vi "GUI2.vi"() -> ()   [LabVIEW 2023]
uses:
  <vilib>/userDefined/High Color/IMAQdx.ctl
  <vilib>/vision/Image Controls.llb/IMAQ Image.ctl
  <vilib>/vision/Avi.llb/IMAQ AVI2 Refnum.ctl
  Control2.ctl
  <vilib>/vision/driver/IMAQdx.llb/IMAQdx Acquisition Mode.ctl
  <vilib>/vision/driver/IMAQdx.llb/IMAQdx Buffer Number Mode.ctl
  <vilib>/Utility/error.llb/DialogType.ctl
  <vilib>/DAQmx/read.llb/DAQmx Read (Analog 1D Wfm NChan NSamp).vi
  <vilib>/DAQmx/write.llb/DAQmx Write (Analog 1D Wfm NChan NSamp).vi
  <extravilib>/ChannelInstances/Tag-bool/Read With Abort.vi
  <extravilib>/ChannelInstances/Stream-t'IMAQ Image.ctl'/Read With Abort.vi
  <extravilib>/ChannelInstances/Messenger-a[.](wfm(dbl))/Read With Abort.vi
  <extravilib>/ChannelInstances/Tag-str/Write With Abort.vi
  <extravilib>/ChannelInstances/Tag-c(bool,i32,str)/Read With Abort.vi
  <extravilib>/ChannelInstances/Messenger-c(bool,i32,str)/Write With Abort.vi
  <extravilib>/ChannelInstances/Messenger-a[.](wfm(dbl))/Write With Abort.vi
  <extravilib>/ChannelInstances/Messenger-c(bool,bool,bool,str,t'Rendezvous RefNum',bool)/Read With Abort.vi
  <extravilib>/ChannelInstances/Messenger-c(c(,,,bool),c(u16[NoSync,Sync],dbl,dbl,i32),str,ref(UserDefinedRefnumTag),c(path,str,u16[TDMS,CSV],str,bool))/Read With Abort.vi
  <extravilib>/ChannelInstances/Tag-bool/Write With Abort.vi
  <extravilib>/ChannelInstances/Messenger-c(bool,bool,bool,bool,t'Rendezvous RefNum',bool)/Write With Abort.vi
  <extravilib>/ChannelInstances/Messenger-c(c(str,i64,i64,str,str,t'IMAQdx.ctl'),c(i32,dbl,,,,str),c(dbl,str,str),c(i32,i32),i32,c(path,str,str,str,i32,str,i32,str))/Write With Abort.vi
  <extravilib>/ChannelInstances/Messenger-c(c(,,,bool),c(i32,i32,i32),str,c(path,str,u16[TDMS,CSV],str,bool))/Write With Abort.vi
  <extravilib>/ChannelInstances/Messenger-c(a[.](c(dbl,stamp,dbl)),bool,bool,bool,str,t'Rendezvous RefNum',bool)/Write With Abort.vi
  <extravilib>/ChannelInstances/Messenger-c(c(,,,bool),c(u16[NoSync,Sync],dbl,dbl,i32),str,ref(UserDefinedRefnumTag),c(path,str,u16[TDMS,CSV],str,bool))/Write With Abort.vi
  <extravilib>/ChannelInstances/Messenger-c(bool,bool,bool,str,t'Rendezvous RefNum',bool)/Write With Abort.vi
  <extravilib>/ChannelInstances/Tag-str/Read With Abort.vi
  <vilib>/Utility/High Resolution Relative Seconds.vi
  <extravilib>/ChannelInstances/Messenger-c(a[.](c(dbl,stamp,dbl)),bool,bool,bool,str,t'Rendezvous RefNum',bool)/Read With Abort.vi
  <extravilib>/ChannelInstances/Messenger-c(c(,,,bool),c(i32,i32,i32),str,c(path,str,u16[TDMS,CSV],str,bool))/Read With Abort.vi
  <extravilib>/ChannelInstances/Messenger-c(bool,i32,str)/Read With Abort.vi
  <extravilib>/ChannelInstances/Tag-c(bool,i32,str)/Write With Abort.vi
  <extravilib>/ChannelInstances/Messenger-c(bool,bool,bool,bool,t'Rendezvous RefNum',bool)/Read With Abort.vi
  <extravilib>/ChannelInstances/Messenger-c(c(str,i64,i64,str,str,t'IMAQdx.ctl'),c(i32,dbl,,,,str),c(dbl,str,str),c(i32,i32),i32,c(path,str,str,str,i32,str,i32,str))/Read With Abort.vi
  <extravilib>/ChannelInstances/Stream-t'IMAQ Image.ctl'/Write With Abort.vi
  <extravilib>/ChannelInstances/Stream-t'IMAQ Image.ctl'/EndpointRead.vi
  <extravilib>/ChannelInstances/Stream-t'IMAQ Image.ctl'/Endpoint.vi
  <extravilib>/ChannelInstances/Tag-bool/Instantiate.vi
  <extravilib>/ChannelInstances/Messenger-a[.](wfm(dbl))/Instantiate.vi
  <extravilib>/ChannelInstances/Messenger-c(bool,i32,str)/Instantiate.vi
  <vilib>/Utility/file.llb/Read Delimited Spreadsheet (DBL).vi
  TDMS File Initialization (Read).vi
  <vilib>/Utility/error.llb/Error Cluster From Error Code.vi
  <extravilib>/ChannelInstances/Tag-bool/EndpointRead.vi
  <extravilib>/ChannelInstances/Messenger-a[.](wfm(dbl))/Endpoint.vi
  <extravilib>/ChannelInstances/Tag-str/Instantiate.vi
  <extravilib>/ChannelInstances/Messenger-c(bool,bool,bool,str,t'Rendezvous RefNum',bool)/Instantiate.vi
  <extravilib>/ChannelInstances/Messenger-c(c(,,,bool),c(u16[NoSync,Sync],dbl,dbl,i32),str,ref(UserDefinedRefnumTag),c(path,str,u16[TDMS,CSV],str,bool))/Instantiate.vi
  <extravilib>/ChannelInstances/Messenger-c(a[.](c(dbl,stamp,dbl)),bool,bool,bool,str,t'Rendezvous RefNum',bool)/Instantiate.vi
  <extravilib>/ChannelInstances/Messenger-c(c(,,,bool),c(i32,i32,i32),str,c(path,str,u16[TDMS,CSV],str,bool))/Instantiate.vi
  <extravilib>/ChannelInstances/Messenger-c(bool,bool,bool,bool,t'Rendezvous RefNum',bool)/Instantiate.vi
  <extravilib>/ChannelInstances/Messenger-c(c(str,i64,i64,str,str,t'IMAQdx.ctl'),c(i32,dbl,,,,str),c(dbl,str,str),c(i32,i32),i32,c(path,str,str,str,i32,str,i32,str))/Instantiate.vi
  <extravilib>/ChannelInstances/Tag-bool/Endpoint.vi
  <extravilib>/ChannelInstances/Messenger-c(bool,bool,bool,bool,t'Rendezvous RefNum',bool)/Endpoint.vi
  <extravilib>/ChannelInstances/Messenger-c(c(str,i64,i64,str,str,t'IMAQdx.ctl'),c(i32,dbl,,,,str),c(dbl,str,str),c(i32,i32),i32,c(path,str,str,str,i32,str,i32,str))/Endpoint.vi
  <extravilib>/ChannelInstances/Messenger-c(c(,,,bool),c(i32,i32,i32),str,c(path,str,u16[TDMS,CSV],str,bool))/Endpoint.vi
  <extravilib>/ChannelInstances/Messenger-c(a[.](c(dbl,stamp,dbl)),bool,bool,bool,str,t'Rendezvous RefNum',bool)/Endpoint.vi
  <extravilib>/ChannelInstances/Messenger-c(c(,,,bool),c(u16[NoSync,Sync],dbl,dbl,i32),str,ref(UserDefinedRefnumTag),c(path,str,u16[TDMS,CSV],str,bool))/Endpoint.vi
  <extravilib>/ChannelInstances/Messenger-c(bool,bool,bool,str,t'Rendezvous RefNum',bool)/Endpoint.vi
  <extravilib>/ChannelInstances/Tag-str/EndpointRead.vi
  <extravilib>/ChannelInstances/Messenger-c(bool,i32,str)/Endpoint.vi
  <extravilib>/ChannelInstances/Tag-c(bool,i32,str)/Instantiate.vi
  <extravilib>/ChannelInstances/Tag-str/Endpoint.vi
  <vilib>/DAQmx/create/channels.llb/DAQmx Create Channel (AO-Voltage-Basic).vi
  <vilib>/DAQmx/configure/timing.llb/DAQmx Timing (Sample Clock).vi
  <vilib>/DAQmx/configure/trigger.llb/DAQmx Start Trigger (Digital Edge).vi
  <vilib>/Waveform/WDTFileIO.llb/Export Waveforms To Spreadsheet File (1D).vi
  <vilib>/DAQmx/miscellaneous.llb/DAQmx Fill In Error Info.vi
  <extravilib>/ChannelInstances/Tag-c(bool,i32,str)/EndpointRead.vi
  <vilib>/DAQmx/create/channels.llb/DAQmx Create Channel (AI-Voltage-Basic).vi
  <extravilib>/ChannelInstances/Tag-c(bool,i32,str)/Endpoint.vi
  <extravilib>/ChannelInstances/Stream-t'IMAQ Image.ctl'/Instantiate.vi
  <extravilib>/ChannelInstances/Stream-t'IMAQ Image.ctl'/)Channel.vi
  <resource>/ChannelSupport/_ChannelSupport/WaitIfNeeded.vi
  <vilib>/vision/EDVR.llb/IMAQ ImageToEDVR.vi
  <vilib>/vision/EDVR.llb/IMAQ ImageToEDVR 1D U8.vi
  <vilib>/vision/EDVR.llb/IMAQ ImageToEDVR 1D I16.vi
  <vilib>/vision/EDVR.llb/IMAQ ImageToEDVR 1D U32.vi
  <vilib>/vision/EDVR.llb/IMAQ ImageToEDVR 1D U16.vi
  <vilib>/Waveform/WDTOps.llb/WDT Append Waveforms DBL.vi
  <vilib>/Utility/file.llb/Write Delimited Spreadsheet (string).vi
  <vilib>/ErrorRing/Error Ring.xnode
  <vilib>/vision/driver/NI_Vision_Acquisition_Software.lvlib
  <resource>/objmgr/imaqdx.rc
  <extravilib>/ChannelInstances/Messenger-c(bool,i32,str).lvlib
  <extravilib>/ChannelInstances/Tag-c(bool,i32,str).lvlib
  <extravilib>/ChannelInstances/Tag-bool.lvlib
  <resource>/objmgr/daqmx.rc
  <extravilib>/ChannelInstances/Stream-t'IMAQ Image.ctl'.lvlib
  <extravilib>/ChannelInstances/Tag-str.lvlib
  <extravilib>/ChannelInstances/Messenger-c(bool,bool,bool,bool,t'Rendezvous RefNum',bool).lvlib
  <extravilib>/ChannelInstances/Messenger-c(a[.](c(dbl,stamp,dbl)),bool,bool,bool,str,t'Rendezvous RefNum',bool).lvlib
  <extravilib>/ChannelInstances/Messenger-c(bool,bool,bool,str,t'Rendezvous RefNum',bool).lvlib
  <extravilib>/ChannelInstances/Messenger-a[.](wfm(dbl)).lvlib
  <extravilib>/ChannelInstances/Messenger-c(c(,,,bool),c(i32,i32,i32),str,c(path,str,u16[TDMS,CSV],str,bool)).lvlib
  <extravilib>/ChannelInstances/Messenger-c(c(,,,bool),c(u16[NoSync,Sync],dbl,dbl,i32),str,ref(UserDefinedRefnumTag),c(path,str,u16[TDMS,CSV],str,bool)).lvlib
  <extravilib>/ChannelInstances/Messenger-c(c(str,i64,i64,str,str,t'IMAQdx.ctl'),c(i32,dbl,,,,str),c(dbl,str,str),c(i32,i32),i32,c(path,str,str,str,i32,str,i32,str)).lvlib
  <vilib>/measure/NI_MABase.lvlib
panel:
  out "Sensor Readout Time":dbl
  out "Max FPS":dbl
  out "FPS":dbl
  out "Images Behind":dbl
  out "Missed Images":dbl
  out "Video Bytes/s":dbl
  out "Estimated Time":dbl
  out "FPS 2":dbl
  out "Images Behind 2":dbl
  out "Missed Images 2":dbl
  out "Estimated Time 2":dbl
  out "Array 2":string[](array[string])
  out "Array":string[](array[string])
  in  "CameraPane Selector":u16(ring) items=["None", "CameraDisplay", "Plot1", "Plot2", "Plot3", "Plot4", "XY1", "XY2"]
  in  "Experiment Name":string="VoltageTest"
  in  "Save Path":path
  in  "Save Config":bool
  in  "Apply Configuration":bool
  in  "Config Path":path
  in  "Initialize from config file?":bool caption="Checkbox"
  in  "Quit":bool
  in  "Controls":bool
  in  "File Manager":bool
  in  "Settings":bool
  in  "Camera Setup":bool
  in  "MainTabControl":T1(tab)
  in  "Stop Square":bool
  in  "Initialize Camera":bool
  in  "Cluster - Borderless":T3={"Cluster - Borderless"={"Time Stamp\n Position"=enum."Exposure Center", "Synchronize Camera and Data"=TRUE}, "Sensor readout mode\n(Fast Decreases Quality)"=0, "Pixel Format\n(p not supported)"=0, "Gain"=0.0, "Gamma"=1.0, "Temporary Format\n(can be converted)"=enum."AVI", "Cluster - Borderless 2"={"Frame Limit"=0.0}, "Cluster - Borderless 3"={"Frame Limit"=0.0}, "Camera Ref"="", "Tempory Storage Location\n(File can be moved after acquisition)\nSSD recomended for high frame rate"=path "E:/Jacob", "Images Per File"=1000000.0, "Buffer Images"=1000.0, "Exposure (us)"=100.0, "FPS"=30.0, "Encoding Quality"=-1.0, "Image Width"=0.0, "Image Height"=0.0, "Signal Line"=2, "Codec"=2, "Confirm File Write Optimizations (TDMS)"=TRUE, "Confirm Disable Buffering (advanced TDMS)"=FALSE, "Camera Signal Output Port"="/Dev1/PFI2", "Exposure Mode"=0, "Video File Suffix"="Video", "Timing File Suffix"="VideoTime", "Include Camera Signal Output File"=FALSE, "File Time Resolution (s)"=0.0, "Stop Acquisition on Full Buffer"=TRUE} {"Exposure Mode" items=["Standard", "Ultra Short"]; "Codec" items=["(Select at runtime)", "YUV 4:2:0 Planar (NI Vision)", "Y800 Uncompressed Grey Scale (NI Vision)", "VP9 (NI Vision)", "Motion JPEG (NI Vision)", "FF Video Codec 1 (FFV1) (NI Vision)", "VP8 (NI Vision)"]; "Signal Line" items=["Software", "Line 1", "Line 3", "Line 4", "Software Signal 1", "Software Signal 2", "Software Signal 3"]; "Gamma" min=0.0 max=4.0 step=1.0 scale=0.0..3.0; "Gain" min=0.0 max=12.0092 step=1.0 scale=0.0..12.0; "Pixel Format\n(p not supported)" items=["Mono 8", "Mono 10"]; "Sensor readout mode\n(Fast Decreases Quality)" items=["Normal", "Fast"]}
  in  "Stop Acquisition On Full Hard Drive":bool=TRUE caption="Checkbox"
  in  "XY2 Y":u16(ring) items=["None", "Current (mA)", "Voltage (V)"]
  in  "XY2 X":u16(ring) items=["None", "Current (mA)", "Voltage (V)"]
  in  "XY1 Y":u16(ring) items=["None", "Current (mA)", "Voltage (V)"]
  in  "XY1 X":u16(ring) items=["None", "Current (mA)", "Voltage (V)"]
  in  "Data File Settings":T4={"Data File Format"=FALSE, "Data Temporary Storage Location"=path "E:/Jacob", "Temporary Location"=TRUE, "Input Data File Suffix"="Data", "Output Data File Suffix"="DataOutput", "              CSV\nMultiple Time Columns"=FALSE}
  in  "Plot 4 Channels":i32[](listbox)
  in  "Plot 3 Channels":i32[](listbox)
  in  "Plot 2 Channels":i32[](listbox)
  in  "Plot 1 Channels":i32[](listbox)
  in  "Samples to Generate":dbl=1000.0
  out "1D Array":string[](array[string])
  in  "Channel Names":string[](array[string])
  in  "Sample Buffer":dbl=1000.0
  in  "Sample Rate":dbl=10000.0
  in  "Input Channels":tag
  in  "Voltage Input Channel":tag
  in  "Current Input Channel":tag
  in  "Using Gamry Potentiostat":bool caption="Checkbox"
  in  "Recipients":string
  in  "Send email on non-user-initiated stop":bool
  out "Shutting\nDown":bool
  out "Video Space Remaining (min)":dbl
  out "Data Space Remaining (min)":dbl
  out "Video Buffer Fill Percent":dbl(slide) scale=0.0..100.0
  in  "Stop Button":bool
  in  "Use Camera":bool
  in  "FPS":dbl=150.0
  in  "Save Video":bool
  in  "Initialize Camera":bool
  in  "Outputs":T5={"AO0"={"signal type"=enum."Sine Wave", "Frequency"=0.0, "Amplitude"=0.0, "Offset"=0.0, "Phase"=0.0, "Duty Cycle"=0.0}, "AO0Enable"=FALSE, "AO1"={"signal type"=enum."Sine Wave", "Frequency"=0.0, "Amplitude"=0.0, "Offset"=0.0, "Phase"=0.0, "Duty Cycle"=0.0}, "AO1Enable"=FALSE, "AO2"={"signal type"=enum."Sine Wave", "Frequency"=0.0, "Amplitude"=0.0, "Offset"=0.0, "Phase"=0.0, "Duty Cycle"=0.0}, "AO3Enable"=FALSE, "AO0Name"="Ao0", "AO1Name"="Ao1", "AO2Name"="Ao2"}
  in  "Re/Start Acquisition":bool
  in  "Exposure (us)":dbl
  in  "Update Viewport Every N Frames":dbl=1.0
  in  "PlotSelector":T6(tab)
  in  "OneSelection":u16(ring) items=["None", "CameraDisplay", "Plot1", "Plot2", "Plot3", "Plot4", "XY1", "XY2"]
  in  "TwoVertSelL":u16(ring) items=["None", "CameraDisplay", "Plot1", "Plot2", "Plot3", "Plot4", "XY1", "XY2"]
  in  "TwoVertSelR":u16(ring) items=["None", "CameraDisplay", "Plot1", "Plot2", "Plot3", "Plot4", "XY1", "XY2"]
  in  "2HorizSelB":u16(ring) items=["None", "CameraDisplay", "Plot1", "Plot2", "Plot3", "Plot4", "XY1", "XY2"]
  in  "2HorizSelT":u16(ring) items=["None", "CameraDisplay", "Plot1", "Plot2", "Plot3", "Plot4", "XY1", "XY2"]
  in  "3PaneVertSelBR":u16(ring) items=["None", "CameraDisplay", "Plot1", "Plot2", "Plot3", "Plot4", "XY1", "XY2"]
  in  "3PaneVertSelTR":u16(ring) items=["None", "CameraDisplay", "Plot1", "Plot2", "Plot3", "Plot4", "XY1", "XY2"]
  in  "3PaneVertSelL":u16(ring) items=["None", "CameraDisplay", "Plot1", "Plot2", "Plot3", "Plot4", "XY1", "XY2"]
  in  "3PaneHorizBL":u16(ring) items=["None", "CameraDisplay", "Plot1", "Plot2", "Plot3", "Plot4", "XY1", "XY2"]
  in  "3PaneHorizBR":u16(ring) items=["None", "CameraDisplay", "Plot1", "Plot2", "Plot3", "Plot4", "XY1", "XY2"]
  in  "3PaneHorizT":u16(ring) items=["None", "CameraDisplay", "Plot1", "Plot2", "Plot3", "Plot4", "XY1", "XY2"]
  in  "4PaneSelBR":u16(ring) items=["None", "CameraDisplay", "Plot1", "Plot2", "Plot3", "Plot4", "XY1", "XY2"]
  in  "4PaneSelBL":u16(ring) items=["None", "CameraDisplay", "Plot1", "Plot2", "Plot3", "Plot4", "XY1", "XY2"]
  in  "4PaneSelTR":u16(ring) items=["None", "CameraDisplay", "Plot1", "Plot2", "Plot3", "Plot4", "XY1", "XY2"]
  in  "4PaneSelTL":u16(ring) items=["None", "CameraDisplay", "Plot1", "Plot2", "Plot3", "Plot4", "XY1", "XY2"]
  out "Plot Overflow":i32
  out "Actual Sample Rate":dbl
  out "Images Missed":u32
  out "Processing Speed (ms)":dbl format="%_19f"
  out "Write Speed (ms)":dbl format="%_19f"
  out "BufferWasFull":bool
  out "Files Complete":i32(slide)=1 max=4 scale=0.0..4.0
  in  "Start Button":bool
  in  "Codec":u16(ring)=2 items=["(Select at runtime)", "YUV 4:2:0 Planar (NI Vision)", "Y800 Uncompressed Grey Scale (NI Vision)", "VP9 (NI Vision)", "Motion JPEG (NI Vision)", "FF Video Codec 1 (FFV1) (NI Vision)", "VP8 (NI Vision)"]
  in  "Quality":dbl=-1.0
  in  "Same as previous":bool=TRUE caption="Checkbox"
  in  "Timing File":path=path "E:/Jacob"
  in  "AVI FPS":dbl=30.0
  in  "Same as acquisition":bool caption="Checkbox"
  in  "Save Name":string
  in  "Save Path":path=path "E:/Jacob"
  in  "Combine Split Videos":bool caption="Checkbox"
  in  "First Video File":path=path "E:/Jacob"
  in  "Current Image Type":u16(ring) items=["Grayscale (U8)"=0, "Grayscale (I16)"=1, "Grayscale (U16)"=7, "RGB Color (U32)"=4]
  in  "Stop Conversion":bool
  out "File Percent Done":dbl(slide) scale=0.0..1.0
  # "Basic Camera Controls"
  # "Camera"
  # "Image Aquisition Settings"
  # "Video File Settings"
  # "Do not use \"_\""
  # "This may cause memory issues"
  # "Advanced Settings"
  # "Advanced File Settings"
  # "(Must be multiple of 64)"
  # "AVI Settings"
  # "If very high framerates are required, save to TDMS not AVI\nFor high framerates Y800 is recomended, but requires\ncompression later to save space\nFor lower framerates, Motion JPEG saves \nspace and conversion time"
  # "For further advanced setting changes (binning,\netc.) open NI Max, select the camera, and change\nthe desired properties, pressing save at the end.\n\n(Note: This program may overwrite settings\ntemporarily while running in order to function)"
  # "(1-1000) or -1 for highest"
  # "Hardware Triggered\nAcquisition Settings"
  # "Use shift or ctrl to select multiple channels for each plot"
  # "XY Plots not yet implemented"
  # "If the data generation estimate does not line up with the measured value, consider increasing the buffer,\nthis allows software processing without interupting sample generation/aquisition.\nIt is highly recomended to measure the generated output instead of relying on just the estimate, since there might be\nartifacts generated by processing, especially near the beginning.\nHaving too small a buffer compared to samples to generate \ncan cause blips in the signal generation when interacting with the software. Leaving a sufficient number of ms\nfor software to work is recomended.\nIf working with an important experiment, it is recomended to minimize interaction to ensure sample generation\nis what is desired.\n\nIf the plot update is too slugish, consider decreasing the buffer.\nHowever, decreasing the buffer decreases ability of plot to keep up with supplied data."
  # "This should be lower than the sample rate"
  # "(Output Only)"
  # "This should be at least 2x higher than the sample buffer"
  # "TDMS may be faster (Can be converted later)"
  # "Writing to CSV can be very slow \nuse only for small data rates with minimal channels\n\nIf time accuracy is required within 10 us, \nuse multiple time columns"
  # "(Needs Reset)"
  # "Does not save video"
  # "TDMS Video Conversion"
  # "Requires timing file"
  # "(1-1000) or -1 for highest"
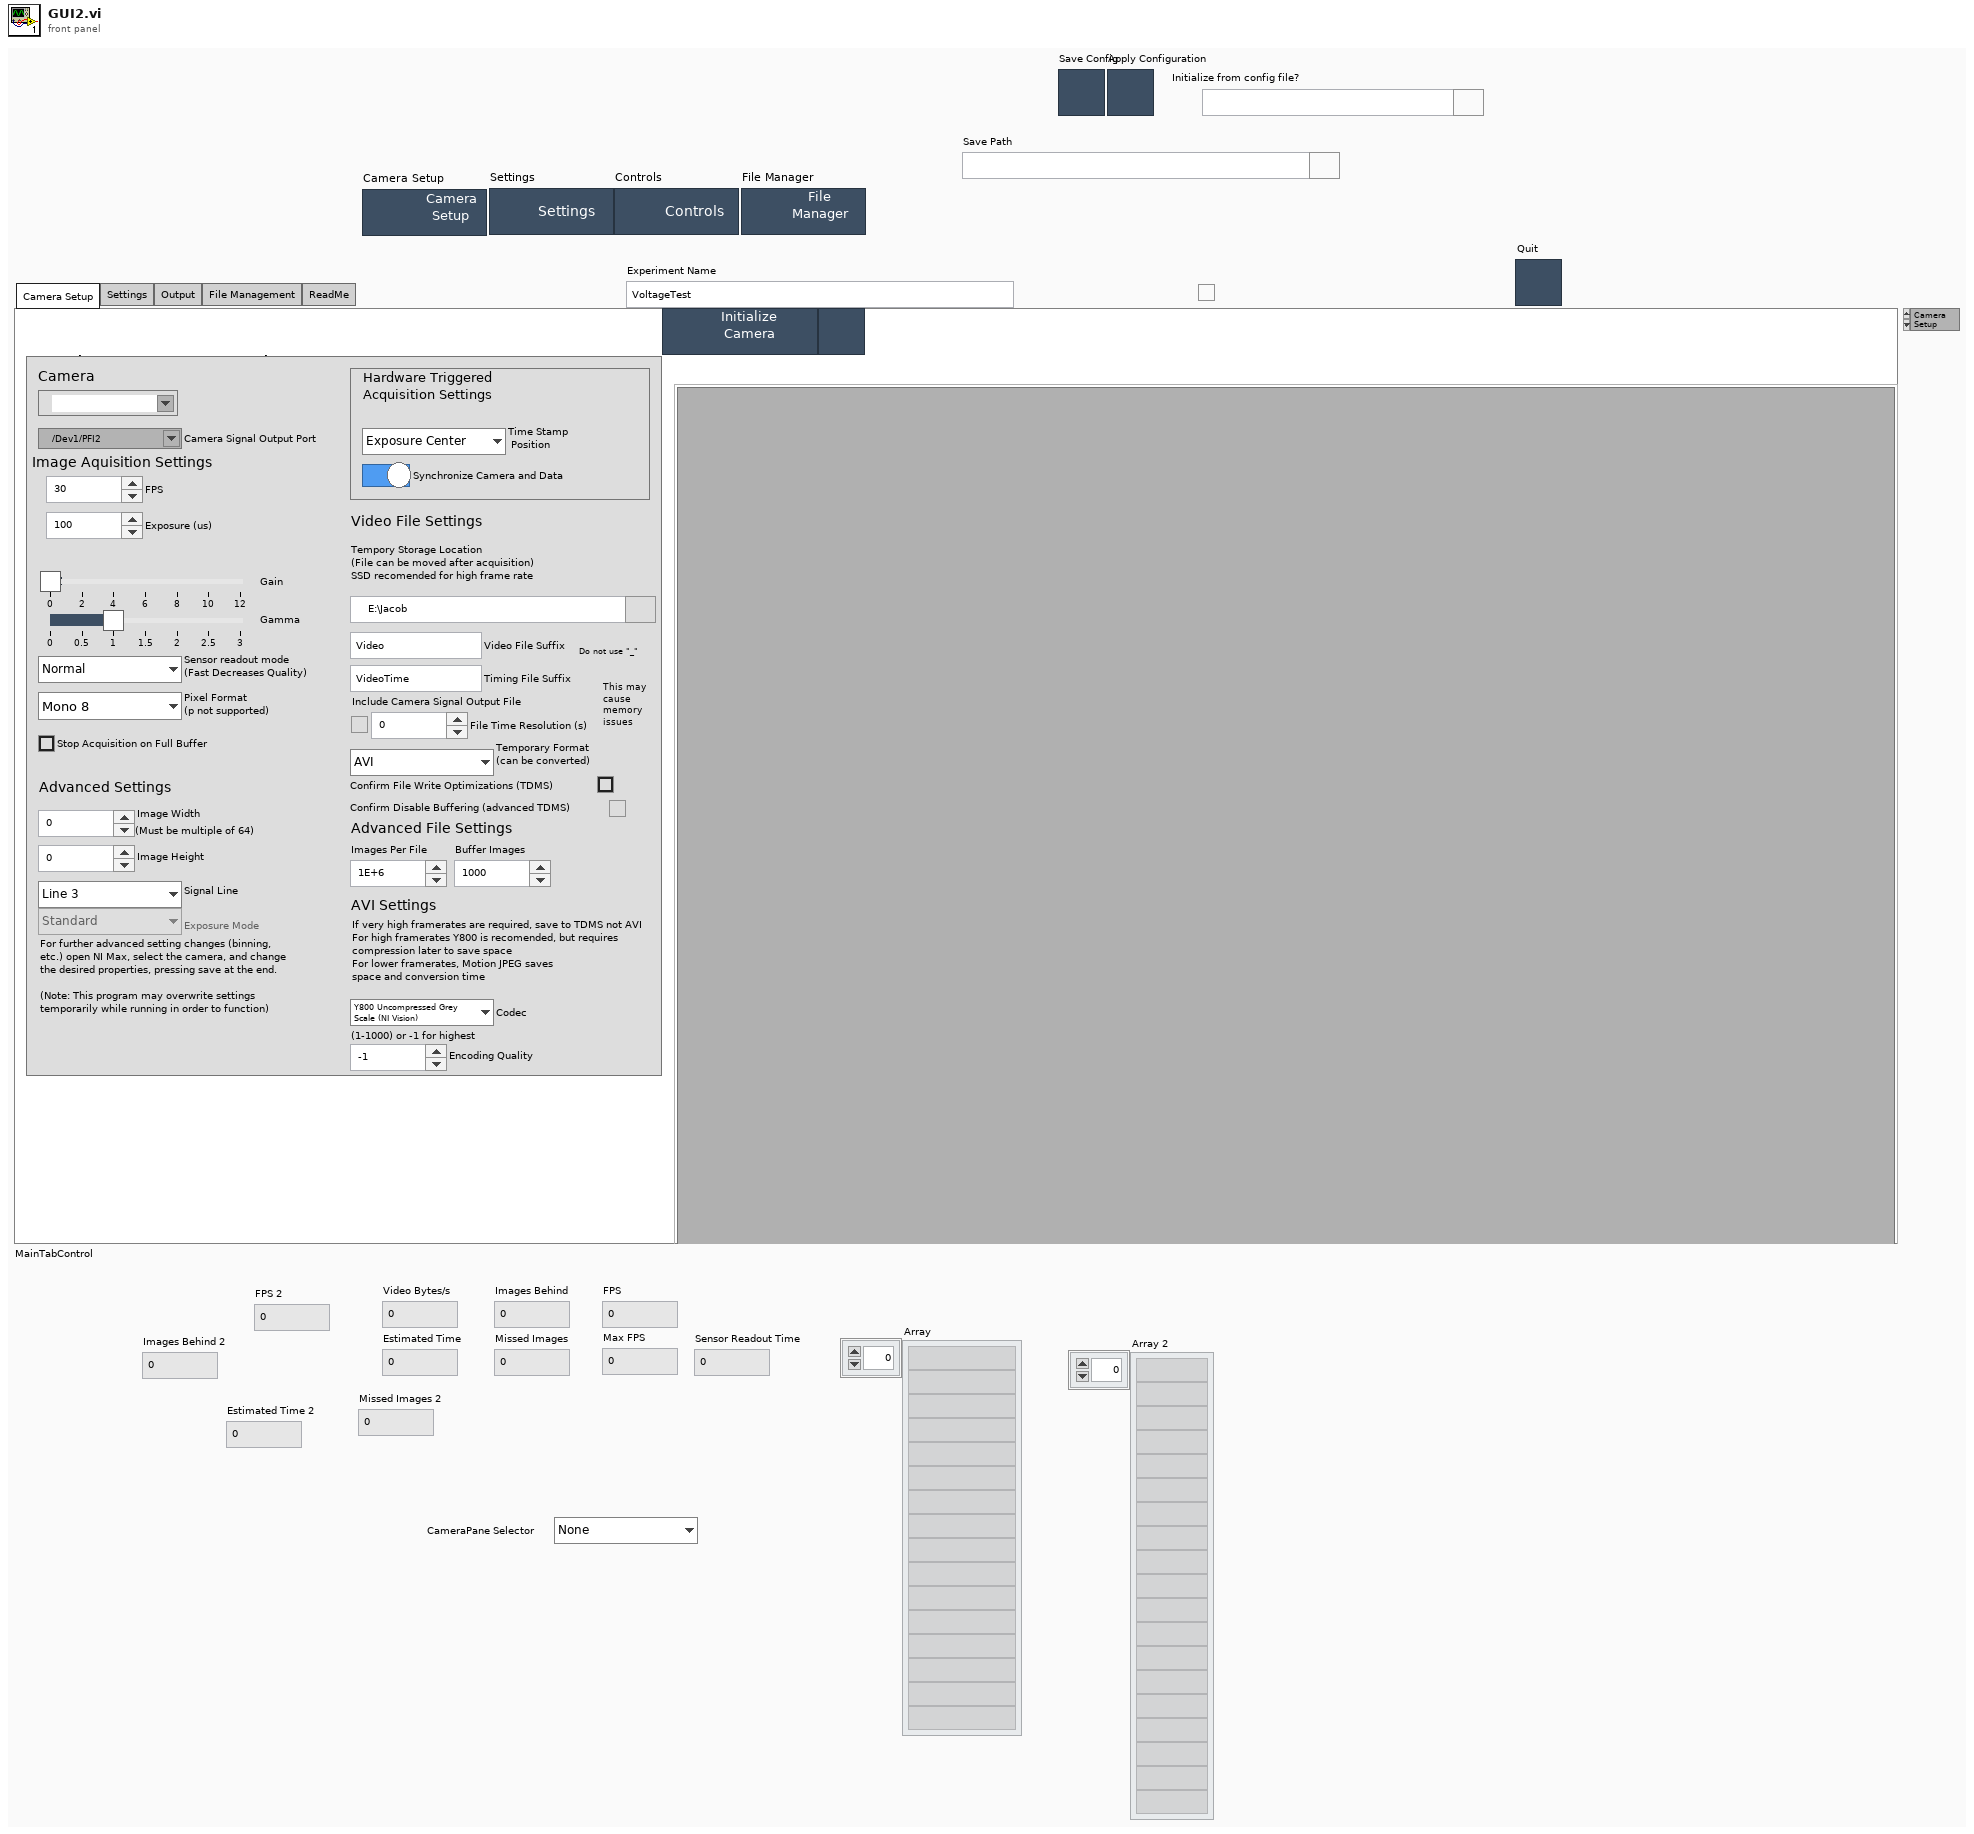
[diagram p1: front panel]
types:
  T1 = enum32{"Camera Setup", "Settings", "Output", "File Management", "ReadMe"}
  T2 = typedef "IMAQdx.ctl" = refnum<k21>
  T3 = cluster{"Cluster - Borderless":cluster{"Time Stamp\n Position":enum16{"Exposure Center", "Exposure Beginning", "Exposure End"}, "Synchronize Camera and Data":bool}, "Sensor readout mode\n(Fast Decreases Quality)":u16, "Pixel Format\n(p not supported)":u16, "Gain":dbl, "Gamma":dbl, "Temporary Format\n(can be converted)":enum16{"AVI", "TDMS", "None"}, "Cluster - Borderless 2":cluster{"Frame Limit":dbl}, "Cluster - Borderless 3":cluster{"Frame Limit":dbl}, "Camera Ref":T2, "Tempory Storage Location\n(File can be moved after acquisition)\nSSD recomended for high frame rate":path, "Images Per File":dbl, "Buffer Images":dbl, "Exposure (us)":dbl, "FPS":dbl, "Encoding Quality":dbl, "Image Width":dbl, "Image Height":dbl, "Signal Line":u16, "Codec":u16, "Confirm File Write Optimizations (TDMS)":bool, "Confirm Disable Buffering (advanced TDMS)":bool, "Camera Signal Output Port":tag, "Exposure Mode":u16, "Video File Suffix":string, "Timing File Suffix":string, "Include Camera Signal Output File":bool, "File Time Resolution (s)":dbl, "Stop Acquisition on Full Buffer":bool}
  T4 = cluster{"Data File Format":bool, "Data Temporary Storage Location":path, "Temporary Location":bool, "Input Data File Suffix":string, "Output Data File Suffix":string, "              CSV\nMultiple Time Columns":bool}
  T5 = cluster{"AO0":cluster{"signal type":enum16{"Sine Wave", "Triangle Wave", "Square Wave", "Sawtooth Wave"}, "Frequency":dbl, "Amplitude":dbl, "Offset":dbl, "Phase":dbl, "Duty Cycle":dbl}, "AO0Enable":bool, "AO1":cluster{"signal type":enum16{"Sine Wave", "Triangle Wave", "Square Wave", "Sawtooth Wave"}, "Frequency":dbl, "Amplitude":dbl, "Offset":dbl, "Phase":dbl, "Duty Cycle":dbl}, "AO1Enable":bool, "AO2":cluster{"signal type":enum16{"Sine Wave", "Triangle Wave", "Square Wave", "Sawtooth Wave"}, "Frequency":dbl, "Amplitude":dbl, "Offset":dbl, "Phase":dbl, "Duty Cycle":dbl}, "AO3Enable":bool, "AO0Name":string, "AO1Name":string, "AO2Name":string}
  T6 = enum32{"One Pane", "2 Vertical Panes", "2 Horizontal Panes", "3 Panes Vert", "3 Panes Horiz", "Four Panes"}
  T7 = typedef "Rendezvous RefNum" = refnum<k1>
  T8 = cluster{"Use Camera":bool, "Use Inputs":bool, "Use Outputs":bool, "rendezvous":T7, "Save Video":bool, "VideoPath":path, "DataPath":path, "Acquiring":bool, "LastSizeVid":dbl, "Last Time":dbl, "LastSizeData":dbl, "StopMessage":string, "Description":string, "Post Notes":string, "StopDueToError":bool}
  T9 = cluster{"SyncStart":bool, "Leader":bool, "Started?":bool, "AfterErrorCheck":string, "rendezvous ref":T7, "AcStarted":bool, "FirstAq":bool, "t0":timestamp, "TDMSRef":refnum<k34>, "CSV path":path}
  T10 = cluster{"Physical Settings":cluster{"physical channels":tag, "source":tag, "Start Trigger":tag, "StartTriggered":bool}, "Acquisition Settings":cluster{"SyncType":enum16{"NoSync", "Sync"}, "Frame Rate":dbl, "Sample Rate":dbl, "Sample BufferSize":i32}, "Channel Names":string, "task in":refnum<k21>, "FileSettings":cluster{"Path":path, "File":string, "FileFormat":enum16{"TDMS", "CSV"}, "FileSuffix":string, "Multiple Time Columns":bool}}
  T11 = cluster{"DefaultAction":string, "NextAction":string, "ActionString":string}
  T12 = typedef "Control2.ctl" = cluster{"SubPanel":refnum<vi>, "Selector":refnum<vi>}
  T13 = cluster{"One Pane":cluster{"Panel2":cluster{"SubPanel":refnum<vi>, "Selector":refnum<vi>}, "Panel3":cluster{"SubPanel":refnum<vi>, "Selector":refnum<vi>}, "Panel4":cluster{"SubPanel":refnum<vi>, "Selector":refnum<vi>}, "Panel1":T12}, "2 Vertical Panes":cluster{"Panel2":cluster{"SubPanel":refnum<vi>, "Selector":refnum<vi>}, "Panel3":cluster{"SubPanel":refnum<vi>, "Selector":refnum<vi>}, "Panel4":cluster{"SubPanel":refnum<vi>, "Selector":refnum<vi>}, "Panel1":T12}, "2 Horizontal Panes":cluster{"Panel2":cluster{"SubPanel":refnum<vi>, "Selector":refnum<vi>}, "Panel3":cluster{"SubPanel":refnum<vi>, "Selector":refnum<vi>}, "Panel4":cluster{"SubPanel":refnum<vi>, "Selector":refnum<vi>}, "Panel1":T12}, "3 Panes Vert":cluster{"Panel2":cluster{"SubPanel":refnum<vi>, "Selector":refnum<vi>}, "Panel3":cluster{"SubPanel":refnum<vi>, "Selector":refnum<vi>}, "Panel4":cluster{"SubPanel":refnum<vi>, "Selector":refnum<vi>}, "Panel1":T12}, "3 Panes Horiz":cluster{"Panel2":cluster{"SubPanel":refnum<vi>, "Selector":refnum<vi>}, "Panel3":cluster{"SubPanel":refnum<vi>, "Selector":refnum<vi>}, "Panel4":cluster{"SubPanel":refnum<vi>, "Selector":refnum<vi>}, "Panel1":T12}, "Four Panes":cluster{"Panel2":cluster{"SubPanel":refnum<vi>, "Selector":refnum<vi>}, "Panel3":cluster{"SubPanel":refnum<vi>, "Selector":refnum<vi>}, "Panel4":cluster{"SubPanel":refnum<vi>, "Selector":refnum<vi>}, "Panel1":T12}, "Camera Pane":cluster{"Panel2":cluster{"SubPanel":refnum<vi>, "Selector":refnum<vi>}, "Panel3":cluster{"SubPanel":refnum<vi>, "Selector":refnum<vi>}, "Panel4":cluster{"SubPanel":refnum<vi>, "Selector":refnum<vi>}, "Panel1":T12}}
  T14 = cluster{"Panel2":cluster{"SubPanel":refnum<vi>, "Selector":refnum<vi>}, "Panel3":cluster{"SubPanel":refnum<vi>, "Selector":refnum<vi>}, "Panel4":cluster{"SubPanel":refnum<vi>, "Selector":refnum<vi>}, "Panel1":T12}
  T15 = cluster{"PreviousInfo":cluster{"FinalSamplePhase":dbl, "LastTf":timestamp, "LastSelectedPhase":dbl}[], "SyncStart":bool, "Leader":bool, "Started?":bool, "AfterErrorCheck":string, "rendezvous ref ":T7, "AcStarted":bool, "PrevousWave":waveform(dbl)[], "TDMSRef":refnum<k34>, "CSV path":path}
  T16 = cluster{"Physical Settings":cluster{"physical channels":tag, "source":tag, "Start Trigger":tag, "StartTriggered":bool}, "OutputTask":refnum<k21>, "GenerationSettings":cluster{"NumberOfSamples":i32, "Sample Rate":i32, "SampleBuffer":i32}, "Channel Names":string, "FileSettings":cluster{"Path":path, "File":string, "FileFormat":enum16{"TDMS", "CSV"}, "FileSuffix":string, "Multiple Time Columns":bool}}
  T17 = cluster{"SyncStart":bool, "AfterErrorCheck":string, "VideoPath":path, "ConfirmTDMSOptimizations":bool, "ConfirmTDMSDisableBuffer":bool, "CameraOpen":bool, "TriggerStarted":bool, "AcquisitionStarted":bool, "FileOpen":bool, "VideoSave":bool, "BufferOpen":bool, "ShutdownActions":string[], "Acquisition Configured":bool, "rendezvous ref ":T7, "ResetAq?":bool, "AcStarted":bool, "Frames":i32}
  T18 = typedef "IMAQ Image.ctl" = refnum<image>
  T19 = typedef "IMAQ AVI2 Refnum.ctl" = refnum<k20>
  T20 = typedef "Image Type" = u32
  T21 = cluster{"User Camera Settings":cluster{"Pixel Format":string, "Width":i64, "Height":i64, "Trigger Source":string, "Readout Mode":string, "Session In":T2}, "IMAQdx Session":T2, "Camera Aq Attributes":cluster{"Readout Time":dbl, "Resulting FPS":dbl, "Width":u32, "Height":u32, "Format":u32, "Bit Depth":u32}, "Camera Attributes":cluster{"Exposure Start Delay":dbl, "Model":string, "Make":string}, "AcquisitionSettings":cluster{"Buffer":i32, "FramesPerFile":i32}, "Image Buffer":T18[], "Example Image":T18, "AVIRef":T19, "TDMSRef":refnum<k34>, "TDMSWSet":cluster{"Image Type":T20, "Async File Format":bool}, "CameraSignalRefnum":refnum<k21>, "CameraSignalDefinition":cluster{"High Time":dbl, "Low Time":dbl, "Delay":dbl}, "DisplayEveryNFrames":i32, "Trigger Settings":cluster{"FPS":i32, "Exposure Time":dbl, "Start Trigger Source":tag, "Camera\nClock\nCounter":tag, "PhysicalCameraSignalLine":tag, "Sync Type":string}, "FileSettings":cluster{"FileSaveLocation":path, "FileName":string, "VideoSuffix":string, "Codec":string, "Quality":i32, "Format":string, "AVI FPS":i32, "TimingSuffix":string}}
  T22 = enum8{"Enabled", "Disabled", "Disabled and Grayed Out"}
  T23 = enum16{"open", "replace", "create", "open or create", "replace or create", "replace or create with confirmation"}
  T24 = cluster{"User Camera Settings":cluster{"Pixel Format":string, "Width":i64, "Height":i64, "Trigger Source":string, "Readout Mode":string, "Session In":T2}, "Trigger Settings":cluster{"FPS":i32, "Exposure Time":dbl, "Start Trigger Source":tag, "Camera\nClock\nCounter":tag, "PhysicalCameraSignalLine":tag, "Sync Type":string}, "Camera Attributes":cluster{"Exposure Start Delay":dbl, "Model":string, "Make":string}, "AcquisitionSettings":cluster{"Buffer":i32, "FramesPerFile":i32}, "DisplayEveryNFrames":i32, "FileSettings":cluster{"FileSaveLocation":path, "FileName":string, "VideoSuffix":string, "Codec":string, "Quality":i32, "Format":string, "AVI FPS":i32, "TimingSuffix":string}}
  T25 = enum16{"Exposure End", "Exposure Center", "Exposure Start", "Start", "NoSync"}
  T26 = cluster{"Physical Settings":cluster{"physical channels":tag, "source":tag, "Start Trigger":tag, "StartTriggered":bool}, "GenerationSettings":cluster{"NumberOfSamples":i32, "Sample Rate":i32, "SampleBuffer":i32}, "Channel Names":string, "FileSettings":cluster{"Path":path, "File":string, "FileFormat":enum16{"TDMS", "CSV"}, "FileSuffix":string, "Multiple Time Columns":bool}}
  T27 = typedef "Tag-bool.lvlib/))Channel.ctl" = refnum<queue>
  T28 = cluster{"Panel2":cluster{"SubPanel":refnum<vi>, "Selector":refnum<vi>}, "Panel3":cluster{"SubPanel":refnum<vi>, "Selector":refnum<vi>}, "Panel4":cluster{"SubPanel":refnum<vi>, "Selector":refnum<vi>}, "Panel1":T12}[]
  T29 = cluster{"SubPanel":refnum<vi>, "Selector":refnum<vi>}
  T30 = cluster{"FPS":i32, "Exposure Time":dbl, "Start Trigger Source":tag, "Camera\nClock\nCounter":tag, "PhysicalCameraSignalLine":tag, "Sync Type":string}
  T31 = cluster{"SyncStart":bool, "ConfirmTDMSOptimizations":bool, "ConfirmTDMSDisableBuffer":bool, "VideoSave":bool, "rendezvous ref ":T7, "AcStarted":bool}
  T32 = cluster{"FileSaveLocation":path, "FileName":string, "VideoSuffix":string, "Codec":string, "Quality":i32, "Format":string, "AVI FPS":i32, "TimingSuffix":string}
  T33 = cluster{"Pixel Format":string, "Width":i64, "Height":i64, "Trigger Source":string, "Readout Mode":string, "Session In":T2}
  T34 = typedef "Messenger-c(bool,bool,bool,bool,t'Rendezvous RefNum',bool).lvlib/))Channel.ctl" = refnum<queue>
  T35 = typedef "Messenger-c(c(str,i64,i64,str,str,t'IMAQdx.ctl'),c(i32,dbl,,,,str),c(dbl,str,str),c(i32,i32),i32,c(path,str,str,str,i32,str,i32,str)).lvlib/))Channel.ctl" = refnum<queue>
  T36 = cluster{"Path":path, "File":string, "FileFormat":enum16{"TDMS", "CSV"}, "FileSuffix":string, "Multiple Time Columns":bool}
  T37 = cluster{"PreviousInfo":cluster{"FinalSamplePhase":dbl, "LastTf":timestamp, "LastSelectedPhase":dbl}[], "SyncStart":bool, "Leader":bool, "Started?":bool, "AfterErrorCheck":string, "rendezvous ref ":T7, "AcStarted":bool}
  T38 = cluster{"physical channels":tag, "source":tag, "Start Trigger":tag, "StartTriggered":bool}
  T39 = cluster{"NumberOfSamples":i32, "Sample Rate":i32, "SampleBuffer":i32}
  T40 = typedef "Messenger-c(c(,,,bool),c(i32,i32,i32),str,c(path,str,u16[TDMS,CSV],str,bool)).lvlib/))Channel.ctl" = refnum<queue>
  T41 = typedef "Messenger-c(a[.](c(dbl,stamp,dbl)),bool,bool,bool,str,t'Rendezvous RefNum',bool).lvlib/))Channel.ctl" = refnum<queue>
  T42 = cluster{"SyncStart":bool, "Leader":bool, "Started?":bool, "AfterErrorCheck":string, "rendezvous ref":T7, "AcStarted":bool}
  T43 = cluster{"SyncType":enum16{"NoSync", "Sync"}, "Frame Rate":dbl, "Sample Rate":dbl, "Sample BufferSize":i32}
  T44 = typedef "Messenger-c(c(,,,bool),c(u16[NoSync,Sync],dbl,dbl,i32),str,ref(UserDefinedRefnumTag),c(path,str,u16[TDMS,CSV],str,bool)).lvlib/))Channel.ctl" = refnum<queue>
  T45 = typedef "Messenger-c(bool,bool,bool,str,t'Rendezvous RefNum',bool).lvlib/))Channel.ctl" = refnum<queue>
  T46 = typedef "Messenger-c(bool,i32,str).lvlib/))Channel.ctl" = refnum<queue>
  T47 = typedef "Tag-c(bool,i32,str).lvlib/))Channel.ctl" = refnum<queue>
  T48 = enum16{"open", "open or create", "create or replace", "create", "open (read-only)"}
  T49 = typedef "Tag-str.lvlib/))Channel.ctl" = refnum<queue>
  T50 = typedef "Messenger-a[.](wfm(dbl)).lvlib/))Channel.ctl" = refnum<queue>
  T51 = typedef "NI_Vision_Acquisition_Software.lvlib/IMAQdx Acquisition Mode.ctl" = enum32{"One Shot", "Continuous"}
  T52 = typedef "NI_Vision_Acquisition_Software.lvlib/IMAQdx Buffer Number Mode.ctl" = enum32{"Next", "Last", "Buffer Number", "Every", "Last New"}
  T53 = cluster{"Exposure Start Delay":dbl, "Model":string, "Make":string}
  T54 = cluster{"Readout Time":dbl, "Resulting FPS":dbl, "Width":u32, "Height":u32, "Format":u32, "Bit Depth":u32}
  T55 = cluster{"Image Type":T20, "Async File Format":bool}
  T56 = cluster{"Asynchronous Writes":bool, "Reserve Disk Space":bool, "Disable Buffering":bool}
  T57 = cluster{"High Time":dbl, "Low Time":dbl, "Delay":dbl}
  T58 = typedef "DialogType.ctl" = u16
  T59 = typedef "Stream-t'IMAQ Image.ctl'.lvlib/)Channel.ctl" = refnum<queue>
  T60 = cluster{"FinalSamplePhase":dbl, "LastTf":timestamp, "LastSelectedPhase":dbl}[]
  T61 = cluster{"AO0":cluster{"signal type":enum16{"Sine Wave", "Triangle Wave", "Square Wave", "Sawtooth Wave"}, "Frequency":dbl, "Amplitude":dbl, "Offset":dbl, "Phase":dbl, "Duty Cycle":dbl}, "AO0Enable":bool, "AO1":cluster{"signal type":enum16{"Sine Wave", "Triangle Wave", "Square Wave", "Sawtooth Wave"}, "Frequency":dbl, "Amplitude":dbl, "Offset":dbl, "Phase":dbl, "Duty Cycle":dbl}, "AO1Enable":bool, "AO2":cluster{"signal type":enum16{"Sine Wave", "Triangle Wave", "Square Wave", "Sawtooth Wave"}, "Frequency":dbl, "Amplitude":dbl, "Offset":dbl, "Phase":dbl, "Duty Cycle":dbl}, "AO3Enable":bool, "Nme":string, "Nme 2":string, "Nme 3":string}
  T62 = typedef "TDMS Read Data.ctl" = cluster{"Image Type":T20, "Width":u32, "Height":u32, "Pixels per Image":u32, "Total Width":u32, "Left Offset":u32, "Image":T18}
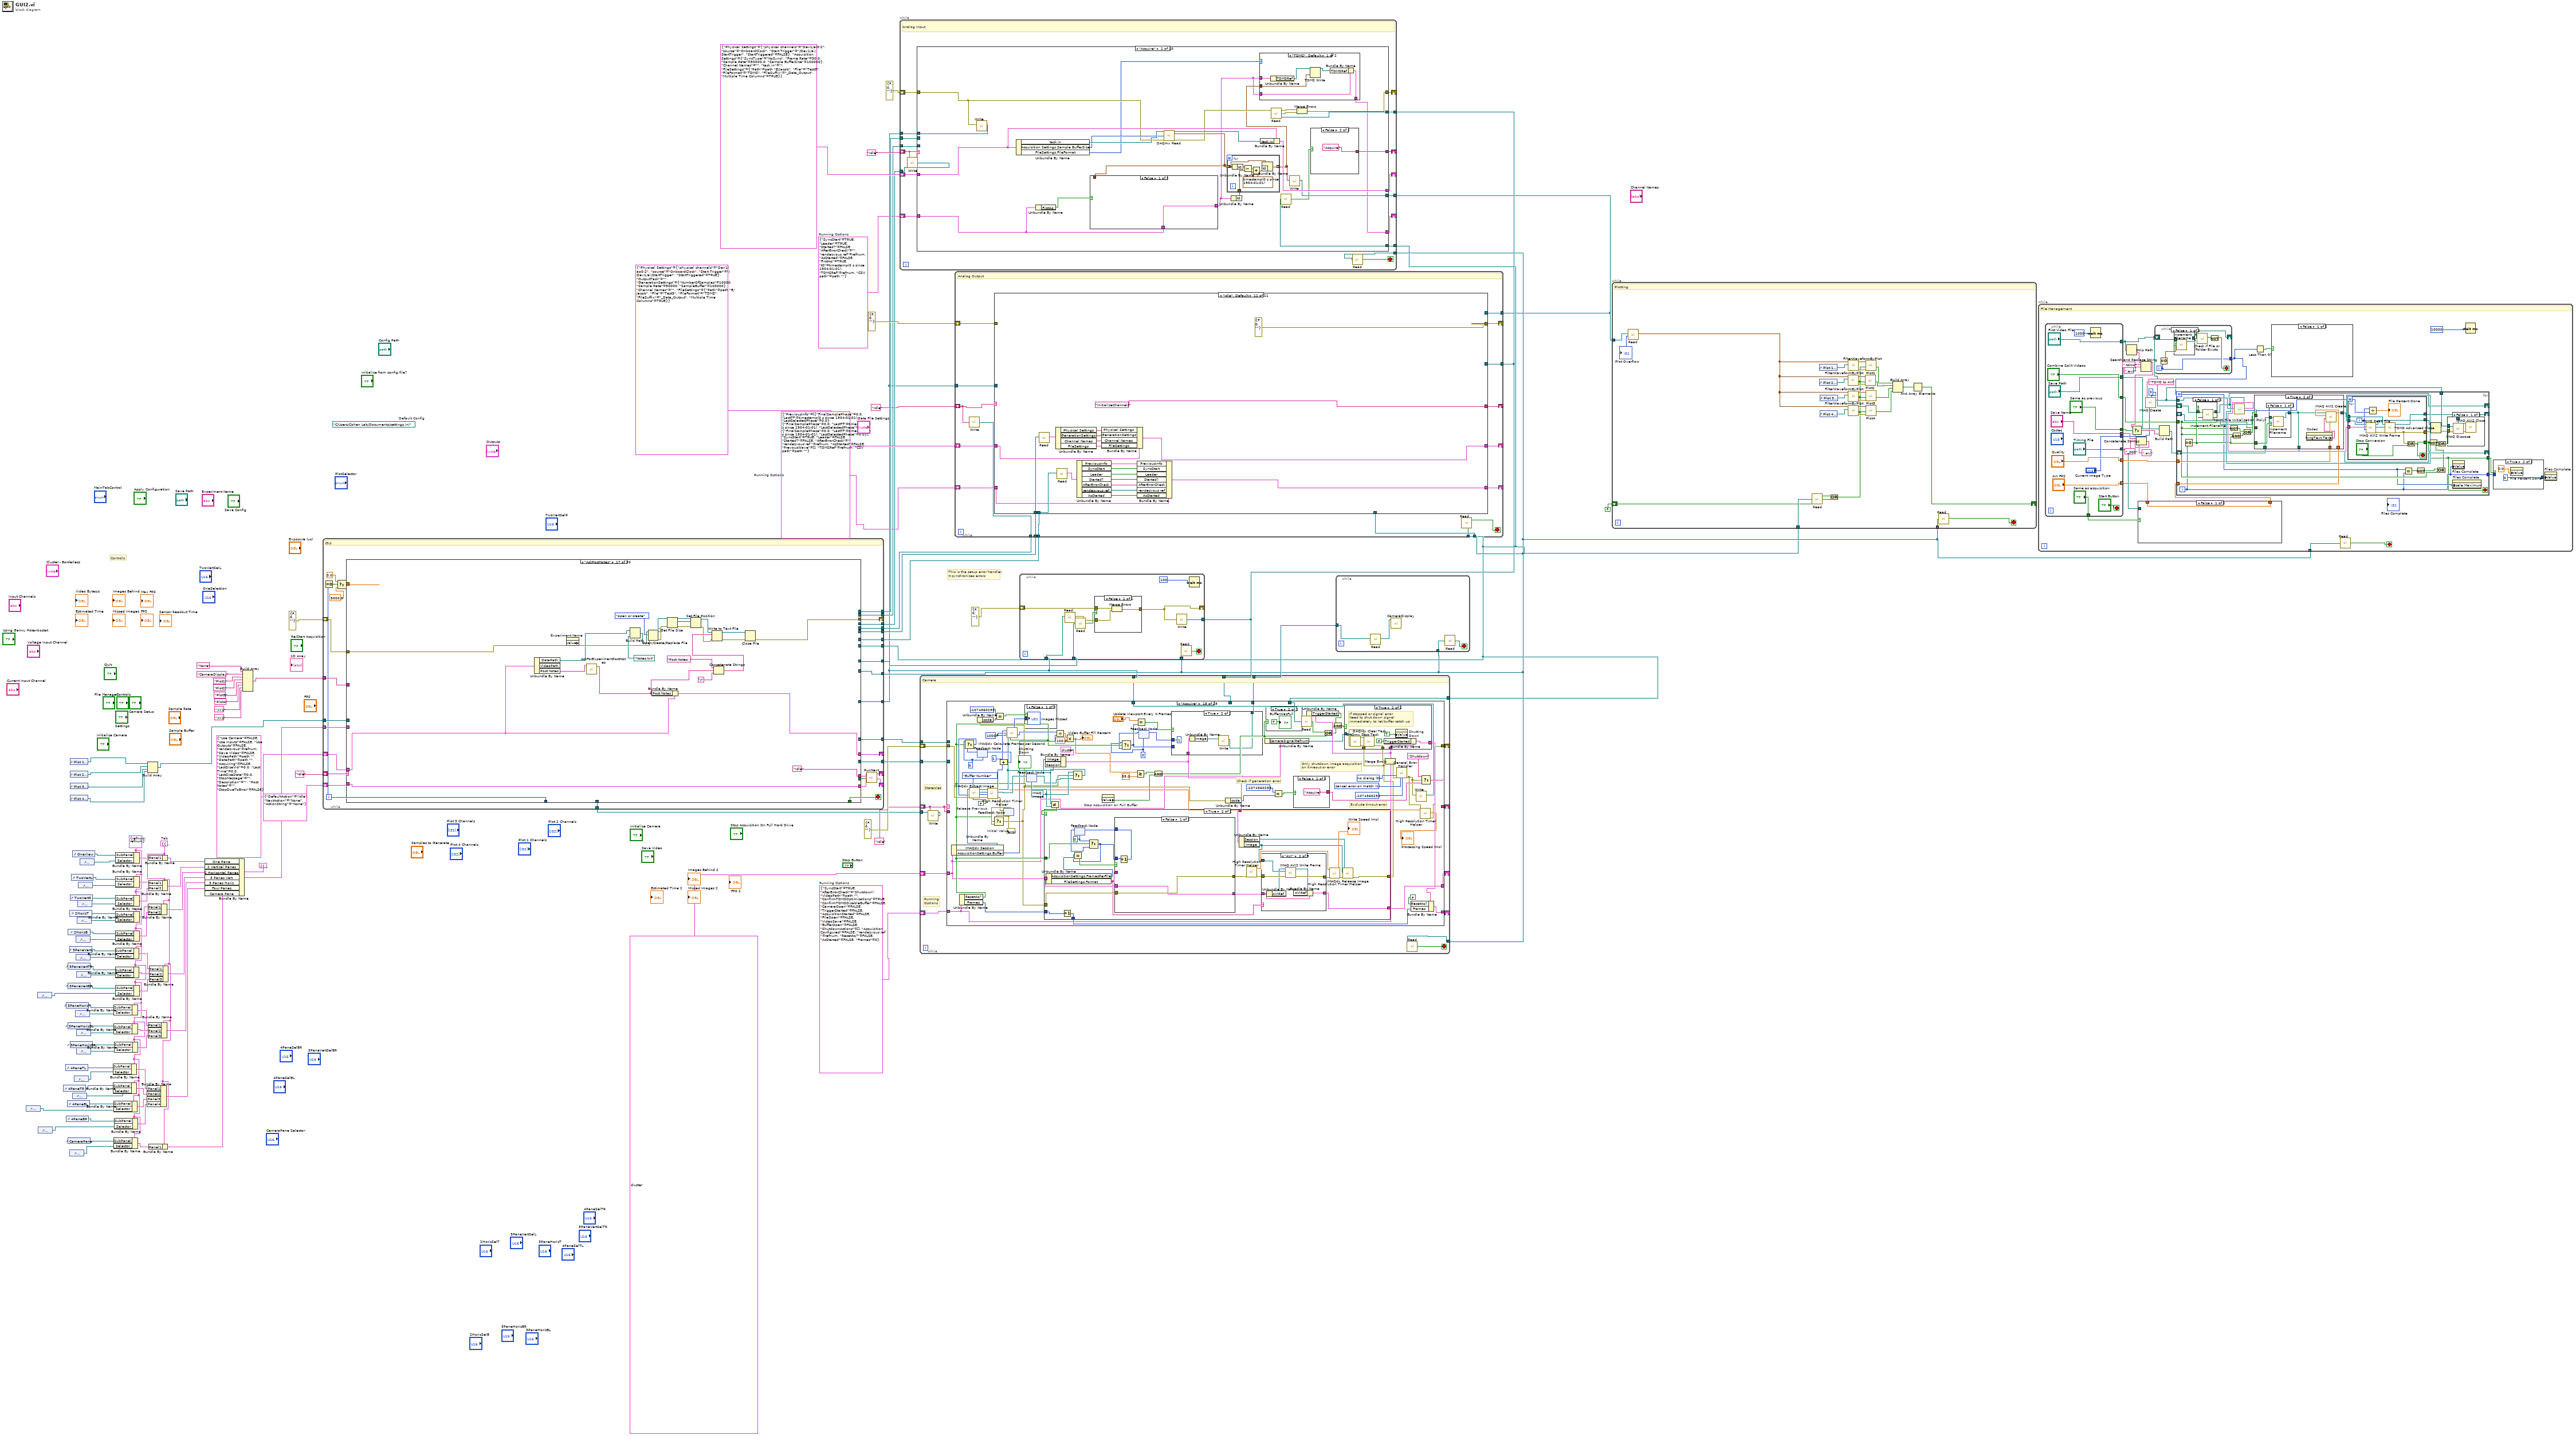
[diagram p0: block diagram]
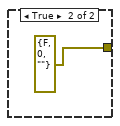
[diagram p2: hidden frame]
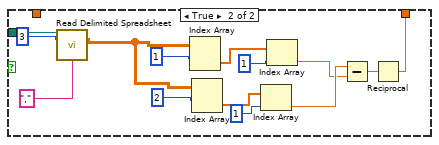
[diagram p3: hidden frame]
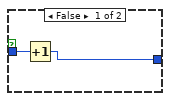
[diagram p4: hidden frame]
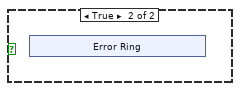
[diagram p9: hidden frame]
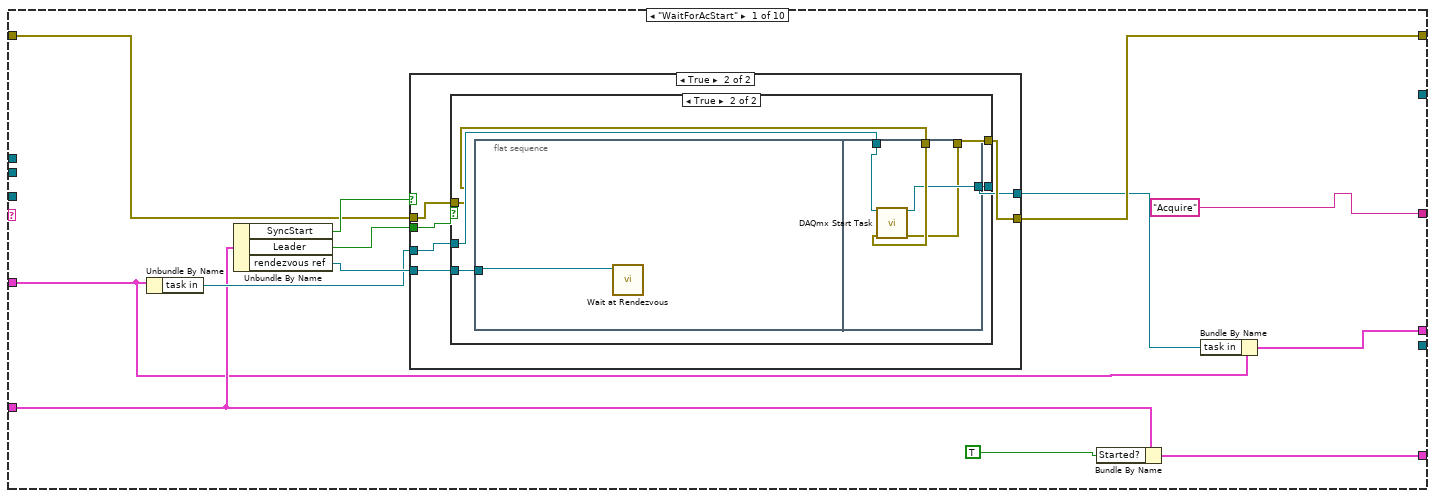
[diagram p11: hidden frame]
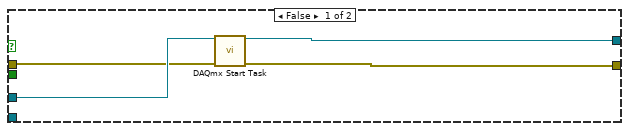
[diagram p12: hidden frame]
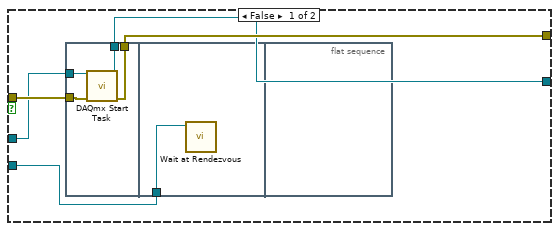
[diagram p13: hidden frame]
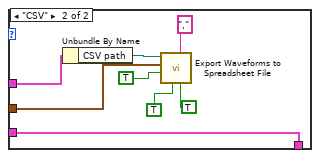
[diagram p14: hidden frame]
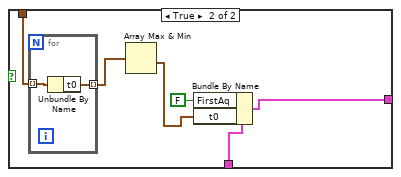
[diagram p15: hidden frame]
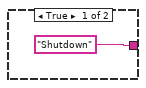
[diagram p16: hidden frame]
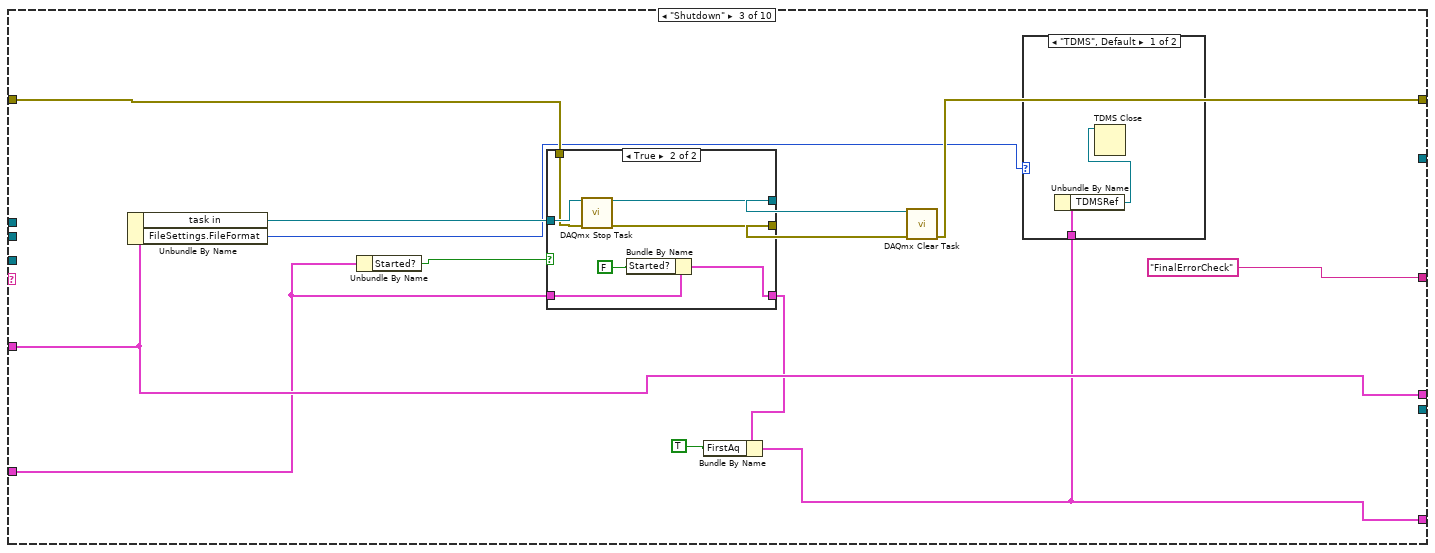
[diagram p17: hidden frame]
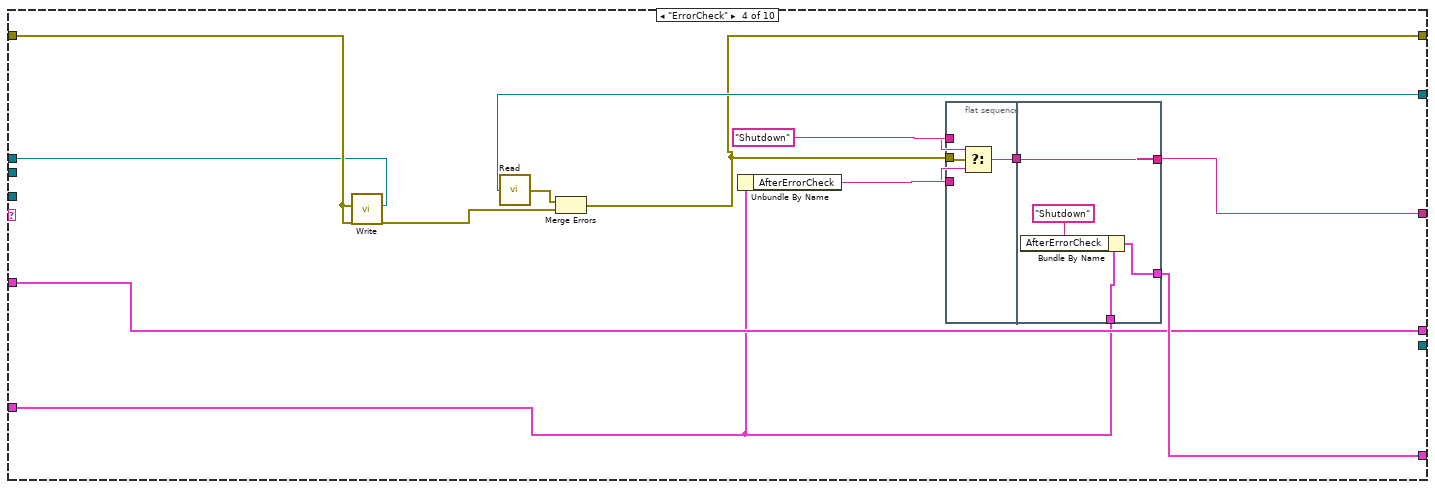
[diagram p20: hidden frame]
diagram:
  w11 = T9 {"SyncStart"=TRUE, "Leader"=TRUE, "Started?"=FALSE, "AfterErrorCheck"="", "rendezvous ref"=refnum, "AcStarted"=FALSE, "FirstAq"=TRUE, "t0"=timestamp(0 s since 1904-01-01), "TDMSRef"=refnum, "CSV path"=path ""}  # Running Options
  w41 = T12 {"SubPanel"=refnum, "Selector"=refnum} ("Panel1")
  w39 = T14 {"Panel2"={"SubPanel"=refnum, "Selector"=refnum}, "Panel3"={"SubPanel"=refnum, "Selector"=refnum}, "Panel4"={"SubPanel"=refnum, "Selector"=refnum}, "Panel1"={"SubPanel"=refnum, "Selector"=refnum}}  # Tab
  w12 = T15 {"PreviousInfo"=[{"FinalSamplePhase"=0.0, "LastTf"=timestamp(0 s since 1904-01-01), "LastSelectedPhase"=0.0}, {"FinalSamplePhase"=0.0, "LastTf"=timestamp(0 s since 1904-01-01), "LastSelectedPhase"=0.0}, {"FinalSamplePhase"=0.0, "LastTf"=timestamp(0 s since 1904-01-01), "LastSelectedPhase"=0.0}], "SyncStart"=TRUE, "Leader"=FALSE, "Started?"=FALSE, "AfterErrorCheck"="", "rendezvous ref "=refnum, "AcStarted"=FALSE, "PrevousWave"=[], "TDMSRef"=refnum, "CSV path"=path ""}  # Running Options
  w10 = T17 {"SyncStart"=TRUE, "AfterErrorCheck"="Shutdown", "VideoPath"=path "", "ConfirmTDMSOptimizations"=TRUE, "ConfirmTDMSDisableBuffer"=FALSE, "CameraOpen"=FALSE, "TriggerStarted"=FALSE, "AcquisitionStarted"=FALSE, "FileOpen"=FALSE, "VideoSave"=FALSE, "BufferOpen"=FALSE, "ShutdownActions"=[], "Acquisition Configured"=FALSE, "rendezvous ref "=refnum, "ResetAq?"=FALSE, "AcStarted"=FALSE, "Frames"=0}  # Running Options
  (unwired) path "C:/Users/Cohen Lab/Documents/settings.ini"  # Default Config
  # "This is the setup error handler\nIt synchronizes errors"
  # "Controls"
  n1 = control-ref of="4PaneSelBL"() -> (w30:refnum<vi>)
  n2 = control-ref of="3PaneVertSelBR"() -> (w28:refnum<vi>)
  n3 = control-ref of="4PaneSelBR"() -> (w29:refnum<vi>)
  n4 = control-ref of="4PaneTR"() -> (w49:refnum<vi>)
  n5 = control-ref of="4PaneTL"() -> (w50:refnum<vi>)
  n6 = control-ref of="3PaneHorizT"() -> (w53:refnum<vi>)
  n7 = control-ref of="4PaneBR"() -> (w47:refnum<vi>)
  n8 = control-ref of="4PaneBL"() -> (w48:refnum<vi>)
  n9 = control-ref of="3PaneVertBR"() -> (w67:refnum<vi>)
  n10 = control-ref of="CameraPane"() -> (w43:refnum<vi>)
  n11 = control-ref of="2HorizB"() -> (w76:refnum<vi>)
  n12 = control-ref of="3PaneVertTR"() -> (w69:refnum<vi>)
  n13 = control-ref of="3PaneHorizBL"() -> (w52:refnum<vi>)
  n14 = control-ref of="2HorizT"() -> (w44:refnum<vi>)
  n15 = control-ref of="3PaneVertL"() -> (w71:refnum<vi>)
  n16 = control-ref of="CameraPane Selector"() -> (w42:refnum<vi>)
  n17 = control-ref of="Plot 4 Channels"() -> (w5:refnum<vi>)
  n18 = control-ref of="TwoVertR"() -> (w85:refnum<vi>)
  n19 = control-ref of="3PaneHorizBR"() -> (w51:refnum<vi>)
  n20 = control-ref of="Plot 1 Channels"() -> (w8:refnum<vi>)
  n21 = control-ref of="Plot 2 Channels"() -> (w7:refnum<vi>)
  n22 = control-ref of="Plot 3 Channels"() -> (w6:refnum<vi>)
  n23 = control-ref of="TwoVertL"() -> (w88:refnum<vi>)
  n24 = control-ref of="OneView"() -> (w93:refnum<vi>)
  n25 = control-ref of="4PaneSelTR"() -> (w54:refnum<vi>)
  n26 = control-ref of="4PaneSelTL"() -> (w55:refnum<vi>)
  n27 = control-ref of="3PaneHorizT"() -> (w58:refnum<vi>)
  n28 = control-ref of="2HorizSelB"() -> (w78:refnum<vi>)
  n29 = control-ref of="3PaneVertSelL"() -> (w70:refnum<vi>)
  n30 = control-ref of="3PaneVertSelTR"() -> (w68:refnum<vi>)
  n31 = control-ref of="3PaneHorizBL"() -> (w57:refnum<vi>)
  n32 = control-ref of="3PaneHorizBR"() -> (w56:refnum<vi>)
  n33 = control-ref of="2HorizSelT"() -> (w77:refnum<vi>)
  n34 = control-ref of="TwoVertSelR"() -> (w84:refnum<vi>)
  n35 = control-ref of="TwoVertSelL"() -> (w87:refnum<vi>)
  n36 = control-ref of="OneSelection"() -> (w92:refnum<vi>)
  n37 = Bundle By Name(cluster=w41, "SubPanel"=w50, "Selector"=w55) -> (w62:T12)
  n38 = Bundle By Name(cluster=w41, "SubPanel"=w49, "Selector"=w54) -> (w61:T12)
  n39 = Bundle By Name(cluster=w41, "SubPanel"=w48, "Selector"=w30) -> (w60:T12)
  n40 = Bundle By Name(cluster=w41, "SubPanel"=w53, "Selector"=w58) -> (w65:T12)
  n41 = Bundle By Name(cluster=w41, "SubPanel"=w52, "Selector"=w57) -> (w64:T12)
  n42 = Bundle By Name(cluster=w41, "SubPanel"=w43, "Selector"=w42) -> (w38:T12)
  n43 = Bundle By Name(cluster=w41, "SubPanel"=w51, "Selector"=w56) -> (w63:T12)
  n44 = Bundle By Name(cluster=w41, "SubPanel"=w47, "Selector"=w29) -> (w59:T12)
  n45 = Bundle By Name(cluster=w41, "SubPanel"=w71, "Selector"=w70) -> (w75:T12)
  n46 = Bundle By Name(cluster=w41, "SubPanel"=w69, "Selector"=w68) -> (w74:T12)
  n47 = Bundle By Name(cluster=w41, "SubPanel"=w93, "Selector"=w92) -> (w91:T12)
  n48 = Bundle By Name(cluster=w41, "SubPanel"=w88, "Selector"=w87) -> (w86:T12)
  n49 = Bundle By Name(cluster=w41, "SubPanel"=w85, "Selector"=w84) -> (w83:T12)
  n50 = Bundle By Name(cluster=w41, "SubPanel"=w44, "Selector"=w77) -> (w81:T12)
  n51 = Bundle By Name(cluster=w41, "SubPanel"=w76, "Selector"=w78) -> (w80:T12)
  n52 = Bundle By Name(cluster=w41, "SubPanel"=w67, "Selector"=w28) -> (w73:T12)
  n53 = Bundle By Name(cluster=w39, "Panel1"=w62, "Panel2"=w61, "Panel3"=w60, "Panel4"=w59) -> (w45:T14)
  n54 = Build Array(w8, w7, w6, w5) -> (w9:refnum<vi>[])
  n55 = Bundle By Name(cluster=w39, "Panel1"=w81, "Panel2"=w80) -> (w79:T14)
  n56 = Bundle By Name(cluster=w39, "Panel1"=w65, "Panel2"=w64, "Panel3"=w63) -> (w66:T14)
  n57 = Bundle By Name(cluster=w39, "Panel1"=w86, "Panel2"=w83) -> (w82:T14)
  n58 = Bundle By Name(cluster=w39, "Panel1"=w38) -> (w40:T14)
  n59 = Bundle By Name(cluster=w39, "Panel1"=w91) -> (w89:T14)
  n60 = Bundle By Name(cluster=w39, "Panel1"=w75, "Panel2"=w74, "Panel3"=w73) -> (w72:T14)
  n61 = Bundle By Name(cluster=T13 {"One Pane"={"Panel2"={"SubPanel"=refnum, "Selector"=refnum}, "Panel3"={"SubPanel"=refnum, "Selector"=refnum}, "Panel4"={"SubPanel"=refnum, "Selector"=refnum}, "Panel1"={"SubPanel"=refnum, "Selector"=refnum}}, "2 Vertical Panes"={"Panel2"={"SubPanel"=refnum, "Selector"=refnum}, "Panel3"={"SubPanel"=refnum, "Selector"=refnum}, "Panel4"={"SubPanel"=refnum, "Selector"=refnum}, "Panel1"={"SubPanel"=refnum, "Selector"=refnum}}, "2 Horizontal Panes"={"Panel2"={"SubPanel"=refnum, "Selector"=refnum}, "Panel3"={"SubPanel"=refnum, "Selector"=refnum}, "Panel4"={"SubPanel"=refnum, "Selector"=refnum}, "Panel1"={"SubPanel"=refnum, "Selector"=refnum}}, "3 Panes Vert"={"Panel2"={"SubPanel"=refnum, "Selector"=refnum}, "Panel3"={"SubPanel"=refnum, "Selector"=refnum}, "Panel4"={"SubPanel"=refnum, "Selector"=refnum}, "Panel1"={"SubPanel"=refnum, "Selector"=refnum}}, "3 Panes Horiz"={"Panel2"={"SubPanel"=refnum, "Selector"=refnum}, "Panel3"={"SubPanel"=refnum, "Selector"=refnum}, "Panel4"={"SubPanel"=refnum, "Selector"=refnum}, "Panel1"={"SubPanel"=refnum, "Selector"=refnum}}, "Four Panes"={"Panel2"={"SubPanel"=refnum, "Selector"=refnum}, "Panel3"={"SubPanel"=refnum, "Selector"=refnum}, "Panel4"={"SubPanel"=refnum, "Selector"=refnum}, "Panel1"={"SubPanel"=refnum, "Selector"=refnum}}, "Camera Pane"={"Panel2"={"SubPanel"=refnum, "Selector"=refnum}, "Panel3"={"SubPanel"=refnum, "Selector"=refnum}, "Panel4"={"SubPanel"=refnum, "Selector"=refnum}, "Panel1"={"SubPanel"=refnum, "Selector"=refnum}}}, "One Pane"=w89, "2 Vertical Panes"=w82, "2 Horizontal Panes"=w79, "3 Panes Vert"=w72, "3 Panes Horiz"=w66, "Four Panes"=w45, "Camera Pane"=w40) -> (w46:T13)
  n62 = Build Array("None", "CameraDisplay", "Plot1", "Plot2", "Plot3", "Plot4", "XY1", "XY2") -> (w94:string[])
  n63 = while {
    shift-right: [w130] -> _
    shift-left: "Idle" ("NextAction") -> [w140]
    shift-right: [w135] -> _
    shift-left: errorcluster {"status"=FALSE, "code"=0, "source"=""} ("error constant") -> [w134]
    tunnel: w94 -> [w133]
    tunnel: w46 -> [w132]
    shift-right: [w129] -> _
    shift-left: T11 {"DefaultAction"="Idle", "NextAction"="None", "ActionString"="None"} -> [w131]
    shift-right: [w124] -> _
    shift-left: T8 {"Use Camera"=FALSE, "Use Inputs"=FALSE, "Use Outputs"=FALSE, "rendezvous"=refnum, "Save Video"=FALSE, "VideoPath"=path "", "DataPath"=path "", "Acquiring"=FALSE, "LastSizeVid"=0.0, "Last Time"=0.0, "LastSizeData"=0.0, "StopMessage"="", "Description"="", "Post Notes"="", "StopDueToError"=FALSE} -> [w125]
    tunnel: [w123] -> w26
    tunnel: [w122] -> w25
    tunnel: [w121] -> w24
    tunnel: [w120] -> w23
    tunnel: [w119] -> w22
    tunnel: [w118] -> w21
    tunnel: w20 -> [w117]
    tunnel: w19 -> [w116]
    tunnel: w18 -> [w115]
    tunnel: [w114] -> w3
    tunnel: [w113] -> w17
    tunnel: [w112] -> w16
    tunnel: [w110] -> w13
    tunnel: w9 -> [w109]
    i -> [w108]
    stop <- w111 stop-if-true
    # "GUI"
    n64 = Equal To 0?(x=w108) -> (x = 0?=w139:bool)
    n65 = Select(t=0.0, s=w139, f=5000.0) -> (s? t:f=w136:dbl)
    n66 = case shown="\"AskPostNotes\"" w140 {
      selector: w140 -> [w144 _ _ _ _ _ _ _ _ _ _ _ _ _ _ _ _ _ _ _ _ _ _ _ _ _ _ _ _ _]
      tunnel: w136 -> [_ w158 _ _ _ _ _ _ _ _ _ _ _ _ _ _ _ _ _ _ _ _ _ _ _ _ _ _ _ _]
      tunnel: w134 -> [w142 w157 w205 w232 w245 w273 w351 w428 w433 w445 w464 w499 w518 w545 w547 w623 w647 w664 w699 w711 w796 w880 w947 w989 w1050 w1089 w1094 w1106 w1129 w1189]
      tunnel: [w142 w157 w205 w232 w245 w273 w341 w428 w433 w448 w464 w499 w518 w545 w547 w622 w648 w663 w699 w711 w796 w880 w947 w989 w1050 w1089 w1096 w1104 w1129 w1189] -> w135
      tunnel: w133 -> [_ _ _ _ w244 _ _ _ _ _ _ _ _ _ _ _ _ _ _ _ _ _ _ _ _ _ _ _ _ _]
      tunnel: w132 -> [_ _ _ _ w242 w280 _ _ _ _ _ _ w520 _ _ _ _ _ _ _ _ _ _ _ _ _ _ _ _ _]
      tunnel: w131 -> [w145 w155 w199 w225 w237 w265 w348 w427 w431 w435 w467 w502 w515 w546 w552 w633 w654 w672 w697 w712 w798 w882 w944 w988 w1039 w1088 w1102 w1110 w1128 w1187]
      tunnel: ["Idle" ("DefaultAction") "Idle" w201 "Idle" "InitializeSubVIs" "Idle" "Idle" "Idle" "CloseOpenVIs" "Idle" "Idle" "Idle" "InitializeSubVIs" "Idle" "Idle" "Idle" ("DefaultAction") "Idle" ("DefaultAction") "Idle" "Idle" ("DefaultAction") "Idle" "Idle" "Idle" "Idle" w991 w1051 "Idle" "Idle" "Idle" w1127 "Break"] -> w128
      tunnel: [w145 w156 w197 w226 w237 w265 w348 w427 w431 w435 w467 w502 w515 w546 w552 w633 w654 w672 w697 w712 w798 w882 w944 w987 w1038 w1088 w1102 w1110 w1128 w1187] -> w127
      tunnel: [_ _ w200 _ TRUE _ _ _ _ _ _ _ _ _ _ _ _ _ _ _ _ _ _ w990 w1040 _ _ _ w1114 _] -> w126
      tunnel: w125 -> [w143 w152 w198 w222 w235 w264 w337 w425 w430 w434 w465 w500 w514 w543 w551 w629 w656 w671 w698 w706 w797 w881 w943 w986 w1037 w1084 w1100 w1108 w1116 w1188]
      tunnel: [w143 w151 w198 w222 w235 w264 w337 w425 w430 w434 w465 w500 w514 w542 w550 w631 w655 w670 w698 w706 w797 w881 w943 w985 w1049 w1084 w1100 w1108 w1125 w1188] -> w124
      tunnel: [_ _ _ _ _ _ _ _ _ _ _ _ _ _ _ _ _ _ _ w710 _ _ _ _ _ _ _ _ _ _] -> w123
      tunnel: [_ _ _ _ _ _ _ _ _ _ _ _ _ _ _ _ _ _ _ w709 _ _ _ _ _ _ _ _ _ _] -> w122
      tunnel: [_ _ _ _ _ _ _ _ _ _ _ _ _ _ _ _ _ _ _ _ w801 _ _ _ _ _ _ _ _ _] -> w121
      tunnel: [_ _ _ _ _ _ _ _ _ _ _ _ _ _ _ _ _ _ _ _ w800 _ _ _ _ _ _ _ _ _] -> w120
      tunnel: [_ _ _ _ _ _ _ _ _ _ _ _ _ _ _ _ _ _ _ _ _ w884 _ _ _ _ _ _ _ _] -> w119
      tunnel: [_ _ _ _ _ _ _ _ _ _ _ _ _ _ _ _ _ _ _ _ _ w883 _ _ _ _ _ _ _ _] -> w118
      tunnel: w117 -> [_ _ _ _ _ _ _ _ _ _ _ _ _ _ _ _ _ _ _ _ _ _ w950 w1000 _ _ _ _ w1132 _]
      tunnel: w116 -> [_ _ _ _ _ _ _ _ _ _ _ _ _ _ _ _ _ _ _ _ _ _ w948 w1002 _ _ _ _ w1133 _]
      tunnel: w115 -> [_ _ _ _ _ _ _ _ _ _ _ _ _ _ _ _ _ _ _ _ _ _ w949 w1001 _ _ _ _ w1134 _]
      tunnel: [_ _ _ _ _ _ _ _ _ _ _ _ _ _ _ _ _ _ _ _ _ _ _ _ _ _ _ _ w1130 _] -> w114
      tunnel: [_ w150 _ _ _ _ _ _ _ _ _ _ _ _ _ _ _ _ _ _ _ _ _ _ _ _ _ _ w1131 _] -> w113
      tunnel: [_ _ _ _ _ _ _ _ _ _ _ _ _ _ _ _ _ _ _ _ _ _ _ _ _ _ _ _ _ w1191] -> w112
      tunnel: [_ _ _ _ _ _ _ _ _ _ _ _ _ _ _ _ _ _ _ _ _ _ _ _ _ _ _ _ _ w1190] -> w111
      tunnel: [_ _ _ _ _ _ _ _ _ _ _ _ _ _ _ _ _ _ _ _ _ _ _ _ _ _ _ _ w1126 _] -> w110
      tunnel: w109 -> [_ _ _ _ _ _ _ _ _ _ w478 _ _ _ _ _ _ _ _ _ _ _ _ _ _ _ _ _ _ _]
      tunnel: w108 -> [_ w148 _ _ _ _ _ _ _ _ _ _ _ _ _ _ _ _ _ _ _ _ _ _ _ _ _ _ _ _]
      frame "NameError", Default {
        n67 = Concatenate Strings("The name does not exist" ("message"), w144) -> (w146:string)
        n68 = call "oneButtonTimeout.vi"("message"=w146) -> ()  [unwired: 1 in, 1 out]
      }
      frame "Idle" {
        n69 = event shown="[10] \"Re/Start Acquisition\": Value Change" {
          selector: _ -> [_ _ _ _ _ _ _ _ _ _ _ _ _]
          dyn-events: _ -> [_ _ _ _ _ _ _ _ _ _ _ _ _]
          timeout: w158 -> [_ _ _ _ _ _ _ _ _ _ _ _ _]
          tunnel: [w161 "CloseOpenVIs,InitializeSubVIs" "ChangeNameArray,UpdatePlotSelection" "UpdatePlotSelection" "UpdatePlotSelection,GreyOutputs" "StopAcquisition,ManageCameraButton,StartCamera" "StopAcquisition" _ "StopAcquisition,Abort" "InitializeCameraSelections" "StopAcquisition,SetAcquireState,ExperimentName,CheckDriveSpace,AskDescription,Rendezvous,StartCamera,StartOutput,StartInput,AcquisitionGUI" "UpdateVideoControlExFPS" ("f") "UpdateFPControlExFPS" ("f")] -> w154
          tunnel: w152 -> [w159 w168 w170 w172 w174 w179 w181 _ w187 w189 w193 _ _]
          tunnel: [w159 w168 w170 w172 w174 w180 w181 _ w187 w189 w191 _ _] -> w151
          tunnel: w148 -> [w160 _ _ _ _ _ _ _ _ _ _ _ _]
          event Timeout {
            n70 = event-data() -> ()  [unwired: 1 in, 3 out]
            n71 = case shown="Default" w160 {
              tunnel: [w162 "Initialize"] -> w161
              tunnel: w159 -> [w166 _]
              frame Default {
                n72 = Unbundle By Name(w166) -> ("Acquiring"=w163:bool)
                n73 = Select(t="CheckStatus,CheckHardDrive", s=w163, f="Idle") -> (s? t:f=w162:string)
              }
              frame 0 {
              }
            }
          }
          event "OneSelection", "TwoVertSelR", "TwoVertSelL", "2HorizSelT", "2HorizSelB", "3PaneVertSelL", "3PaneVertSelTR", "3PaneHorizT", "3PaneHorizBR", "3PaneHorizBL", "4PaneSelTL", "4PaneSelTR", "MainTabControl", "PlotSelector": Value Change {
            n74 = event-data() -> ()  [unwired: 1 in, 6 out]
          }
          event "Input Channels": Value Change {
            n75 = event-data() -> ()  [unwired: 1 in, 6 out]
          }
          event "Channel Names": Value Change {
            n76 = event-data() -> ()  [unwired: 1 in, 6 out]
          }
          event "Outputs.AO0Enable", "Outputs.AO1Enable", "Outputs.AO3Enable", "Outputs.AO0Name", "Outputs.AO1Name", "Outputs.AO2Name": Value Change {
            n77 = event-data() -> ()  [unwired: 1 in, 6 out]
          }
          event "Initialize Camera", "Initialize Camera": Value Change {
            w177 = FALSE ("Save Video")
            n78 = event-data() -> ()  [unwired: 1 in, 6 out]
            n79 = Bundle By Name(cluster=w179, "Save Video"=w177, "Use Inputs"=w177, "Use Outputs"=w177, "Use Camera"=TRUE) -> (w180:T8)
          }
          event "Stop Button", "Stop Square": Value Change {
            n80 = event-data() -> ()  [unwired: 1 in, 6 out]
          }
          event "Data File Settings.Temporary Location": Value Change {
            n81 = event-data() -> ("NewVal"=w184:bool)  [unwired: 1 in, 5 out]
            n82 = case shown="False" w184 {
              tunnel: [T22."Enabled" ("Disabled") T22."Disabled and Grayed Out" ("Disabled")] -> w183
              frame False {
              }
              frame True {
              }
            }
            n83 = property on="Data Temporary Storage Location" class="Path"("DisabledEnum"=w183) -> ()  [unwired: 2 in, 2 out]
          }
          event "Quit": Value Change {
            n84 = event-data() -> ()  [unwired: 1 in, 6 out]
          }
          event Value Change {
            n85 = event-data() -> ()  [unwired: 1 in, 6 out]
          }
          event "Re/Start Acquisition": Value Change {
            n86 = event-data() -> ()  [unwired: 1 in, 6 out]
            n87 = property on="Save Video" class="Bool (strict)"() -> ("Value"=w192:bool)  [unwired: 2 in, 2 out]
            n88 = Bundle By Name(cluster=w193, "Save Video"=w192) -> (w191:T8)
          }
          event "FPS", "Exposure (us)": Value Change {
            n89 = event-data() -> ()  [unwired: 1 in, 6 out]
          }
          event "Cluster - Borderless.FPS", "Cluster - Borderless.Exposure (us)": Value Change {
            n90 = event-data() -> ()  [unwired: 1 in, 6 out]
          }
        }
        n91 = call <extravilib>:"Write.vi"("element"=FALSE) -> ("channel"=w150:T27)  [unwired: 1 out]
        n92 = Bundle By Name(cluster=w155, "ActionString"=w154) -> (w156:T11)
      }
      frame "CheckDriveSpace" {
        n93 = Unbundle By Name(w198) -> ("VideoPath"=w209:path, "DataPath"=w208:path)
        n94 = Get Volume Info(11:w209) -> (1:w203:i64)  [unwired: 1 in, 5 out]
        n95 = Get Volume Info(11:w208) -> (1:w204:i64)  [unwired: 1 in, 5 out]
        n96 = Max & Min(x=w203, y=w204) -> (min(x,y)=w207:i64)  [unwired: 1 out]
        n97 = Greater?(x=w207, y=i64 10000000000) -> (0:w202:bool)
        n98 = case shown="False" w202 {
          tunnel: [w211 "Idle"] -> w201
          tunnel: [TRUE FALSE] -> w200
          tunnel: w199 -> [w213 w215]
          tunnel: [w212 w215] -> w197
          frame False {
            w211 = "StopAcquisition"
            n99 = Bundle By Name(cluster=w213, "DefaultAction"=w211, "NextAction"=w211, "ActionString"=w211) -> (w212:T11)
            n100 = call "oneButtonTimeout.vi"("message"="Drive must have more than 10 Gb to run.\nPlease make space before acquiring data.") -> ()  [unwired: 1 in, 1 out]
          }
          frame True {
          }
        }
      }
      frame "Initialize" {
        n101 = Build Array("InitializeSubViSelections", "InitializeCameraSelections", "GreyOutControls", "GreyOutputs" ("element"), "ChangeNameArray" ("element"), "UpdatePlotSelection" ("element"), "UpdateFPControlExFPS" ("element")) -> (w228:string[])
        n102 = call <vilib>:"1D String Array to Delimited String.vi"("delimiter"=",", "string array"=w228) -> ("delimited string"=w224:string)  [unwired: 9 in]
        n103 = Bundle By Name(cluster=w225, "ActionString"=w224) -> (w226:T11)
      }
      frame "InitializeSubViSelections" {
        (unwired) refnum<vi>[][] []
        n104 = Cluster To Array(cluster=w242) -> (array=w243:T28)
        n105 = for {
          tunnel: w243 -> [w249] mode=indexing
          shift-right: [w246] -> w234
          shift-left: refnum<vi>[] [] -> [w247]
          n106 = Cluster To Array(cluster=w249) -> (array=w248:T12[])
          n107 = for {
            tunnel: w248 -> [w255] mode=indexing
            shift-right: [w254] -> w246
            shift-left: w247 -> [w253]
            n108 = Unbundle By Name(w255) -> ("Selector"=w251:refnum<vi>)
            n109 = Equal?(x=refnum<vi> refnum ("Selector"), y=w251) -> (x = y?=w250:bool)
            n110 = case shown="False" w250 {
              tunnel: [w258 w259] -> w254
              tunnel: w253 -> [w257 w259]
              tunnel: w251 -> [w256 _]
              frame False {
                n111 = Insert Into Array(array=w257, new element=w256) -> (w258:refnum<vi>[])  [unwired: 1 in]
              }
              frame True {
              }
            }
          }
        }
        n112 = for {
          tunnel: w244 -> [w260]
          tunnel: w234 -> [w262] mode=indexing
          shift-right: [w263] -> w239
          shift-left: _ -> [w261]
          n113 = property class="Ring (strict)"(reference=w262, error in=w261, "Strings []"=w260) -> (error out=w263:errorcluster)  [unwired: 1 out]
        }
        n114 = Unbundle By Name(w242) -> ("Camera Pane.Panel1.Selector"=w241:refnum<vi>)
        n115 = property class="Ring (strict)"(reference=w241, error in=w239, "Value"=u16 1) -> ()  [unwired: 2 out]
      }
      frame "InitializeSubVIs" {
        n116 = property on="MainTabControl" class="TabCtl (strict)"() -> ("Value"=w281:T1)  [unwired: 2 in, 2 out]
        n117 = case shown="\"Output\"" w281 {
          tunnel: w280 -> [w319 _ w322 _]
          tunnel: [w318 w320 w321 w336] -> w274
          frame "Camera Setup", Default {
            n118 = Unbundle By Name(w319) -> ("Camera Pane"=w318:T14)
          }
          frame "Settings" {
            w320 = T14 {"Panel2"={"SubPanel"=refnum, "Selector"=refnum}, "Panel3"={"SubPanel"=refnum, "Selector"=refnum}, "Panel4"={"SubPanel"=refnum, "Selector"=refnum}, "Panel1"={"SubPanel"=refnum, "Selector"=refnum}}  # Tab
          }
          frame "Output" {
            n119 = property on="PlotSelector" class="TabCtl (strict)"() -> ("Value"=w323:T6)  [unwired: 2 in, 2 out]
            n120 = case shown="\"3 Panes Vert\"" w323 {
              tunnel: w322 -> [w325 w327 w329 w331 w333 w335]
              tunnel: [w324 w326 w328 w330 w332 w334] -> w321
              frame "One Pane", Default {
                n121 = Unbundle By Name(w325) -> ("One Pane"=w324:T14)
              }
              frame "2 Vertical Panes" {
                n122 = Unbundle By Name(w327) -> ("2 Vertical Panes"=w326:T14)
              }
              frame "2 Horizontal Panes" {
                n123 = Unbundle By Name(w329) -> ("2 Horizontal Panes"=w328:T14)
              }
              frame "3 Panes Vert" {
                n124 = Unbundle By Name(w331) -> ("3 Panes Vert"=w330:T14)
              }
              frame "3 Panes Horiz" {
                n125 = Unbundle By Name(w333) -> ("3 Panes Horiz"=w332:T14)
              }
              frame "Four Panes" {
                n126 = Unbundle By Name(w335) -> ("Four Panes"=w334:T14)
              }
            }
          }
          frame "File Management" {
            w336 = T14 {"Panel2"={"SubPanel"=refnum, "Selector"=refnum}, "Panel3"={"SubPanel"=refnum, "Selector"=refnum}, "Panel4"={"SubPanel"=refnum, "Selector"=refnum}, "Panel1"={"SubPanel"=refnum, "Selector"=refnum}}  # Tab
          }
        }
        n127 = Unbundle By Name(w274) -> ("Panel1"=w275:T12, "Panel2"=w276:T29, "Panel3"=w277:T29, "Panel4"=w278:T29)
        n128 = Build Array(w275, w276, w277, w278) -> (w279:T12[])
        n129 = for {
          tunnel: w279 -> [w290] mode=indexing
          shift-right: [w285] -> w272
          shift-left: refnum<vi>[] [] -> [w284]
          shift-right: [w283] -> w271
          shift-left: refnum<vi>[] [] -> [w282]
          n130 = Unbundle By Name(w290) -> ("SubPanel"=w286:refnum<vi>, "Selector"=w287:refnum<vi>)
          n131 = Equal?(x=refnum<vi> refnum ("OneView"), y=w286) -> (x = y?=w288:bool)
          n132 = case shown="True" w288 {
            tunnel: w287 -> [w296 _]
            tunnel: w286 -> [w295 _]
            tunnel: [w294 w298] -> w285
            tunnel: w284 -> [w293 w298]
            tunnel: [w292 w297] -> w283
            tunnel: w282 -> [w291 w297]
            frame False {
              n133 = Insert Into Array(array=w293, new element=w295) -> (w294:refnum<vi>[])  [unwired: 1 in]
              n134 = Insert Into Array(array=w291, new element=w296) -> (w292:refnum<vi>[])  [unwired: 1 in]
            }
            frame True {
            }
          }
        }
        n135 = for {
          tunnel: w272 -> [w305] mode=indexing
          tunnel: w271 -> [w304] mode=indexing
          shift-right: [w300] -> w270
          shift-left: string[] [] -> [w299]
          n136 = property class="Ring (strict)"(reference=w304) -> ("RingText.Text"=w301:string)  [unwired: 1 in, 2 out]
          n137 = Not Equal?(x="None", y=w301) -> (x != y?=w302:bool)
          n138 = case shown="True" w302 {
            tunnel: w305 -> [_ w310]
            tunnel: w301 -> [_ w311]
            tunnel: [w306 w309] -> w300
            tunnel: w299 -> [w306 w308]
            frame False {
            }
            frame True {
              n139 = Current VI's Path() -> (path=w313:path)
              n140 = property class="SubPnl"(reference=w310) -> ("Label.Text"=w307:string)  [unwired: 1 in, 2 out]
              n141 = Strip Path(path=w313) -> (stripped path=w312:path)  [unwired: 1 out]
              n142 = Concatenate Strings(w311, ".vi") -> (w315:string)
              n143 = Build Path(base path=w312, name or relative path=w315) -> (appended path=w314:path)
              n144 = Open VI Reference(vi path=w314) -> (vi reference=w316:refnum<vi>)  [unwired: 5 in, 1 out]
              n145 = invoke class="SubPnl" method="Insert VI"(reference=w310, "VI Ref"=w316) -> ()  [unwired: 2 in, 4 out]
              n146 = Insert Into Array(array=w308, new element=w307) -> (w309:string[])  [unwired: 1 in]
            }
          }
        }
        "Array 2" <- w270
      }
      frame "InitializeCameraSelections" {
        n147 = control-ref of="Camera Ref"() -> (w354:refnum<vi>)
        n148 = property class="IMAQdx (strict)"(reference=w354, error in=w351) -> (error out=w350:errorcluster, "Value"=w349:T2)  [unwired: 1 out]
        n149 = Not Equal?(x=T2 refnum ("Value"), y=w349) -> (x != y?=w352:bool)
        n150 = case shown="True" w352 {
          tunnel: w350 -> [w356 w367]
          tunnel: w349 -> [_ w366]
          tunnel: [w356 w359] -> w339
          tunnel: [w355 w363] -> w342
          tunnel: [w355 w358] -> w340
          tunnel: [w355 w357] -> w338
          frame False {
            w355 = T22."Disabled and Grayed Out" ("Disabled")
          }
          frame True {
            n151 = call <vilib>:"IMAQdx Open Camera.vi"("error in"=w367, "Session In"=w366) -> ("error out"=w365:errorcluster, "Session Out"=w371:T2)  [unwired: 8 in]
            n152 = property class="IMAQdx"(reference=w371, error in=w365) -> (reference out=w362:T2, error out=w364:errorcluster, "VendorName"=w370:string)
            n153 = Equal?(x=w370, y="Basler") -> (x = y?=w368:bool)
            n154 = case shown="True" w368 {
              tunnel: w364 -> [w374 w386]
              tunnel: [w376 w379] -> w360
              tunnel: [w372 T22."Enabled" ("Disabled")] -> w363
              tunnel: w362 -> [w373 w383]
              tunnel: [w373 w383] -> w361
              tunnel: [w372 w382] -> w358
              tunnel: [w372 w377] -> w357
              frame False {
                w372 = T22."Disabled and Grayed Out" ("Disabled")
                n155 = Merge Errors(w374, errorcluster {"status"=TRUE, "code"=258, "source"="Camera is Unsupported at this time"} ("error constant")) -> (w376:errorcluster)
              }
              frame True {
                w388 = u32 64 ("y")
                n156 = property class="IMAQdx"(reference=w383, "ActiveAttribute"="CameraAttributes::DeviceControl::DeviceModelName") -> ("ValueString"=w381:string)  [unwired: 1 in, 2 out]
                n157 = case shown="\"acA1300-200um\"" w381 {
                  tunnel: w383 -> [w400 w411 _]
                  tunnel: [T22."Disabled and Grayed Out" ("Disabled") T22."Enabled" ("Disabled") w412] -> w382
                  tunnel: [errorcluster {"status"=FALSE, "code"=0, "source"=""} ("error in") errorcluster {"status"=FALSE, "code"=0, "source"=""} ("error in") errorcluster {"status"=TRUE, "code"=599, "source"="Camera Not Yet Supported"} ("error in")] -> w378
                  tunnel: [T22."Enabled" ("Disabled") T22."Disabled and Grayed Out" ("Disabled") w412] -> w377
                  frame "acA720-520uc" {
                    n158 = property class="IMAQdx"(reference=w400, "ActiveAttribute"="CameraAttributes::AcquisitionControl::ExposureTimeMode") -> ("EnumStrings[]"=w402:string[])  [unwired: 1 in, 2 out]
                    n159 = property on="Exposure Mode" class="Ring (strict)"("Strings []"=w402) -> ()  [unwired: 2 in, 2 out]
                  }
                  frame "acA1300-200um" {
                    n160 = property class="IMAQdx"(reference=w411, "ActiveAttribute"="CameraAttributes::AcquisitionControl::SensorReadoutMode") -> ("EnumStrings[]"=w409:string[])  [unwired: 1 in, 2 out]
                    n161 = property on="Sensor readout mode\n(Fast Decreases Quality)" class="Ring (strict)"("Strings []"=w409) -> ()  [unwired: 2 in, 2 out]
                  }
                  frame "NotSupported", Default {
                    w412 = T22."Disabled and Grayed Out" ("Disabled")
                  }
                }
                n162 = property class="IMAQdx"(reference=w383, error in=w386, "ActiveAttribute"="CameraAttributes::ImageFormatControl::PixelFormat", "ActiveAttribute"="CameraAttributes::ImageFormatControl::Width", "ActiveAttribute"="CameraAttributes::ImageFormatControl::Height", "ActiveAttribute"="CameraAttributes::AcquisitionControl::TriggerSource") -> (error out=w380:errorcluster, "EnumStrings[]"=w395:string[], "ValueU32"=w390:u32, "ValueU32"=w392:u32, "EnumStrings[]"=w391:string[])  [unwired: 1 out]
                n163 = for {
                  tunnel: w395 -> [w416] mode=indexing
                  shift-right: [w415] -> w393
                  shift-left: string[] [] -> [w414]
                  n164 = Match Pattern(string=w416, regular expression="p") -> (offset past match=w419:i32)  [unwired: 1 in, 3 out]
                  n165 = Not Equal?(x=w419, y=-1) -> (x != y?=w417:bool)
                  n166 = case shown="False" w417 {
                    tunnel: w416 -> [w423 _]
                    tunnel: [w422 w424] -> w415
                    tunnel: w414 -> [w421 w424]
                    frame False {
                      n167 = Insert Into Array(array=w421, new element=w423) -> (w422:string[])  [unwired: 1 in]
                    }
                    frame True {
                    }
                  }
                }
                n168 = Quotient & Remainder(x=w390, y=w388) -> (floor(x/y)=w389:u32)  [unwired: 1 out]
                n169 = Multiply(x=w389, y=w388) -> (x*y=w387:u32)
                n170 = property on="Signal Line" class="Ring (strict)"("Strings []"=w391) -> ()  [unwired: 2 in, 2 out]
                n171 = property on="Image Width" class="DigNum (strict)"("Value"=w387) -> ()  [unwired: 2 in, 2 out]
                n172 = property on="Image Height" class="DigNum (strict)"("Value"=w392) -> ()  [unwired: 2 in, 2 out]
                n173 = property on="Pixel Format\n(p not supported)" class="Ring (strict)"("Strings []"=w393) -> ()  [unwired: 2 in, 2 out]
                n174 = Merge Errors(w380, w378) -> (w379:errorcluster)
              }
            }
            n175 = call <vilib>:"IMAQdx Close Camera.vi"("error in"=w360, "Session In"=w361) -> ("error out"=w359:errorcluster)  [unwired: 9 out]
          }
        }
        n176 = property on="Signal Line" class="Ring (strict)"("DisabledEnum"=w342) -> (error out=w345:errorcluster)  [unwired: 2 in, 1 out]
        n177 = property on="Image Height" class="DigNum (strict)"("DisabledEnum"=w342) -> (error out=w343:errorcluster)  [unwired: 2 in, 1 out]
        n178 = property on="Pixel Format\n(p not supported)" class="Ring (strict)"("DisabledEnum"=w342) -> (error out=w346:errorcluster)  [unwired: 2 in, 1 out]
        n179 = property on="Image Width" class="DigNum (strict)"("DisabledEnum"=w342) -> (error out=w344:errorcluster)  [unwired: 2 in, 1 out]
        n180 = property on="Exposure Mode" class="Ring (strict)"("DisabledEnum"=w338) -> ()  [unwired: 2 in, 2 out]
        n181 = property on="Sensor readout mode\n(Fast Decreases Quality)" class="Ring (strict)"("DisabledEnum"=w340) -> ()  [unwired: 2 in, 2 out]
        n182 = Merge Errors(w339, w346, w345, w344, w343) -> (w341:errorcluster)
      }
      frame "GreyOutControls" {
        w429 = T22."Enabled" ("Disabled")
        n183 = property on="Cluster - Borderless" class="Clust (strict)"("DisabledEnum"=w429) -> ()  [unwired: 2 in, 2 out]
        n184 = property on="Input Channels" class="DAQmxName"("DisabledEnum"=w429) -> ()  [unwired: 2 in, 2 out]
        n185 = property on="Channel Names" class="Arr (strict)"("DisabledEnum"=w429) -> ()  [unwired: 2 in, 2 out]
        n186 = property on="Sample Rate" class="DigNum (strict)"("DisabledEnum"=w429) -> ()  [unwired: 2 in, 2 out]
        n187 = property on="Save Video" class="Bool (strict)"("DisabledEnum"=w429) -> ()  [unwired: 2 in, 2 out]
        n188 = property on="Sample Buffer" class="DigNum (strict)"("DisabledEnum"=w429) -> ()  [unwired: 2 in, 2 out]
        n189 = property on="Initialize Camera" class="Bool (strict)"("DisabledEnum"=w429) -> ()  [unwired: 2 in, 2 out]
        n190 = property on="Samples to Generate" class="DigNum (strict)"("DisabledEnum"=w429) -> ()  [unwired: 2 in, 2 out]
        n191 = property on="Data File Settings" class="Clust (strict)"("DisabledEnum"=w429) -> ()  [unwired: 2 in, 2 out]
        n192 = property on="FPS" class="DigNum (strict)"("DisabledEnum"=w429) -> ()  [unwired: 2 in, 2 out]
        n193 = property on="Exposure (us)" class="DigNum (strict)"("DisabledEnum"=w429) -> ()  [unwired: 2 in, 2 out]
        n194 = property on="Use Camera" class="Bool (strict)"("DisabledEnum"=w429) -> ()  [unwired: 2 in, 2 out]
        n195 = property on="AO1Enable" class="Bool (strict)"("DisabledEnum"=w429) -> ()  [unwired: 2 in, 2 out]
        n196 = property on="AO3Enable" class="Bool (strict)"("DisabledEnum"=w429) -> ()  [unwired: 2 in, 2 out]
        n197 = property on="AO0Enable" class="Bool (strict)"("DisabledEnum"=w429) -> ()  [unwired: 2 in, 2 out]
      }
      frame "UpdatePlotTab" {
      }
      frame "ChangeNameArray" {
        n198 = control-ref of="Channel Names"() -> (w442:refnum<vi>)
        n199 = property on="Property Node" class="Arr (strict)"(reference=w442) -> ("Value"=w444:string[])  [unwired: 1 in, 2 out]
        n200 = property on="Input Channels" class="DAQmxName"(error in=w445) -> (error out=w447:errorcluster, "Value"=w449:string)  [unwired: 1 in, 1 out]
        n201 = control-ref of="1D Array"() -> (w441:refnum<vi>)
        n202 = call <vilib>:"DAQmx Unflatten Channel String.vi"("names in"=w449, "error in"=w447) -> ("names out"=w440:string[], "error out"=w446:errorcluster)  [unwired: 12 in]
        n203 = property on="Property Node" class="Arr (strict)"(reference=w441, "Value"=w440) -> (reference out=w439:refnum<vi>, error out=w438:errorcluster)  [unwired: 1 in]
        n204 = Array Size(array=w440) -> (size(s)=w437:i32)
        n205 = property on="Property Node" class="Arr (strict)"(reference=w439, error in=w438, "Number of Rows"=w437) -> ()  [unwired: 2 out]
        n206 = for {
          tunnel: w440 -> [w460] mode=indexing
          tunnel: w444 -> [w457]
          tunnel: [w459] -> w443 mode=indexing
          i -> [w458]
          n207 = Index Array(array=w457, index=w458) -> (element=w450:string)
          n208 = Equal?(x="", y=w450) -> (x = y?=w453:bool)
          n209 = Match Pattern(string=w450, regular expression="Dev") -> (offset past match=w455:i32)  [unwired: 1 in, 3 out]
          n210 = Not Equal?(x=w455, y=-1) -> (x != y?=w452:bool)
          n211 = Or(x=w452, y=w453) -> (x .or. y?=w451:bool)
          n212 = case shown="True" w451 {
            tunnel: w450 -> [w462 _]
            tunnel: w460 -> [_ w463]
            tunnel: [w462 w463] -> w459
            frame False {
            }
            frame True {
            }
          }
        }
        n213 = property on="Property Node" class="Arr (strict)"(reference=w442, error in=w446, "Number of Rows"=w437) -> (error out=w448:errorcluster)  [unwired: 1 out]
        n214 = property on="Property Node" class="Arr (strict)"(reference=w442, "Value"=w443) -> ()  [unwired: 1 in, 2 out]
      }
      frame "UpdatePlotSelection" {
        n215 = property on="Channel Names" class="Arr (strict)"() -> ("Value"=w477:string[])  [unwired: 2 in, 2 out]
        n216 = property on="Outputs" class="Clust (strict)"() -> ("Value"=w476:T5)  [unwired: 2 in, 2 out]
        n217 = Unbundle By Name(w476) -> ("AO0Enable"=w472:bool, "AO1Enable"=w471:bool, "AO3Enable"=w470:bool, "AO0Name"=w475:string, "AO1Name"=w474:string, "AO2Name"=w473:string)
        n218 = Build Array(w475, w474, w473) -> (w469:string[])
        n219 = Build Array(w472, w471, w470) -> (w468:bool[])
        n220 = for {
          tunnel: w478 -> [w485] mode=indexing
          tunnel: w477 -> [w484]
          tunnel: w469 -> [w488]
          tunnel: w468 -> [w487]
          n221 = for {
            tunnel: w488 -> [w492] mode=indexing
            tunnel: w487 -> [w491] mode=indexing
            shift-right: [w490] -> w483
            shift-left: string[] [] -> [w489]
            n222 = case shown="False" w491 {
              tunnel: w492 -> [_ w496]
              tunnel: [w493 w495] -> w490
              tunnel: w489 -> [w493 w494]
              frame False {
              }
              frame True {
                n223 = Build Array (concatenate)(w494, w496) -> (w495:string[])
              }
            }
          }
          n224 = Insert Into Array(array=w484, new element=w483) -> (w482:string[])  [unwired: 1 in]
          n225 = Insert Into Array(array=w482, index=0, new element="None" ("new element/subarray")) -> (w479:string[])
          n226 = property on="XY2 X" class="Ring (strict)"("Strings []"=w479) -> ()  [unwired: 2 in, 2 out]
          n227 = property on="XY2 Y" class="Ring (strict)"("Strings []"=w479) -> ()  [unwired: 2 in, 2 out]
          n228 = property class="LstBox (strict)"(reference=w485, "Item Names"=w482) -> ()  [unwired: 1 in, 2 out]
          n229 = property on="XY1 X" class="Ring (strict)"("Strings []"=w479) -> ()  [unwired: 2 in, 2 out]
          n230 = property on="XY1 Y" class="Ring (strict)"("Strings []"=w479) -> ()  [unwired: 2 in, 2 out]
        }
      }
      frame "GreyOutputs" {
        n231 = property on="Outputs" class="Clust (strict)"() -> ("Value"=w507:T5)  [unwired: 2 in, 2 out]
        n232 = Unbundle By Name(w507) -> ("AO0Enable"=w506:bool, "AO1Enable"=w498:bool, "AO3Enable"=w497:bool)
        n233 = case shown="False" w497 {
          tunnel: [T22."Disabled and Grayed Out" ("DisabledEnum") T22."Enabled" ("DisabledEnum")] -> w503
          frame False {
          }
          frame True {
          }
        }
        n234 = case shown="False" w506 {
          tunnel: [T22."Disabled and Grayed Out" ("DisabledEnum") T22."Enabled" ("DisabledEnum")] -> w505
          frame False {
          }
          frame True {
          }
        }
        n235 = case shown="False" w498 {
          tunnel: [T22."Disabled and Grayed Out" ("DisabledEnum") T22."Enabled" ("DisabledEnum")] -> w504
          frame False {
          }
          frame True {
          }
        }
        n236 = property on="AO0" class="Clust (strict)"("DisabledEnum"=w505) -> ()  [unwired: 2 in, 2 out]
        n237 = property on="AO2" class="Clust (strict)"("DisabledEnum"=w503) -> ()  [unwired: 2 in, 2 out]
        n238 = property on="AO1" class="Clust (strict)"("DisabledEnum"=w504) -> ()  [unwired: 2 in, 2 out]
      }
      frame "CloseOpenVIs" {
        n239 = Cluster To Array(cluster=w520) -> (array=w522:T28)
        n240 = for {
          tunnel: w522 -> [w526] mode=indexing
          shift-right: [w524] -> w519
          shift-left: refnum<vi>[] [] -> [w523]
          n241 = Cluster To Array(cluster=w526) -> (array=w525:T12[])
          n242 = for {
            tunnel: w525 -> [w530] mode=indexing
            shift-right: [w528] -> w524
            shift-left: w523 -> [w527]
            n243 = Unbundle By Name(w530) -> ("SubPanel"=w529:refnum<vi>)
            n244 = Insert Into Array(array=w527, new element=w529) -> (w528:refnum<vi>[])  [unwired: 1 in]
          }
        }
        n245 = for {
          tunnel: w519 -> [w534] mode=indexing
          shift-right: [w532] -> w517
          shift-left: _ -> [w531]
          n246 = Equal?(x=refnum<vi> refnum ("Selector"), y=w534) -> (x = y?=w533:bool)
          n247 = case shown="False" w533 {
            tunnel: w534 -> [w539 _]
            tunnel: [w537 w540] -> w532
            tunnel: w531 -> [w536 w540]
            frame False {
              n248 = property class="SubPnl"(reference=w539) -> ("Label.Text"=w538:string)  [unwired: 1 in, 2 out]
              n249 = invoke class="SubPnl" method="Remove VI"(reference=w539) -> ()  [unwired: 2 in, 3 out]
              n250 = Insert Into Array(array=w536, new element=w538) -> (w537:string[])  [unwired: 1 in]
            }
            frame True {
            }
          }
        }
        "Array" <- w517
      }
      frame "SetAcquireState" {
        n251 = Bundle By Name(cluster=w543, "Acquiring"=TRUE) -> (w542:T8)
      }
      frame "ExperimentName" {
        n252 = property on="Data Temporary Storage Location" class="Path"() -> ("Value"=w555:path)  [unwired: 2 in, 2 out]
        n253 = property on="Temporary Location" class="Bool (strict)"() -> ("Value"=w556:bool)  [unwired: 2 in, 2 out]
        n254 = property on="Experiment Name" class="Str"() -> ("Value"=w553:string)  [unwired: 2 in, 2 out]
        n255 = property on="Tempory Storage Location\n(File can be moved after acquisition)\nSSD recomended for high frame rate" class="Path"() -> ("Value"=w554:path)  [unwired: 2 in, 2 out]
        n256 = while {
          tunnel: w556 -> [w570]
          tunnel: w555 -> [w558]
          tunnel: w554 -> [w557]
          shift-right: [w566] -> w549
          shift-left: w553 -> [w565]
          tunnel: w551 -> [w563]
          tunnel: [w559] -> w550
          stop <- w564 stop-if-true
          n257 = Build Path(base path=w557, name or relative path=w565) -> (appended path=w562:path)
          n258 = case shown="False" w570 {
            tunnel: w558 -> [w607 _]
            tunnel: w565 -> [w606 _]
            tunnel: [w605 TRUE ("file or folder exists?")] -> w569
            tunnel: w562 -> [_ w608]
            tunnel: [w604 w608] -> w561
            frame False {
              n259 = Build Path(base path=w607, name or relative path=w606) -> (appended path=w604:path)
              n260 = call <vilib>:"Check if File or Folder Exists.vi"("path"=w604) -> ("file or folder exists?"=w605:bool)  [unwired: 8 in, 2 out]
            }
            frame True {
            }
          }
          n261 = call <vilib>:"Check if File or Folder Exists.vi"("path"=w562) -> ("file or folder exists?"=w568:bool, "dup path"=w560:path)  [unwired: 8 in, 1 out]
          n262 = And(x=w568, y=w569) -> (x .and. y?=w567:bool)
          n263 = case shown="True" w567 {
            tunnel: w565 -> [w579 w591]
            tunnel: [w579 w586] -> w566
            tunnel: [TRUE FALSE] -> w564
            tunnel: w563 -> [w573 w594]
            tunnel: w561 -> [w576 _]
            tunnel: w560 -> [w575 _]
            tunnel: [w574 w594] -> w559
            tunnel: w558 -> [_ w590]
            tunnel: w557 -> [_ w589]
            frame False {
              n264 = Equal?(x=w575, y=w576) -> (x = y?=w577:bool)
              n265 = case shown="True" w577 {
                tunnel: w576 -> [w583 w585]
                tunnel: w575 -> [w582 _]
                tunnel: [w581 w584] -> w572
                tunnel: [w580 w584] -> w571
                frame False {
                  n266 = Create Folder(path (use dialog)=w582) -> (created path=w581:path)  [unwired: 2 in, 2 out]
                  n267 = Create Folder(path (use dialog)=w583) -> (created path=w580:path)  [unwired: 2 in, 2 out]
                }
                frame True {
                  n268 = Create Folder(path (use dialog)=w585) -> (created path=w584:path)  [unwired: 2 in, 2 out]
                }
              }
              n269 = Bundle By Name(cluster=w573, "VideoPath"=w572, "DataPath"=w571) -> (w574:T8)
            }
            frame True {
              n270 = call "AskForExperimentName.vi"("String Control"=w591) -> ("Disable Button 2"=w593:bool, "Experiment Name 2"=w586:string)  [unwired: 5 in]
              n271 = Build Path(base path=w589, name or relative path=w586) -> (appended path=w587:path)
              n272 = Build Path(base path=w590, name or relative path=w586) -> (appended path=w588:path)
              n273 = case shown="True" w593 {
                tunnel: w588 -> [_ w597]
                tunnel: w587 -> [_ w595]
                frame False {
                }
                frame True {
                  n274 = Equal?(x=w595, y=w597) -> (x = y?=w598:bool)
                  n275 = case shown="True" w598 {
                    tunnel: w597 -> [w600 w603]
                    tunnel: w595 -> [w601 _]
                    tunnel: TRUE ("entire hierarchy (F)") -> [w599 w602]
                    frame False {
                      n276 = Delete(path (use dialog)=w600, entire hierarchy (F)=w599, confirm (F)=w599) -> ()  [unwired: 2 in, 3 out]
                      n277 = Delete(path (use dialog)=w601, entire hierarchy (F)=w599, confirm (F)=w599) -> ()  [unwired: 2 in, 3 out]
                    }
                    frame True {
                      n278 = Delete(path (use dialog)=w603, entire hierarchy (F)=w602, confirm (F)=w602) -> ()  [unwired: 2 in, 3 out]
                    }
                  }
                }
              }
            }
          }
        }
        n279 = property on="Experiment Name" class="Str"("Value"=w549) -> ()  [unwired: 2 in, 2 out]
      }
      frame "AskDescription" {
        n280 = Unbundle By Name(w629) -> ("DataPath"=w621:path, "Description"=w630:string)
        n281 = call "AskForExperimentDescription.vi"("String Control"=w630) -> ("Experiment Name 2"=w613:string)  [unwired: 5 in, 1 out]
        n282 = property on="Experiment Name" class="Str" props=["Value"]() -> ()  [unwired: 2 in, 3 out]
        n283 = Bundle By Name(cluster=w629, "Description"=w613) -> (w631:T8)
        n284 = Build Path(base path=w621, name or relative path=path "Notes.txt") -> (appended path=w626:path)
        n285 = Concatenate Strings("Description: " ("string"), w613, "\r") -> (w610:string)
        n286 = Open/Create/Replace File(file path (use dialog)=w626, error in=w623, operation (0:open)=T23."open or create") -> (refnum out=w615:refnum<file>, error out=w617:errorcluster)  [unwired: 3 in, 1 out]
        n287 = Get File Size(file=w615, error in=w617) -> (refnum out=w619:refnum<file>, size (in bytes)=w618:i64, 0:w620:errorcluster)
        n288 = Set File Position(offset (in bytes) (0)=w618, refnum=w619, error in=w620) -> (refnum out=w614:refnum<file>, error out=w616:errorcluster)  [unwired: 1 in]
        n289 = Write to Text File(file (use dialog)=w614, text=w610, error in=w616) -> (refnum out=w628:refnum<file>, error out=w625:errorcluster)  [unwired: 1 in, 1 out]
        n290 = Close File(refnum=w628, error in=w625) -> (error out=w622:errorcluster)  [unwired: 1 out]
      }
      frame "AskPostNotes" {
        n291 = Unbundle By Name(w656) -> ("DataPath"=w645:path, "Post Notes"=w657:string)  [unwired: 1 out]
        n292 = property on="Experiment Name" class="Str" props=["Value"]() -> ()  [unwired: 2 in, 3 out]
        n293 = call "AskForExperimentPostNotes.vi"("String Control"=w657) -> ("Experiment Name 2"=w635:string)  [unwired: 5 in, 1 out]
        n294 = Build Path(base path=w645, name or relative path=path "Notes.txt") -> (appended path=w650:path)
        n295 = Open/Create/Replace File(file path (use dialog)=w650, error in=w647, operation (0:open)=T23."open or create") -> (refnum out=w640:refnum<file>, error out=w642:errorcluster)  [unwired: 3 in, 1 out]
        n296 = Bundle By Name(cluster=w656, "Post Notes"=w635) -> (w655:T8)
        n297 = Get File Size(file=w640, error in=w642) -> (refnum out=w639:refnum<file>, size (in bytes)=w638:i64, 0:w641:errorcluster)
        n298 = Set File Position(offset (in bytes) (0)=w638, refnum=w639, error in=w641) -> (refnum out=w644:refnum<file>, error out=w643:errorcluster)  [unwired: 1 in]
        n299 = Concatenate Strings("Post Notes: " ("string"), w635, "\r") -> (w634:string)
        n300 = Write to Text File(file (use dialog)=w644, text=w634, error in=w643) -> (refnum out=w652:refnum<file>, error out=w649:errorcluster)  [unwired: 1 in, 1 out]
        n301 = Close File(refnum=w652, error in=w649) -> (error out=w648:errorcluster)  [unwired: 1 out]
      }
      frame "Rendezvous" {
        n302 = control-ref of="Outputs"() -> (w683:refnum<vi>)
        n303 = property on="Property Node" class="Clust (strict)"(reference=w683) -> ("Value"=w688:T5)  [unwired: 1 in, 2 out]
        n304 = control-ref of="Input Channels"() -> (w689:refnum<vi>)
        n305 = Unbundle By Name(w688) -> ("AO0Enable"=w687:bool, "AO1Enable"=w686:bool, "AO3Enable"=w685:bool)
        n306 = property on="Synchronize Camera and Data" class="Bool (strict)"() -> ("Value"=w659:bool)  [unwired: 2 in, 2 out]
        n307 = property on="Use Camera" class="Bool (strict)"() -> ("Value"=w661:bool)  [unwired: 2 in, 2 out]
        n308 = property on="Property Node" class="DAQmxName"(reference=w689) -> ("Value"=w691:string)  [unwired: 1 in, 2 out]
        n309 = Or(x=w687, y=w686) -> (x .or. y?=w684:bool)
        n310 = Not Equal?(x=w691, y=tag "" ("Input Channels")) -> (x != y?=w667:bool)
        n311 = Or(x=w684, y=w685) -> (x .or. y?=w666:bool)
        n312 = And(x=w661, y=w659) -> (x .and. y?=w660:bool)
        n313 = Select(t=1.0, s=w666, f=0.0) -> (s? t:f=w675:dbl)
        n314 = Select(t=1.0, s=w660, f=0.0) -> (s? t:f=w674:dbl)
        n315 = Select(t=1.0, s=w667, f=0.0) -> (s? t:f=w676:dbl)
        n316 = Compound Arithmetic op=ADD(w676, w675, w674) -> (w673:dbl)
        n317 = call <vilib>:"Create Rendezvous.vi"("return existing (F)"=FALSE, "size (2)"=w673) -> ("rendezvous"=w669:T7)  [unwired: 3 in, 2 out]
        n318 = Or(x=w667, y=w666) -> (x .or. y?=w668:bool)
        n319 = Or(x=w668, y=w660) -> (x .or. y?=w665:bool)
        n320 = Bundle By Name(cluster=w671, "Use Camera"=w661, "Use Inputs"=w667, "Use Outputs"=w666, "rendezvous"=w669) -> (w670:T8)
        n321 = case shown="True" w665 {
          tunnel: w664 -> [w694 w695]
          tunnel: [w692 w695] -> w663
          frame False {
            n322 = Merge Errors(w694, errorcluster {"status"=FALSE, "code"=2147, "source"="No Options are selected"} ("error constant")) -> (w692:errorcluster)
          }
          frame True {
          }
        }
      }
      frame "ManageCameraButton" {
        n323 = property on="Initialize Camera" class="Bool (strict)"("Value"=TRUE ("Initialize Camera")) -> ()  [unwired: 2 in, 2 out]
      }
      frame "StartCamera" {
        n324 = Unbundle By Name(w706) -> ("Use Camera"=w708:bool, "Save Video"=w703:bool, "Use Inputs"=w704:bool, "Use Outputs"=w705:bool, "rendezvous"=w702:T7, "VideoPath"=w701:path)
        n325 = case shown="True" w708 {
          tunnel: [_ w726] -> w710
          tunnel: [_ w723] -> w709
          tunnel: w703 -> [_ w724]
          tunnel: w705 -> [_ w721]
          tunnel: w704 -> [_ w722]
          tunnel: w703 -> [_ w717]
          tunnel: w702 -> [_ w716]
          tunnel: w701 -> [_ w715]
          frame False {
          }
          frame True {
            w730 = T30 {"FPS"=30, "Exposure Time"=0.0001, "Start Trigger Source"="/Dev1/ai/StartTrigger", "Camera\nClock\nCounter"="Dev1/ctr0", "PhysicalCameraSignalLine"="/Dev1/PFI2", "Sync Type"=""}  # Trigger Settings
            w740 = T31 {"SyncStart"=TRUE, "ConfirmTDMSOptimizations"=TRUE, "ConfirmTDMSDisableBuffer"=FALSE, "VideoSave"=FALSE, "rendezvous ref "=refnum, "AcStarted"=FALSE}  # Running Options
            w748 = T32 {"FileSaveLocation"=path "", "FileName"="", "VideoSuffix"="", "Codec"="", "Quality"=0, "Format"="", "AVI FPS"=0, "TimingSuffix"=""}  # FileSettings
            w751 = cluster{"Buffer":i32, "FramesPerFile":i32} {"Buffer"=10, "FramesPerFile"=100000}  # AcquisitionSettings
            w753 = tag "Dev1/ctr0"  # Camera Clock Counter
            w760 = T33 {"Pixel Format"="Mono 8", "Width"=704, "Height"=704, "Trigger Source"="Line 3", "Readout Mode"="Normal", "Session In"="cam0"}  # User Camera Settings
            n326 = property on="Synchronize Camera and Data" class="Bool (strict)"() -> ("Value"=w731:bool)  [unwired: 2 in, 2 out]
            n327 = property on="Pixel Format\n(p not supported)" class="Ring (strict)"() -> ("RingText.Text"=w754:string)  [unwired: 2 in, 2 out]
            n328 = property on="Signal Line" class="Ring (strict)"() -> ("RingText.Text"=w755:string)  [unwired: 2 in, 2 out]
            n329 = property on="Sensor readout mode\n(Fast Decreases Quality)" class="Ring (strict)"() -> ("RingText.Text"=w756:string)  [unwired: 2 in, 2 out]
            n330 = property on="Camera Ref" class="IMAQdx (strict)"() -> ("Value"=w757:T2)  [unwired: 2 in, 2 out]
            n331 = property on="Image Height" class="DigNum (strict)"() -> ("Value"=w758:dbl)  [unwired: 2 in, 2 out]
            n332 = property on="Image Width" class="DigNum (strict)"() -> ("Value"=w759:dbl)  [unwired: 2 in, 2 out]
            n333 = Bundle By Name(cluster=w760, "Pixel Format"=w754, "Width"=w759, "Height"=w758, "Trigger Source"=w755, "Readout Mode"=w756, "Session In"=w757) -> (w732:T33)
            n334 = case shown="False" w717 {
              tunnel: ["None" ("RingText.Text") w762] -> w746
              frame False {
              }
              frame True {
                n335 = property on="Temporary Format\n(can be converted)" class="Enum (strict)"() -> ("RingText.Text"=w762:string)  [unwired: 2 in, 2 out]
              }
            }
            n336 = property on="Images Per File" class="DigNum (strict)"() -> ("Value"=w749:dbl)  [unwired: 2 in, 2 out]
            n337 = property on="Buffer Images" class="DigNum (strict)"() -> ("Value"=w750:dbl)  [unwired: 2 in, 2 out]
            n338 = case shown="True" w731 {
              tunnel: w722 -> [_ w771]
              tunnel: w721 -> [_ w770]
              tunnel: [tag "" ("Start Trigger Source") w769] -> w741
              tunnel: w740 -> [w765 w768]
              tunnel: [w766 w767] -> w739
              frame False {
                n339 = Bundle By Name(cluster=w765, "SyncStart"=FALSE) -> (w766:T31)
              }
              frame True {
                n340 = case shown="True" w771 {
                  tunnel: w770 -> [w775 _]
                  tunnel: [w774 tag "/Dev1/ai/StartTrigger" ("Start Trigger Source")] -> w769
                  tunnel: w768 -> [w773 w784]
                  tunnel: [w772 w785] -> w767
                  frame False {
                    n341 = case shown="False" w775 {
                      tunnel: [tag "" ("Start Trigger Source") tag "/Dev1/ao/StartTrigger" ("Start Trigger Source")] -> w774
                      tunnel: w773 -> [w779 w780]
                      tunnel: [w777 w781] -> w772
                      frame False {
                        n342 = Bundle By Name(cluster=w779, "SyncStart"=FALSE) -> (w777:T31)
                      }
                      frame True {
                        n343 = Bundle By Name(cluster=w780, "SyncStart"=TRUE) -> (w781:T31)
                      }
                    }
                  }
                  frame True {
                    n344 = Bundle By Name(cluster=w784, "SyncStart"=TRUE) -> (w785:T31)
                  }
                }
              }
            }
            n345 = Bundle By Name(cluster=w751, "Buffer"=w750, "FramesPerFile"=w749) -> (w733:cluster{"Buffer":i32, "FramesPerFile":i32})
            n346 = property on="Codec" class="Ring (strict)"() -> ("RingText.Text"=w745:string)  [unwired: 2 in, 2 out]
            n347 = property on="Experiment Name" class="Str"() -> ("Value"=w742:string)  [unwired: 2 in, 2 out]
            n348 = property on="Video File Suffix" class="Str"() -> ("Value"=w743:string)  [unwired: 2 in, 2 out]
            n349 = property on="Timing File Suffix" class="Str"() -> ("Value"=w714:string)  [unwired: 2 in, 2 out]
            n350 = property on="Encoding Quality" class="DigNum (strict)"() -> ("Value"=w744:dbl)  [unwired: 2 in, 2 out]
            n351 = property on="Confirm File Write Optimizations (TDMS)" class="Bool (strict)"() -> ("Value"=w738:bool)  [unwired: 2 in, 2 out]
            n352 = property on="Confirm Disable Buffering (advanced TDMS)" class="Bool (strict)"() -> ("Value"=w737:bool)  [unwired: 2 in, 2 out]
            n353 = case shown="True" w731 {
              tunnel: [T25."NoSync" ("Sync Type") w789] -> w729
              frame False {
              }
              frame True {
                n354 = property on="Time Stamp\n Position" class="Enum (strict)"() -> ("RingText.Text"=w790:string)  [unwired: 2 in, 2 out]
                n355 = case shown="\"Exposure Center\", Default" w790 {
                  tunnel: [T25."Exposure Start" ("Sync Type") T25."Exposure End" ("Sync Type") T25."Exposure Center" ("Sync Type")] -> w789
                  frame "Exposure Beginning" {
                  }
                  frame "Exposure End" {
                  }
                  frame "Exposure Center", Default {
                  }
                }
              }
            }
            n356 = Bundle By Name(cluster=w739, "ConfirmTDMSOptimizations"=w738, "ConfirmTDMSDisableBuffer"=w737, "VideoSave"=w724, "rendezvous ref"=w716) -> (w725:T31)
            n357 = property on="Exposure (us)" class="DigNum (strict)"() -> ("Value"=w720:dbl)  [unwired: 2 in, 2 out]
            n358 = Divide(x=w720, y=1000000.0) -> (x/y=w718:dbl)
            n359 = property on="FPS" class="DigNum (strict)"() -> ("Value"=w747:dbl)  [unwired: 2 in, 2 out]
            n360 = Bundle By Name(cluster=w748, "FileSaveLocation"=w715, "FileName"=w742, "VideoSuffix"=w743, "Codec"=w745, "Quality"=w744, "Format"=w746, "AVI FPS"=w747, "TimingSuffix"=w714) -> (w734:T32)
            n361 = property on="Camera Signal Output Port" class="DAQmxName"() -> ("Value"=w752:string)  [unwired: 2 in, 2 out]
            n362 = property on="Update Viewport Every N Frames" class="DigNum (strict)"() -> ("Value"=w736:dbl)  [unwired: 2 in, 2 out]
            n363 = call <extravilib>:"Write.vi"("element"=w725) -> ("channel"=w723:T34)  [unwired: 8 in, 2 out]
            n364 = Format Into String(w729) -> (resulting string=w728:string)  [unwired: 3 in, 1 out]
            n365 = Bundle By Name(cluster=w730, "FPS"=w747, "Exposure Time"=w718, "Start Trigger Source"=w741, "Camera\nClock\nCounter"=w753, "PhysicalCameraSignalLine"=w752, "Sync Type"=w728) -> (w735:T30)
            n366 = Bundle By Name(cluster=T24 {"User Camera Settings"={"Pixel Format"="Mono 8", "Width"=1280, "Height"=1024, "Trigger Source"="Line 3", "Readout Mode"="Normal", "Session In"="cam0"}, "Trigger Settings"={"FPS"=30, "Exposure Time"=0.0001, "Start Trigger Source"="/Dev1/ai/StartTrigger", "Camera\nClock\nCounter"="Dev1/ctr0", "PhysicalCameraSignalLine"="/Dev1/PFI2", "Sync Type"=""}, "Camera Attributes"={"Exposure Start Delay"=0.0, "Model"="", "Make"=""}, "AcquisitionSettings"={"Buffer"=10, "FramesPerFile"=100000}, "DisplayEveryNFrames"=30, "FileSettings"={"FileSaveLocation"=path "", "FileName"="", "VideoSuffix"="", "Codec"="", "Quality"=0, "Format"="", "AVI FPS"=0, "TimingSuffix"=""}}, "User Camera Settings"=w732, "Trigger Settings"=w735, "AcquisitionSettings"=w733, "FileSettings"=w734, "DisplayEveryNFrames"=w736) -> (w727:T24)
            n367 = call <extravilib>:"Write.vi"("element"=w727) -> ("channel"=w726:T35)  [unwired: 8 in, 2 out]
          }
        }
      }
      frame "StartOutput" {
        n368 = Unbundle By Name(w797) -> ("Use Outputs"=w803:bool, "Use Inputs"=w802:bool, "rendezvous"=w795:T7, "DataPath"=w794:path)
        n369 = case shown="False" w803 {
          tunnel: w802 -> [_ w837]
          tunnel: [_ w819] -> w801
          tunnel: [_ w818] -> w800
          tunnel: w795 -> [_ w817]
          tunnel: w794 -> [_ w810]
          frame False {
          }
          frame True {
            w811 = T36 {"Path"=path "E:/Jacob", "File"="Test3", "FileFormat"=enum."TDMS", "FileSuffix"="_Data_Output", "Multiple Time Columns"=TRUE}  # FileSettings
            w836 = T37 {"PreviousInfo"=[{"FinalSamplePhase"=0.0, "LastTf"=timestamp(0 s since 1904-01-01), "LastSelectedPhase"=0.0}, {"FinalSamplePhase"=0.0, "LastTf"=timestamp(0 s since 1904-01-01), "LastSelectedPhase"=0.0}, {"FinalSamplePhase"=0.0, "LastTf"=timestamp(0 s since 1904-01-01), "LastSelectedPhase"=0.0}], "SyncStart"=FALSE, "Leader"=FALSE, "Started?"=FALSE, "AfterErrorCheck"="", "rendezvous ref "=refnum, "AcStarted"=FALSE}  # Running Options
            w833 = T38 {"physical channels"="Dev1/ao0:2", "source"="OnboardClock", "Start Trigger"="/Dev1/ai/StartTrigger", "StartTriggered"=TRUE}  # Physical Settings
            w847 = T39 {"NumberOfSamples"=10000, "Sample Rate"=50000, "SampleBuffer"=100000}  # GenerationSettings
            n370 = case shown="True" w837 {
              tunnel: [w853 w857] -> w835
              tunnel: [w852 w858] -> w834
              tunnel: [w851 w860] -> w831
              tunnel: [w850 w859] -> w830
              frame False {
                w852 = TRUE  # Leader
                w850 = FALSE  # StartTriggered
                w851 = tag ""  # Start Trigger
                n371 = property on="Synchronize Camera and Data" class="Bool (strict)"() -> ("Value"=w854:bool)  [unwired: 2 in, 2 out]
                n372 = case shown="True" w854 {
                  tunnel: [w855 w856] -> w853
                  frame False {
                    w855 = FALSE  # SyncStart
                  }
                  frame True {
                    w856 = TRUE  # SyncStart
                  }
                }
              }
              frame True {
                w857 = TRUE  # SyncStart
                w858 = FALSE  # Leader
                w859 = TRUE  # StartTriggered
                w860 = tag "/Dev1/ai/StartTrigger"  # Start Trigger
              }
            }
            n373 = property on="Outputs" class="Clust (strict)"() -> ("Value"=w843:T5)  [unwired: 2 in, 2 out]
            n374 = property on="Sample Rate" class="DigNum (strict)"() -> ("Value"=w846:dbl)  [unwired: 2 in, 2 out]
            n375 = property on="Sample Buffer" class="DigNum (strict)"() -> ("Value"=w845:dbl)  [unwired: 2 in, 2 out]
            n376 = property on="Samples to Generate" class="DigNum (strict)"() -> ("Value"=w844:dbl)  [unwired: 2 in, 2 out]
            n377 = Unbundle By Name(w843) -> ("AO0Enable"=w842:bool, "AO1Enable"=w841:bool, "AO3Enable"=w840:bool, "AO0Name"=w829:string, "AO1Name"=w828:string, "AO2Name"=w827:string)
            n378 = Bundle By Name(cluster=w847, "NumberOfSamples"=w844, "Sample Rate"=w846, "SampleBuffer"=w845) -> (w823:T39)
            n379 = Build Array(w829, w828, w827) -> (w826:string[])
            n380 = Build Array(w842, w841, w840) -> (w839:bool[])
            n381 = for {
              tunnel: w839 -> [w867] mode=indexing
              tunnel: w826 -> [w863] mode=indexing
              shift-right: [w865] -> w816
              shift-left: string[] [] -> [w864]
              shift-right: [w862] -> w815
              shift-left: string[] [] -> [w861]
              i -> [w868]
              n382 = Number To Decimal String(number=w868) -> (decimal integer string=w869:string)  [unwired: 1 in]
              n383 = Concatenate Strings("Dev1/ao", w869) -> (w866:string)
              n384 = case shown="False" w867 {
                tunnel: w866 -> [_ w878]
                tunnel: [w872 w877] -> w865
                tunnel: w864 -> [w872 w876]
                tunnel: w863 -> [_ w875]
                tunnel: [w871 w874] -> w862
                tunnel: w861 -> [w871 w873]
                frame False {
                }
                frame True {
                  n385 = Build Array (concatenate)(w873, w875) -> (w874:string[])
                  n386 = Build Array (concatenate)(w876, w878) -> (w877:string[])
                }
              }
            }
            n387 = call <vilib>:"1D String Array to Delimited String.vi"("delimiter"=",", "string array"=w816) -> ("delimited string"=w832:string)  [unwired: 9 in]
            n388 = call <vilib>:"1D String Array to Delimited String.vi"("delimiter"=",", "string array"=w815) -> ("delimited string"=w822:string)  [unwired: 9 in]
            n389 = property on="Data File Format" class="Bool (strict)"() -> ("Value"=w808:bool)  [unwired: 2 in, 2 out]
            n390 = case shown="False" w808 {
              tunnel: [enum16{"TDMS", "CSV"}."TDMS" ("FileFormat") enum16{"TDMS", "CSV"}."CSV" ("FileFormat")] -> w807
              frame False {
              }
              frame True {
              }
            }
            n391 = Bundle By Name(cluster=w833, "physical channels"=w832, "Start Trigger"=w831, "StartTriggered"=w830) -> (w824:T38)
            n392 = property on="Output Data File Suffix" class="Str"() -> ("Value"=w806:string)  [unwired: 2 in, 2 out]
            n393 = Bundle By Name(cluster=w836, "Leader"=w834, "SyncStart"=w835, "rendezvous ref"=w817) -> (w820:T37)
            n394 = property on="Experiment Name" class="Str"() -> ("Value"=w809:string)  [unwired: 2 in, 2 out]
            n395 = property on="CSV\nMultiple Time Columns" class="Bool (strict)"() -> ("Value"=w805:bool)  [unwired: 2 in, 2 out]
            n396 = Bundle By Name(cluster=w811, "Path"=w810, "File"=w809, "FileFormat"=w807, "FileSuffix"=w806, "Multiple Time Columns"=w805) -> (w804:T36)
            n397 = Bundle By Name(cluster=T26 {"Physical Settings"={"physical channels"="Dev1/ao0:2", "source"="OnboardClock", "Start Trigger"="/Dev1/ai/StartTrigger", "StartTriggered"=TRUE}, "GenerationSettings"={"NumberOfSamples"=10000, "Sample Rate"=50000, "SampleBuffer"=100000}, "Channel Names"="", "FileSettings"={"Path"=path "E:/Jacob", "File"="Test3", "FileFormat"=enum."TDMS", "FileSuffix"="_Data_Output", "Multiple Time Columns"=TRUE}}, "Physical Settings"=w824, "GenerationSettings"=w823, "Channel Names"=w822, "FileSettings"=w804) -> (w821:T26)
            n398 = call <extravilib>:"Write.vi"("element"=w821) -> ("channel"=w819:T40)  [unwired: 8 in, 2 out]
            n399 = call <extravilib>:"Write.vi"("element"=w820) -> ("channel"=w818:T41)  [unwired: 8 in, 2 out]
          }
        }
      }
      frame "StartInput" {
        n400 = Unbundle By Name(w881) -> ("Use Inputs"=w889:bool, "rendezvous"=w887:T7, "Use Camera"=w885:bool, "Use Outputs"=w886:bool, "DataPath"=w879:path)
        n401 = case shown="True" w889 {
          tunnel: w887 -> [_ w910]
          tunnel: w886 -> [_ w907]
          tunnel: w885 -> [_ w904]
          tunnel: [_ w901] -> w884
          tunnel: [_ w900] -> w883
          tunnel: w879 -> [_ w895]
          frame False {
          }
          frame True {
            w897 = T36 {"Path"=path "E:/Jacob", "File"="Test3", "FileFormat"=enum."TDMS", "FileSuffix"="_Data_Output", "Multiple Time Columns"=TRUE}  # FileSettings
            w911 = T42 {"SyncStart"=TRUE, "Leader"=TRUE, "Started?"=FALSE, "AfterErrorCheck"="", "rendezvous ref"=refnum, "AcStarted"=FALSE}  # Running Options
            w922 = T43 {"SyncType"=enum."NoSync", "Frame Rate"=30.0, "Sample Rate"=50000.0, "Sample BufferSize"=100000}  # Acquisition Settings
            w926 = T38 {"physical channels"="Dev1/ai0:2", "source"="OnboardClock", "Start Trigger"="", "StartTriggered"=FALSE}  # Physical Settings
            n402 = property on="Synchronize Camera and Data" class="Bool (strict)"() -> ("Value"=w921:bool)  [unwired: 2 in, 2 out]
            n403 = property on="Channel Names" class="Arr (strict)"() -> ("Value"=w899:string[])  [unwired: 2 in, 2 out]
            n404 = case shown="True" w921 {
              tunnel: [w938 w939] -> w920
              frame False {
                w938 = enum16{"NoSync", "Sync"}."NoSync"  # SyncType
              }
              frame True {
                w939 = enum16{"NoSync", "Sync"}."Sync"  # SyncType
              }
            }
            n405 = property on="Sample Buffer" class="DigNum (strict)"() -> ("Value"=w917:dbl)  [unwired: 2 in, 2 out]
            n406 = property on="Sample Rate" class="DigNum (strict)"() -> ("Value"=w918:dbl)  [unwired: 2 in, 2 out]
            n407 = property on="FPS" class="DigNum (strict)"() -> ("Value"=w919:dbl)  [unwired: 2 in, 2 out]
            n408 = property on="Input Channels" class="DAQmxName"() -> ("Value"=w925:string)  [unwired: 2 in, 2 out]
            n409 = for {
              tunnel: w899 -> [w932] mode=indexing
              tunnel: [w929] -> w898 mode=indexing
              n410 = Search and Replace String(input string=w932, search string="/", replace string="") -> (result string=w929:string)  [unwired: 5 in, 3 out]
            }
            n411 = Bundle By Name(cluster=w926, "physical channels"=w925, "Start Trigger"=tag "", "StartTriggered"=FALSE) -> (w914:T38)
            n412 = Bundle By Name(cluster=w922, "SyncType"=w920, "Frame Rate"=w919, "Sample Rate"=w918, "Sample BufferSize"=w917) -> (w913:T43)
            n413 = property on="Data File Format" class="Bool (strict)"() -> ("Value"=w891:bool)  [unwired: 2 in, 2 out]
            n414 = call <vilib>:"1D String Array to Delimited String.vi"("delimiter"=",", "string array"=w898) -> ("delimited string"=w912:string)  [unwired: 9 in]
            n415 = property on="Input Data File Suffix" class="Str"() -> ("Value"=w892:string)  [unwired: 2 in, 2 out]
            n416 = case shown="False" w891 {
              tunnel: [enum16{"TDMS", "CSV"}."TDMS" ("FileFormat") enum16{"TDMS", "CSV"}."CSV" ("FileFormat")] -> w893
              frame False {
              }
              frame True {
              }
            }
            n417 = property on="CSV\nMultiple Time Columns" class="Bool (strict)"() -> ("Value"=w890:bool)  [unwired: 2 in, 2 out]
            n418 = property on="Experiment Name" class="Str"() -> ("Value"=w894:string)  [unwired: 2 in, 2 out]
            n419 = Bundle By Name(cluster=w897, "Path"=w895, "File"=w894, "FileFormat"=w893, "FileSuffix"=w892, "Multiple Time Columns"=w890) -> (w896:T36)
            n420 = property on="Synchronize Camera and Data" class="Bool (strict)"() -> ("Value"=w906:bool)  [unwired: 2 in, 2 out]
            n421 = And(x=w906, y=w904) -> (x .and. y?=w905:bool)
            n422 = case shown="True" w905 {
              tunnel: [w933 TRUE ("SyncStart")] -> w908
              tunnel: w907 -> [w934 _]
              frame False {
                n423 = case shown="True" w934 {
                  tunnel: [FALSE ("SyncStart") TRUE ("SyncStart")] -> w933
                  frame False {
                  }
                  frame True {
                  }
                }
              }
              frame True {
              }
            }
            n424 = Bundle By Name(cluster=T10 {"Physical Settings"={"physical channels"="Dev1/ai0:2", "source"="OnboardClock", "Start Trigger"="/Dev1/ai/StartTrigger", "StartTriggered"=FALSE}, "Acquisition Settings"={"SyncType"=enum."NoSync", "Frame Rate"=30.0, "Sample Rate"=50000.0, "Sample BufferSize"=100000}, "Channel Names"="", "task in"="", "FileSettings"={"Path"=path "E:/Jacob", "File"="Test3", "FileFormat"=enum."TDMS", "FileSuffix"="_Data_Output", "Multiple Time Columns"=TRUE}}, "Physical Settings"=w914, "Acquisition Settings"=w913, "Channel Names"=w912, "FileSettings"=w896) -> (w903:T10)
            n425 = call <extravilib>:"Write.vi"("element"=w903) -> ("channel"=w901:T44)  [unwired: 8 in, 2 out]
            n426 = Bundle By Name(cluster=w911, "SyncStart"=w908, "Leader"=TRUE, "rendezvous ref"=w910) -> (w902:T42)
            n427 = call <extravilib>:"Write.vi"("element"=w902) -> ("channel"=w900:T45)  [unwired: 8 in, 2 out]
          }
        }
      }
      frame "AcquisitionGUI" {
        w945 = T22."Disabled and Grayed Out" ("Disabled")
        n428 = property on="Cluster - Borderless" class="Clust (strict)"("DisabledEnum"=w945) -> ()  [unwired: 2 in, 2 out]
        n429 = property on="Channel Names" class="Arr (strict)"("DisabledEnum"=w945) -> ()  [unwired: 2 in, 2 out]
        n430 = property on="Input Channels" class="DAQmxName"("DisabledEnum"=w945) -> ()  [unwired: 2 in, 2 out]
        n431 = property on="Sample Rate" class="DigNum (strict)"("DisabledEnum"=w945) -> ()  [unwired: 2 in, 2 out]
        n432 = property on="Samples to Generate" class="DigNum (strict)"("DisabledEnum"=w945) -> ()  [unwired: 2 in, 2 out]
        n433 = property on="Sample Buffer" class="DigNum (strict)"("DisabledEnum"=w945) -> ()  [unwired: 2 in, 2 out]
        n434 = property on="Initialize Camera" class="Bool (strict)"("DisabledEnum"=w945) -> ()  [unwired: 2 in, 2 out]
        n435 = property on="Exposure (us)" class="DigNum (strict)"("DisabledEnum"=w945) -> ()  [unwired: 2 in, 2 out]
        n436 = property on="AO1Enable" class="Bool (strict)"("DisabledEnum"=w945) -> ()  [unwired: 2 in, 2 out]
        n437 = property on="FPS" class="DigNum (strict)"("DisabledEnum"=w945) -> ()  [unwired: 2 in, 2 out]
        n438 = property on="AO3Enable" class="Bool (strict)"("DisabledEnum"=w945) -> ()  [unwired: 2 in, 2 out]
        n439 = property on="Use Camera" class="Bool (strict)"("DisabledEnum"=w945) -> ()  [unwired: 2 in, 2 out]
        n440 = property on="Save Video" class="Bool (strict)"("DisabledEnum"=w945) -> ()  [unwired: 2 in, 2 out]
        n441 = property on="AO0Enable" class="Bool (strict)"("DisabledEnum"=w945) -> ()  [unwired: 2 in, 2 out]
        n442 = Unbundle By Name(w943) -> ("Use Camera"=w942:bool, "Use Inputs"=w940:bool, "Use Outputs"=w941:bool)
        n443 = flat-sequence {
          tunnel: w950 -> [w956]
          tunnel: w949 -> [w955]
          tunnel: w948 -> [w954]
          tunnel: w942 -> [w953]
          tunnel: w941 -> [w952]
          tunnel: w940 -> [w951]
          frame #0 {
            n444 = while {
              tunnel: w955 -> [w968]
              tunnel: w954 -> [w967]
              tunnel: w956 -> [w966]
              tunnel: w953 -> [w959]
              tunnel: w952 -> [w958]
              tunnel: w951 -> [w957]
              stop <- w960 stop-if-true
              n445 = case shown="False" w957 {
                tunnel: w968 -> [_ w973]
                tunnel: [TRUE w972] -> w964
                frame False {
                }
                frame True {
                  n446 = call <extravilib>:"Read.vi"("channel"=w973) -> ("element"=w971:string)  [unwired: 1 in, 1 out]
                  n447 = Equal?(x=w971, y="Acquire") -> (x = y?=w972:bool)
                }
              }
              n448 = case shown="False" w958 {
                tunnel: w967 -> [_ w978]
                tunnel: [TRUE w977] -> w962
                frame False {
                }
                frame True {
                  n449 = call <extravilib>:"Read.vi"("channel"=w978) -> ("element"=w976:string)  [unwired: 1 in, 1 out]
                  n450 = Equal?(x=w976, y="Generate") -> (x = y?=w977:bool)
                }
              }
              n451 = case shown="True" w959 {
                tunnel: w966 -> [_ w983]
                tunnel: [TRUE w982] -> w963
                frame False {
                }
                frame True {
                  n452 = call <extravilib>:"Read.vi"("channel"=w983) -> ("element"=w981:string)  [unwired: 1 in, 1 out]
                  n453 = Equal?(x=w981, y="Acquire") -> (x = y?=w982:bool)
                }
              }
              n454 = And(x=w962, y=w963) -> (x .and. y?=w961:bool)
              n455 = And(x=w964, y=w961) -> (x .and. y?=w960:bool)
              n456 = Wait (ms)(milliseconds to wait=u32 10) -> ()  [unwired: 1 out]
            }
          }
          frame #1 {
            n457 = property on="Re/Start Acquisition" class="Bool (strict)"("Value"=FALSE) -> ()  [unwired: 2 in, 2 out]
          }
        }
      }
      frame "CheckStatus" {
        n458 = Unbundle By Name(w986) -> ("Use Camera"=w999:bool, "Use Inputs"=w998:bool, "Use Outputs"=w997:bool)
        n459 = case shown="True" w998 {
          tunnel: w1001 -> [_ w1025]
          tunnel: [FALSE w1024] -> w996
          frame False {
          }
          frame True {
            n460 = call <extravilib>:"Read.vi"("channel"=w1025) -> ("element"=w1023:string)  [unwired: 1 in, 1 out]
            n461 = Equal?(x=w1023, y="Idle") -> (x = y?=w1024:bool)
          }
        }
        n462 = case shown="False" w997 {
          tunnel: w1002 -> [_ w1030]
          tunnel: [FALSE w1029] -> w994
          frame False {
          }
          frame True {
            n463 = call <extravilib>:"Read.vi"("channel"=w1030) -> ("element"=w1028:string)  [unwired: 1 in, 1 out]
            n464 = Equal?(x=w1028, y="Idle") -> (x = y?=w1029:bool)
          }
        }
        n465 = case shown="True" w999 {
          tunnel: w1000 -> [_ w1035]
          tunnel: [FALSE w1034] -> w995
          frame False {
          }
          frame True {
            n466 = call <extravilib>:"Read.vi"("channel"=w1035) -> ("element"=w1033:string)  [unwired: 1 in, 1 out]
            n467 = Equal?(x=w1033, y="Idle") -> (x = y?=w1034:bool)
          }
        }
        n468 = Or(x=w994, y=w995) -> (x .or. y?=w993:bool)
        n469 = Or(x=w996, y=w993) -> (x .or. y?=w992:bool)
        n470 = case shown="False" w992 {
          tunnel: ["Idle" w1014] -> w991
          tunnel: [w1003 FALSE] -> w990
          tunnel: w988 -> [w1006 w1016]
          tunnel: [w1006 w1015] -> w987
          tunnel: w986 -> [w1005 w1012]
          tunnel: [w1004 w1010] -> w985
          frame False {
            w1003 = FALSE
            n471 = Bundle By Name(cluster=w1005, "StopDueToError"=w1003) -> (w1004:T8)
          }
          frame True {
            w1014 = "StopAcquisition"
            n472 = property on="BufferWasFull" class="Bool (strict)"() -> ("Value"=w1009:bool)  [unwired: 2 in, 2 out]
            n473 = case shown="True" w1009 {
              tunnel: ["Aquisition has stopped for unknown reason" ("StopMessage") "Aquisition has stopped due to full buffer" ("StopMessage")] -> w1011
              frame False {
              }
              frame True {
                n474 = property on="BufferWasFull" class="Bool (strict)"("Value"=FALSE ("BufferWasFull")) -> ()  [unwired: 2 in, 2 out]
              }
            }
            n475 = Bundle By Name(cluster=w1016, "DefaultAction"=w1014, "NextAction"=w1014, "ActionString"="StopAcquisition,StopWarning") -> (w1015:T11)
            n476 = Bundle By Name(cluster=w1012, "StopMessage"=w1011, "StopDueToError"=TRUE) -> (w1010:T8)
          }
        }
      }
      frame "CheckHardDrive" {
        # "If less than 10 Gb on disk, stop"
        n477 = Unbundle By Name(w1037) -> ("VideoPath"=w1060:path, "DataPath"=w1059:path, "LastSizeVid"=w1054:dbl, "Last Time"=w1055:dbl)  [unwired: 1 out]
        n478 = Greater Than 0?(x=w1055) -> ()  [unwired: 1 out]
        n479 = Get Volume Info(11:w1060) -> (1:w1045:i64, 5:w1058:path)  [unwired: 1 in, 4 out]
        n480 = Get Volume Info(11:w1059) -> (1:w1044:i64, 5:w1057:path)  [unwired: 1 in, 4 out]
        n481 = call "High Resolution Timer Helper.vi"("Previous Time"=w1055) -> ("Time Difference (ms)"=w1047:dbl, "Current Time"=w1046:dbl)  [unwired: 8 in, 1 out]
        n482 = Equal?(x=w1058, y=w1057) -> (x = y?=w1056:bool)
        n483 = Divide(x=w1047, y=1000.0) -> (x/y=w1053:dbl)
        n484 = case shown="True" w1056 {
          tunnel: w1053 -> [_ w1080]
          tunnel: w1054 -> [_ w1075]
          tunnel: w1045 -> [w1074 w1076]
          tunnel: [w1074 w1076] -> w1048
          frame False {
          }
          frame True {
            n485 = Subtract(x=w1075, y=w1076) -> (x-y=w1081:dbl)
            n486 = Divide(x=w1081, y=w1080) -> (x/y=w1082:dbl)
            n487 = Divide(x=w1076, y=w1082) -> (x/y=w1079:dbl)
            n488 = Divide(x=w1079, y=60.0) -> (x/y=w1078:dbl)
            n489 = property on="Video Space Remaining (min)" class="DigNum (strict)"("Value"=w1078) -> ()  [unwired: 2 in, 2 out]
            n490 = property on="Data Space Remaining (min)" class="DigNum (strict)"("Value"=w1078) -> ()  [unwired: 2 in, 2 out]
          }
        }
        n491 = Max & Min(x=w1045, y=w1044) -> (min(x,y)=w1042:i64)  [unwired: 1 out]
        n492 = Greater?(x=w1042, y=i64 10000000000) -> (0:w1043:bool)
        n493 = case shown="False" w1043 {
          tunnel: [w1064 "Idle"] -> w1051
          tunnel: [FALSE FALSE] -> w1040
          tunnel: w1039 -> [w1068 w1071]
          tunnel: [w1067 w1071] -> w1038
          tunnel: w1037 -> [w1063 w1070]
          tunnel: [w1061 w1070] -> w1036
          frame False {
            w1064 = "StopAcquisition" ("DefaultAction")
            n494 = Bundle By Name(cluster=w1068, "DefaultAction"=w1064, "NextAction"="StopAcquisition", "ActionString"="StopAcquisition,StopWarning") -> (w1067:T11)
            n495 = Bundle By Name(cluster=w1063, "StopMessage"="Acquisition Stopped because not enough space on drive.\n10 Gb required for acquisition.\nPlease back up and remove data." ("message")) -> (w1061:T8)
          }
          frame True {
          }
        }
        n496 = Bundle By Name(cluster=w1036, "LastSizeVid"=w1048, "Last Time"=w1046, "LastSizeData"=w1044) -> (w1049:T8)
      }
      frame "StopWarning" {
        (unwired) "Acquisition Stopped because not enough space on drive.\n10 Gb required for acquisition.\nPlease back up and remove data." ("message")
        n497 = Unbundle By Name(w1084) -> ("StopMessage"=w1083:string)
        n498 = call "oneButtonTimeout.vi"("message"=w1083) -> ()  [unwired: 1 in, 1 out]
        n499 = case shown="True" "Send email on non-user-initiated stop" {
          tunnel: "Recipients" -> [_ w1091]
          tunnel: w1083 -> [_ w1090]
          frame False {
          }
          frame True {
            n500 = call "Send Email"("Message"=w1090, "Subject"=w1090, "Recipients"=w1091) -> ()  [unwired: 8 in, 1 out]
          }
        }
      }
      frame "UpdateVideoControlExFPS" {
        n501 = property on="Exposure (us)" class="DigNum (strict)"(error in=w1094) -> (error out=w1093:errorcluster, "Value"=w1098:dbl)  [unwired: 1 in, 1 out]
        n502 = property on="FPS" class="DigNum (strict)"(error in=w1094) -> (error out=w1097:errorcluster, "Value"=w1099:dbl)  [unwired: 1 in, 1 out]
        n503 = property on="Exposure (us)" class="DigNum (strict)"(error in=w1093, "Value"=w1098) -> (error out=w1092:errorcluster)  [unwired: 1 in, 1 out]
        n504 = property on="FPS" class="DigNum (strict)"(error in=w1097, "Value"=w1099) -> (error out=w1095:errorcluster)  [unwired: 1 in, 1 out]
        n505 = Merge Errors(w1095, w1092) -> (w1096:errorcluster)
      }
      frame "UpdateFPControlExFPS" {
        n506 = property on="Exposure (us)" class="DigNum (strict)"(error in=w1106) -> (error out=w1107:errorcluster, "Value"=w1112:dbl)  [unwired: 1 in, 1 out]
        n507 = property on="FPS" class="DigNum (strict)"(error in=w1106) -> (error out=w1111:errorcluster, "Value"=w1113:dbl)  [unwired: 1 in, 1 out]
        n508 = property on="FPS" class="DigNum (strict)"(error in=w1111, "Value"=w1113) -> (error out=w1105:errorcluster)  [unwired: 1 in, 1 out]
        n509 = property on="Exposure (us)" class="DigNum (strict)"(error in=w1107, "Value"=w1112) -> (error out=w1103:errorcluster)  [unwired: 1 in, 1 out]
        n510 = Merge Errors(w1105, w1103) -> (w1104:errorcluster)
      }
      frame "StopAcquisition" {
        n511 = Get Date/Time In Seconds() -> (seconds since 1Jan1904=w1121:timestamp)
        n512 = property on="Recipients" class="Str"() -> ("Value"=w1124:string)  [unwired: 2 in, 2 out]
        n513 = while {
          tunnel: [w1140] -> w1123
          tunnel: w1122 -> [w1145]
          tunnel: w1121 -> [w1143]
          tunnel: 360.0 ("Time Target (s)") -> [w1141]
          stop <- w1145 stop-if-true
          n514 = Get Date/Time In Seconds() -> (seconds since 1Jan1904=w1142:timestamp)
          n515 = Subtract(x=w1142, y=w1143) -> (x-y=w1139:dbl)
          n516 = Wait (ms)(milliseconds to wait=u32 10) -> ()  [unwired: 1 out]
          n517 = Less?(x=w1141, y=w1139) -> (x < y?=w1140:bool)
        }
        n518 = Unbundle By Name(w1116) -> ("StopMessage"=w1117:string)
        n519 = flat-sequence {
          tunnel: [w1153] -> w1130
          tunnel: w1116 -> [w1152]
          tunnel: [w1150] -> w1115
          tunnel: w1134 -> [w1157]
          tunnel: w1133 -> [w1156]
          tunnel: w1132 -> [w1155]
          tunnel: [w1177] -> w1131
          tunnel: [w1175] -> w1126
          tunnel: w1116 -> [w1173]
          tunnel: [w1171] -> w1125
          tunnel: w1131 -> [w1181]
          tunnel: w1130 -> [w1179]
          tunnel: [TRUE] -> w1122
          frame #0 {
            n520 = Unbundle By Name(w1152) -> ("StopDueToError"=w1149:bool, "Acquiring"=w1151:bool)
            n521 = Not(x=w1149) -> (.not. x?=w1148:bool)
            n522 = call <extravilib>:"Write.vi"("element"=TRUE) -> ("channel"=w1153:T27)  [unwired: 1 out]
            n523 = And(x=w1148, y=w1151) -> (x .and. y?=w1150:bool)
          }
          frame #1 {
            n524 = while {
              tunnel: w1157 -> [w1170]
              tunnel: w1156 -> [w1169]
              tunnel: w1155 -> [w1168]
              stop <- w1158 stop-if-true
              w1159 = "Idle"
              n525 = call <extravilib>:"Read.vi"("channel"=w1168) -> ("element"=w1160:string)  [unwired: 1 in, 1 out]
              n526 = call <extravilib>:"Read.vi"("channel"=w1170) -> ("element"=w1162:string)  [unwired: 1 in, 1 out]
              n527 = call <extravilib>:"Read.vi"("channel"=w1169) -> ("element"=w1161:string)  [unwired: 1 in, 1 out]
              n528 = Equal?(x=w1160, y=w1159) -> (x = y?=w1165:bool)
              n529 = Equal?(x=w1161, y=w1159) -> (x = y?=w1164:bool)
              n530 = Equal?(x=w1162, y=w1159) -> (x = y?=w1166:bool)
              n531 = And(x=w1164, y=w1165) -> (x .and. y?=w1163:bool)
              n532 = And(x=w1166, y=w1163) -> (x .and. y?=w1158:bool)
              n533 = Wait (ms)(milliseconds to wait=u32 10) -> ()  [unwired: 1 out]
            }
          }
          frame #2 {
            w1178 = TRUE  # Reset
            n534 = Bundle By Name(cluster=w1173, "Acquiring"=FALSE) -> (w1171:T8)
            n535 = call <extravilib>:"Write.vi"("element"=errorcluster {"status"=FALSE, "code"=0, "source"=""}) -> ("channel"=w1175:T46)  [unwired: 8 in, 2 out]
            n536 = Wait (ms)(milliseconds to wait=u32 100) -> ()  [unwired: 1 out]
            n537 = call <extravilib>:"Write.vi"("element"=w1178) -> ("channel"=w1177:T27)  [unwired: 1 out]
          }
          frame #3 {
            w1182 = FALSE  # Reset
            n538 = call <extravilib>:"Write.vi"("element"=w1182) -> ("channel"=w1181:T27)  [unwired: 1 out]
            n539 = call <extravilib>:"Write.vi"("element"=FALSE) -> ("channel"=w1179:T27)  [unwired: 1 out]
          }
          frame #4 {
            w1183 = FALSE
            w1185 = T22."Enabled" ("Disabled")
            n540 = property on="Data File Settings" class="Clust (strict)"("DisabledEnum"=w1185) -> ()  [unwired: 2 in, 2 out]
            n541 = property on="Sample Rate" class="DigNum (strict)"("DisabledEnum"=w1185) -> ()  [unwired: 2 in, 2 out]
            n542 = property on="Samples to Generate" class="DigNum (strict)"("DisabledEnum"=w1185) -> ()  [unwired: 2 in, 2 out]
            n543 = property on="Channel Names" class="Arr (strict)"("DisabledEnum"=w1185) -> ()  [unwired: 2 in, 2 out]
            n544 = property on="Sample Buffer" class="DigNum (strict)"("DisabledEnum"=w1185) -> ()  [unwired: 2 in, 2 out]
            n545 = property on="Input Channels" class="DAQmxName"("DisabledEnum"=w1185) -> ()  [unwired: 2 in, 2 out]
            n546 = property on="Initialize Camera" class="Bool (strict)"("Value"=w1183) -> ()  [unwired: 2 in, 2 out]
            n547 = property on="Stop Button" class="Bool (strict)"("Value"=w1183) -> ()  [unwired: 2 in, 2 out]
            n548 = property on="FPS" class="DigNum (strict)"("DisabledEnum"=w1185) -> ()  [unwired: 2 in, 2 out]
            n549 = property on="Exposure (us)" class="DigNum (strict)"("DisabledEnum"=w1185) -> ()  [unwired: 2 in, 2 out]
            n550 = property on="AO3Enable" class="Bool (strict)"("DisabledEnum"=w1185) -> ()  [unwired: 2 in, 2 out]
            n551 = property on="Initialize Camera" class="Bool (strict)"("DisabledEnum"=w1185) -> ()  [unwired: 2 in, 2 out]
            n552 = property on="Use Camera" class="Bool (strict)"("DisabledEnum"=w1185) -> ()  [unwired: 2 in, 2 out]
            n553 = property on="Cluster - Borderless" class="Clust (strict)"("DisabledEnum"=w1185) -> ()  [unwired: 2 in, 2 out]
            n554 = property on="Save Video" class="Bool (strict)"("DisabledEnum"=w1185) -> ()  [unwired: 2 in, 2 out]
            n555 = property on="AO1Enable" class="Bool (strict)"("DisabledEnum"=w1185) -> ()  [unwired: 2 in, 2 out]
            n556 = property on="AO0Enable" class="Bool (strict)"("DisabledEnum"=w1185) -> ()  [unwired: 2 in, 2 out]
            n557 = property on="Shutting\nDown" class="Bool (strict)"("Value"=w1183) -> ()  [unwired: 2 in, 2 out]
          }
        }
        n558 = Concatenate Strings("Labview Unable to Stop acquisition and shut down" ("Subject"), w1117) -> (w1119:string)
        n559 = case shown="True" w1123 {
          tunnel: w1124 -> [_ w1147]
          tunnel: w1119 -> [_ w1146]
          frame False {
          }
          frame True {
            n560 = call "Send Email2"("Message"=w1146, "Subject"=w1146, "Recipients"=w1147) -> ()  [unwired: 8 in, 1 out]
          }
        }
        n561 = case shown="False" w1115 {
          tunnel: ["Idle" "AskPostNotes"] -> w1127
          tunnel: [FALSE TRUE] -> w1114
          frame False {
          }
          frame True {
          }
        }
      }
      frame "Abort" {
        n562 = flat-sequence {
          tunnel: [w1193] -> w1191
          tunnel: [w1192] -> w1190
          frame #0 {
            w1192 = TRUE
            n563 = call <extravilib>:"Write.vi"("element"=w1192) -> ("channel"=w1193:T27)  [unwired: 1 out]
          }
        }
      }
    }
    n564 = call "RunNext.vi"("Override"=w126, "Default"=w128, "Cluster"=w127) -> ("output cluster"=w129:T11, "NextAction"=w130:string)  [unwired: 7 in]
  }
  n565 = while {
    tunnel: w13 -> [w1196]
    shift-right: [w1203] -> _
    shift-left: errorcluster {"status"=FALSE, "code"=0, "source"=""} ("error IO") -> [w1202]
    tunnel: [w1201] -> w35
    tunnel: w17 -> [w1200]
    tunnel: w16 -> [w1198]
    stop <- w1197 stop-if-true
    n566 = call <extravilib>:"Read.vi"("channel"=w1196) -> ("element"=w1195:errorcluster)  [unwired: 8 in, 2 out]
    n567 = call <extravilib>:"Read.vi"("channel"=w1200) -> ("element"=w1199:bool)  [unwired: 1 in, 1 out]
    n568 = case shown="False" w1199 {
      tunnel: [w1206 errorcluster {"status"=FALSE, "code"=0, "source"=""} ("error constant")] -> w1203
      tunnel: w1202 -> [w1205 _]
      tunnel: w1195 -> [w1204 _]
      frame False {
        n569 = Merge Errors(w1205, w1204) -> (w1206:errorcluster)
      }
      frame True {
      }
    }
    n570 = call <extravilib>:"Write.vi"("element"=w1203) -> ("channel"=w1201:T47)  [unwired: 1 out]
    n571 = call <extravilib>:"Read.vi"("channel"=w1198) -> ("element"=w1197:bool)  [unwired: 1 in, 1 out]
    n572 = Wait (ms)(milliseconds to wait=u32 100) -> ()  [unwired: 1 out]
  }
  n573 = while {
    shift-right: [w1224] -> _
    shift-left: "Idle" ("AfterErrorCheck") -> [w1223]
    shift-right: [w1221] -> _
    shift-left: errorcluster {"status"=FALSE, "code"=0, "source"=""} ("error out") -> [w1222]
    shift-right: [w1219] -> _
    shift-left: T10 {"Physical Settings"={"physical channels"="Dev1/ai0:2", "source"="OnboardClock", "Start Trigger"="/Dev1/ai/StartTrigger", "StartTriggered"=FALSE}, "Acquisition Settings"={"SyncType"=enum."NoSync", "Frame Rate"=30.0, "Sample Rate"=50000.0, "Sample BufferSize"=100000}, "Channel Names"="", "task in"="", "FileSettings"={"Path"=path "E:/Jacob", "File"="Test3", "FileFormat"=enum."TDMS", "FileSuffix"="_Data_Output", "Multiple Time Columns"=TRUE}} -> [w1220]
    shift-right: [w1217] -> _
    shift-left: w11 -> [w1218]
    tunnel: w13 -> [w1216]
    tunnel: w35 -> [w1215]
    tunnel: w3 -> [w1214]
    tunnel: [w1213] -> w4
    tunnel: w22 -> [w1212]
    tunnel: w21 -> [w1211]
    tunnel: [w1210] -> w18
    tunnel: w16 -> [w1209]
    stop <- w1208 stop-if-true
    # "Analog Input"
    n574 = call <extravilib>:"Write.vi"("element"=w1223) -> ("channel"=w1210:T49)  [unwired: 1 out]
    n575 = case shown="\"Acquire\"" w1223 {
      tunnel: ["Acquire" ("AfterErrorCheck") w1285 "FinalErrorCheck" w1352 "Idle" ("AfterErrorCheck") "InitializeChannels" "InitializeFile" w1423 "WaitForAcStart" ("AfterErrorCheck") "WaitForAcStart" ("AfterErrorCheck")] -> w1224
      tunnel: w1222 -> [w1234 w1283 w1327 w1355 w1370 _ w1409 w1422 w1431 w1448]
      tunnel: [w1232 w1279 w1328 w1349 w1369 errorcluster {"status"=FALSE, "code"=0, "source"=""} ("error out") w1408 w1422 w1430 w1448] -> w1221
      tunnel: w1220 -> [w1227 w1287 w1331 w1350 w1371 w1379 w1396 w1424 w1429 w1447]
      tunnel: [w1228 w1286 w1331 w1350 w1371 w1378 w1397 w1424 w1429 w1447] -> w1219
      tunnel: w1218 -> [w1229 w1274 w1330 w1348 w1372 w1388 w1393 w1425 w1433 w1450]
      tunnel: [w1230 w1269 w1323 w1351 w1372 w1387 w1393 w1425 w1432 w1449] -> w1217
      tunnel: [_ w1284 _ w1354 _ _ _ _ _ _] -> w1216
      tunnel: w1215 -> [_ w1282 _ w1353 _ _ _ _ _ _]
      tunnel: w1214 -> [_ w1278 _ _ _ _ _ _ _ _]
      tunnel: [_ w1276 _ _ _ _ _ _ _ _] -> w1213
      tunnel: w1212 -> [_ _ _ _ _ w1391 _ _ _ _]
      tunnel: w1211 -> [_ _ _ _ _ w1390 _ _ _ _]
      frame "WaitForAcStart" {
        n576 = Unbundle By Name(w1227) -> ("task in"=w1233:refnum<k21>)
        n577 = Unbundle By Name(w1229) -> ("SyncStart"=w1236:bool, "Leader"=w1235:bool, "rendezvous ref"=w1237:T7)
        n578 = case shown="True" w1236 {
          tunnel: w1233 -> [w1241 w1245]
          tunnel: w1234 -> [w1240 w1246]
          tunnel: [w1239 w1243] -> w1226
          tunnel: [w1238 w1244] -> w1232
          tunnel: w1235 -> [_ w1247]
          tunnel: w1237 -> [_ w1242]
          frame False {
            n579 = call <vilib>:"DAQmx Start Task.vi"("task/channels in"=w1241, "error in"=w1240) -> ("task out"=w1239:refnum<k21>, "error out"=w1238:errorcluster)  [unwired: 12 in]
          }
          frame True {
            n580 = case shown="True" w1247 {
              tunnel: w1246 -> [w1252 w1260]
              tunnel: w1245 -> [w1251 w1261]
              tunnel: [w1250 w1258] -> w1244
              tunnel: [w1249 w1259] -> w1243
              tunnel: w1242 -> [w1248 w1262]
              frame False {
                n581 = flat-sequence {
                  tunnel: w1252 -> [w1256]
                  tunnel: w1251 -> [w1255]
                  tunnel: [w1254] -> w1250
                  tunnel: [w1253] -> w1249
                  tunnel: w1248 -> [w1257]
                  frame #0 {
                    n582 = call <vilib>:"DAQmx Start Task.vi"("task/channels in"=w1255, "error in"=w1256) -> ("task out"=w1253:refnum<k21>, "error out"=w1254:errorcluster)  [unwired: 12 in]
                  }
                  frame #1 {
                    n583 = call <vilib>:"Wait at Rendezvous.vi"("rendezvous"=w1257) -> ()  [unwired: 4 in, 3 out]
                  }
                  frame #2 {
                  }
                }
              }
              frame True {
                n584 = flat-sequence {
                  tunnel: w1262 -> [w1263]
                  tunnel: w1261 -> [w1267]
                  tunnel: w1260 -> [w1266]
                  tunnel: [w1265] -> w1259
                  tunnel: [w1264] -> w1258
                  frame #0 {
                    n585 = call <vilib>:"Wait at Rendezvous.vi"("rendezvous"=w1263) -> ()  [unwired: 4 in, 3 out]
                  }
                  frame #1 {
                    n586 = call <vilib>:"DAQmx Start Task.vi"("task/channels in"=w1267, "error in"=w1266) -> ("task out"=w1265:refnum<k21>, "error out"=w1264:errorcluster)  [unwired: 12 in]
                  }
                }
              }
            }
          }
        }
        n587 = Bundle By Name(cluster=w1229, "Started?"=TRUE) -> (w1230:T9)
        n588 = Bundle By Name(cluster=w1227, "task in"=w1226) -> (w1228:T10)
      }
      frame "Acquire" {
        n589 = call <extravilib>:"Write.vi"("element"=w1283) -> ("channel"=w1284:T46)  [unwired: 8 in, 2 out]
        n590 = Unbundle By Name(w1287) -> ("task in"=w1290:refnum<k21>, "Acquisition Settings.Sample BufferSize"=w1289:i32, "FileSettings.FileFormat"=w1268:enum16{"TDMS", "CSV"})
        n591 = Unbundle By Name(w1274) -> ("FirstAq"=w1275:bool)
        n592 = call-poly <vilib>:"DAQmx Read.vi"("task/channels in"=w1290, "number of samples per channel"=w1289, "error in"=w1283) -> ("task out"=w1288:refnum<k21>, "data"=w1273:waveform(dbl)[], "error out"=w1280:errorcluster)  [unwired: 10 in]
        n593 = case shown="False" w1275 {
          tunnel: w1274 -> [w1312 w1318]
          tunnel: [w1312 w1317] -> w1270
          tunnel: w1273 -> [_ w1315]
          frame False {
          }
          frame True {
            n594 = for {
              tunnel: w1315 -> [w1320] mode=indexing
              tunnel: [w1319] -> w1314 mode=indexing
              n595 = Unbundle By Name(w1320) -> ("t0"=w1319:timestamp)
            }
            n596 = Array Max & Min(array=w1314) -> (min value=w1313:timestamp)  [unwired: 3 out]
            n597 = Bundle By Name(cluster=w1318, "FirstAq"=FALSE, "t0"=w1313) -> (w1317:T9)
          }
        }
        n598 = Unbundle By Name(w1270) -> ("t0"=w1272:timestamp)
        n599 = for {
          tunnel: w1273 -> [w1309] mode=indexing
          tunnel: w1272 -> [w1310]
          tunnel: [w1305] -> w1271 mode=indexing
          n600 = Unbundle By Name(w1309) -> ("t0"=w1311:timestamp)
          n601 = Subtract(x=w1311, y=w1310) -> (x-y=w1308:dbl)
          n602 = Add(x=w1308, y=timestamp(0 s since 1904-01-01)) -> (x+y=w1306:timestamp)
          n603 = Bundle By Name(cluster=w1309, "t0"=w1306) -> (w1305:waveform(dbl))
        }
        n604 = case shown="\"TDMS\", Default" w1268 {
          tunnel: w1271 -> [w1295 w1303]
          tunnel: w1270 -> [w1294 w1298]
          tunnel: [w1292 w1298] -> w1269
          tunnel: w1270 -> [w1291 w1297]
          frame "TDMS", Default {
            n605 = Unbundle By Name(w1291) -> ("TDMSRef"=w1296:refnum<k34>)
            n606 = TDMS Write(0:w1296, 9:w1295) -> (4:w1293:refnum<k34>)  [unwired: 4 in, 3 out]
            n607 = Bundle By Name(cluster=w1294, "TDMSRef"=w1293) -> (w1292:T9)
          }
          frame "CSV" {
            n608 = Unbundle By Name(w1297) -> ("CSV path"=w1304:path)
            n609 = call-poly <vilib>:"Export Waveforms to Spreadsheet File.vi"("header? (write header:T)"=TRUE, "delimiter (Tab)"=",", "append to file? (new file:F)"=TRUE, "multiple time columns? (single:F)"=TRUE, "waveforms"=w1303, "file path (dialog if empty)"=w1304) -> ()  [unwired: 4 in, 2 out]
          }
        }
        n610 = Bundle By Name(cluster=w1287, "task in"=w1288) -> (w1286:T10)
        n611 = call <extravilib>:"Read.vi"("channel"=w1282) -> ("element"=w1281:errorcluster)  [unwired: 1 in, 1 out]
        n612 = call <extravilib>:"Read.vi"("channel"=w1278) -> ("element"=w1277:bool)  [unwired: 1 in, 1 out]
        n613 = call <extravilib>:"Write.vi"("element"=w1271) -> ("channel"=w1276:T50)  [unwired: 8 in, 2 out]
        n614 = Merge Errors(w1280, w1281) -> (w1279:errorcluster)
        n615 = case shown="False" w1277 {
          tunnel: ["Shutdown" "Acquire"] -> w1285
          frame True {
          }
          frame False {
          }
        }
      }
      frame "Shutdown" {
        n616 = Unbundle By Name(w1331) -> ("task in"=w1334:refnum<k21>, "FileSettings.FileFormat"=w1324:enum16{"TDMS", "CSV"})
        n617 = Unbundle By Name(w1330) -> ("Started?"=w1335:bool)
        n618 = case shown="True" w1335 {
          tunnel: w1334 -> [w1340 w1347]
          tunnel: [w1340 w1346] -> w1333
          tunnel: w1327 -> [w1339 w1345]
          tunnel: [w1339 w1344] -> w1332
          tunnel: w1330 -> [w1338 w1343]
          tunnel: [w1338 w1342] -> w1326
          frame False {
          }
          frame True {
            n619 = call <vilib>:"DAQmx Stop Task.vi"("task/channels in"=w1347, "error in"=w1345) -> ("task out"=w1346:refnum<k21>, "error out"=w1344:errorcluster)  [unwired: 12 in]
            n620 = Bundle By Name(cluster=w1343, "Started?"=FALSE) -> (w1342:T9)
          }
        }
        n621 = Bundle By Name(cluster=w1326, "FirstAq"=TRUE) -> (w1323:T9)
        n622 = call <vilib>:"DAQmx Clear Task.vi"("task in"=w1333, "error in"=w1332) -> ("error out"=w1328:errorcluster)  [unwired: 13 in]
        n623 = case shown="\"TDMS\", Default" w1324 {
          tunnel: w1323 -> [w1337 _]
          frame "TDMS", Default {
            n624 = Unbundle By Name(w1337) -> ("TDMSRef"=w1336:refnum<k34>)
            n625 = TDMS Close(11:w1336) -> ()  [unwired: 1 in, 2 out]
          }
          frame "CSV" {
          }
        }
      }
      frame "ErrorCheck" {
        n626 = call <extravilib>:"Write.vi"("element"=w1355) -> ("channel"=w1354:T46)  [unwired: 8 in, 2 out]
        n627 = call <extravilib>:"Read.vi"("channel"=w1353) -> ("element"=w1356:errorcluster)  [unwired: 1 in, 1 out]
        n628 = Merge Errors(w1356, w1355) -> (w1349:errorcluster)
        n629 = Unbundle By Name(w1348) -> ("AfterErrorCheck"=w1358:string)
        n630 = flat-sequence {
          tunnel: w1358 -> [w1363]
          tunnel: "Shutdown" ("t") -> [w1362]
          tunnel: w1349 -> [w1360]
          tunnel: [w1361] -> w1359
          tunnel: [w1367] -> w1352
          tunnel: w1359 -> [w1367]
          tunnel: w1348 -> [w1366]
          tunnel: [w1364] -> w1351
          frame #0 {
            n631 = Select(t=w1362, s=w1360, f=w1363) -> (s? t:f=w1361:string)
          }
          frame #1 {
            n632 = Bundle By Name(cluster=w1366, "AfterErrorCheck"="Shutdown") -> (w1364:T9)
          }
        }
      }
      frame "FinalErrorCheck" {
        n633 = call <vilib>:"Simple Error Handler.vi"("error in (no error)"=w1370) -> ("error out"=w1369:errorcluster)  [unwired: 4 in, 4 out]
      }
      frame "Idle", Default {
        n634 = call <extravilib>:"Read.vi"("channel"=w1391) -> ("element"=w1377:T10)  [unwired: 8 in, 2 out]
        n635 = call <extravilib>:"Read.vi"("channel"=w1390) -> ("element"=w1386:T42)  [unwired: 8 in, 2 out]
        n636 = Unbundle By Name(w1386) -> ("SyncStart"=w1385:bool, "Leader"=w1384:bool, "Started?"=w1383:bool, "AfterErrorCheck"=w1382:string, "rendezvous ref"=w1381:T7, "AcStarted"=w1380:bool)
        n637 = Unbundle By Name(w1377) -> ("Physical Settings"=w1376:T38, "Acquisition Settings"=w1375:T43, "Channel Names"=w1374:string, "FileSettings"=w1373:T36)
        n638 = Bundle By Name(cluster=w1388, "SyncStart"=w1385, "Leader"=w1384, "Started?"=w1383, "AfterErrorCheck"=w1382, "rendezvous ref"=w1381, "AcStarted"=w1380) -> (w1387:T9)
        n639 = Bundle By Name(cluster=w1379, "Physical Settings"=w1376, "Acquisition Settings"=w1375, "Channel Names"=w1374, "FileSettings"=w1373) -> (w1378:T10)
      }
      frame "InitializeChannels" {
        w1407 = 10123 items=["Finite Samples"=10178, "Continuous Samples"=10123, "Hardware Timed Single Point"=12522] ("sample mode")
        n640 = Unbundle By Name(w1396) -> ("Acquisition Settings"=w1406:T43)
        n641 = Unbundle By Name(w1396) -> ("Physical Settings.physical channels"=w1403:tag, "Channel Names"=w1402:string)
        n642 = Unbundle By Name(w1406) -> ("SyncType"=w1405:enum16{"NoSync", "Sync"}, "Frame Rate"=w1404:dbl, "Sample Rate"=w1394:dbl)
        n643 = call "IfSyncedCompatible.vi"("error in (no error)"=w1409, "Sample Rate"=w1394, "Frame Rate"=w1404, "Enum"=w1405) -> ("error out"=w1410:errorcluster)  [unwired: 7 in]
        n644 = Unbundle By Name(w1396) -> ("Physical Settings"=w1401:T38)
        n645 = call-poly <vilib>:"DAQmx Create Virtual Channel.vi"("physical channels"=w1403, "name to assign"=w1402, "error in"=w1410) -> ("task out"=w1414:refnum<k21>, "error out"=w1413:errorcluster)  [unwired: 11 in]
        n646 = Unbundle By Name(w1401) -> ("Start Trigger"=w1399:tag, "StartTriggered"=w1400:bool)
        n647 = call-poly <vilib>:"DAQmx Timing.vi"("task/channels in"=w1414, "sample mode"=w1407, "rate"=w1394, "error in"=w1413) -> ("task out"=w1411:refnum<k21>, "error out"=w1412:errorcluster)  [unwired: 10 in]
        n648 = case shown="False" w1400 {
          tunnel: w1412 -> [w1416 w1421]
          tunnel: w1411 -> [w1415 w1420]
          tunnel: [w1415 w1419] -> w1395
          tunnel: [w1416 w1418] -> w1408
          tunnel: w1399 -> [_ w1417]
          frame False {
          }
          frame True {
            n649 = call-poly <vilib>:"DAQmx Trigger.vi"("task/channels in"=w1420, "source"=w1417, "error in"=w1421) -> ("task out"=w1419:refnum<k21>, "error out"=w1418:errorcluster)  [unwired: 11 in]
          }
        }
        n650 = Bundle By Name(cluster=w1396, "task in"=w1395) -> (w1397:T10)
      }
      frame "InitializeFile" {
        n651 = Unbundle By Name(w1424) -> ("FileSettings.FileFormat"=w1426:enum16{"TDMS", "CSV"})
        n652 = case shown="\"TDMS\", Default" w1426 {
          tunnel: ["InitializeTDMS" ("AfterErrorCheck") "InitializeCSV" ("AfterErrorCheck")] -> w1423
          frame "TDMS", Default {
          }
          frame "CSV" {
          }
        }
      }
      frame "InitializeTDMS" {
        n653 = Unbundle By Name(w1429) -> ("FileSettings.Path"=w1434:path, "FileSettings.File"=w1435:string, "FileSettings.FileSuffix"=w1439:string)
        n654 = Concatenate Strings(w1435, w1439, ".tdms" ("string")) -> (w1438:string)
        n655 = Build Path(base path=w1434, name or relative path=w1438) -> (appended path=w1437:path)
        n656 = TDMS Open(8:w1431, 10:T48."open or create" ("operation (0:open)"), 11:w1437) -> (0:w1444:errorcluster, 3:w1441:refnum<k34>)  [unwired: 4 in]
        n657 = TDMS Set Properties(5:string[] ["Data"] ("property values"), 7:string[] ["Title"] ("property names"), 8:w1444, 11:w1441) -> (0:w1430:errorcluster, 3:w1440:refnum<k34>)  [unwired: 2 in, 2 out]
        n658 = Bundle By Name(cluster=w1433, "TDMSRef"=w1440) -> (w1432:T9)
      }
      frame "InitializeCSV" {
        n659 = Unbundle By Name(w1447) -> ("FileSettings.Path"=w1452:path, "FileSettings.File"=w1456:string, "FileSettings.FileSuffix"=w1455:string)
        n660 = Concatenate Strings(w1456, w1455, ".csv" ("string")) -> (w1454:string)
        n661 = Build Path(base path=w1452, name or relative path=w1454) -> (appended path=w1451:path)
        n662 = Bundle By Name(cluster=w1450, "CSV path"=w1451) -> (w1449:T9)
      }
    }
    n663 = call <extravilib>:"Read.vi"("channel"=w1209) -> ("element"=w1208:bool)  [unwired: 1 in, 1 out]
  }
  n664 = while {
    shift-right: [w1474] -> _
    shift-left: "Idle" ("AfterErrorCheck") -> [w1458]
    shift-right: [w1472] -> _
    shift-left: T21 {"User Camera Settings"={"Pixel Format"="Mono 8", "Width"=1280, "Height"=1024, "Trigger Source"="Line 3", "Readout Mode"="Normal", "Session In"="cam0"}, "IMAQdx Session"="", "Camera Aq Attributes"={"Readout Time"=0.0, "Resulting FPS"=0.0, "Width"=0, "Height"=0, "Format"=0, "Bit Depth"=0}, "Camera Attributes"={"Exposure Start Delay"=0.0, "Model"="", "Make"=""}, "AcquisitionSettings"={"Buffer"=10, "FramesPerFile"=100000}, "Image Buffer"=[], "Example Image"=refnum, "AVIRef"=refnum, "TDMSRef"=refnum, "TDMSWSet"={"Image Type"=0, "Async File Format"=FALSE}, "CameraSignalRefnum"="", "CameraSignalDefinition"={"High Time"=0.0, "Low Time"=0.0, "Delay"=0.0}, "DisplayEveryNFrames"=30, "Trigger Settings"={"FPS"=30, "Exposure Time"=0.0001, "Start Trigger Source"="/Dev1/ai/StartTrigger", "Camera\nClock\nCounter"="Dev1/ctr0", "PhysicalCameraSignalLine"="/Dev1/PFI2", "Sync Type"=""}, "FileSettings"={"FileSaveLocation"=path "", "FileName"="", "VideoSuffix"="", "Codec"="", "Quality"=0, "Format"="", "AVI FPS"=0, "TimingSuffix"=""}} -> [w1473]
    shift-right: [w1471] -> _
    shift-left: errorcluster {"status"=FALSE, "code"=0, "source"=""} ("error out") -> [w1470]
    shift-right: [w1468] -> _
    shift-left: w10 -> [w1469]
    tunnel: w13 -> [w1467]
    tunnel: w35 -> [w1466]
    tunnel: [w1465] -> w105
    tunnel: w3 -> [w1464]
    tunnel: w26 -> [w1463]
    tunnel: w25 -> [w1462]
    tunnel: [w1461] -> w20
    tunnel: w16 -> [w1460]
    stop <- w1459 stop-if-true
    # "State"
    # "Variables"
    # "Running\nOptions"
    # "Camera"
    n665 = call <extravilib>:"Write.vi"("element"=w1458) -> ("channel"=w1461:T49)  [unwired: 1 out]
    n666 = case shown="\"Acquire\"" w1458 {
      tunnel: ["Idle" ("AfterErrorCheck") "InitializeCameraSettings" "ReadCameraAttributes" "ExposureStartDelay" ("AfterErrorCheck") "CheckParameterCompatability" "ErrorCheck" "ErrorCheck" ("AfterErrorCheck") w1710 "ErrorCheck" ("AfterErrorCheck") "ErrorCheck" ("AfterErrorCheck") w1808 "ErrorCheck" ("AfterErrorCheck") "WaitForAcStart" w1855 w1933 w2051 "Shutdown" ("AfterErrorCheck") "Shutdown" ("AfterErrorCheck") "Shutdown" ("AfterErrorCheck") "Shutdown" ("AfterErrorCheck") "Shutdown" ("AfterErrorCheck") "Shutdown" ("AfterErrorCheck") "Shutdown" ("AfterErrorCheck") "Shutdown" ("AfterErrorCheck") "Idle" ("AfterErrorCheck")] -> w1474
      tunnel: w1473 -> [w1479 w1501 w1512 w1556 w1570 w1647 w1681 w1704 w1744 w1770 w1811 w1820 w1837 w1856 w1873 w2054 w2092 w2106 w2120 w2126 w2142 w2154 w2163 w2180 w2265]
      tunnel: [w1479 w1502 w1515 w1557 w1569 w1647 w1676 w1704 w1745 w1767 w1811 w1821 w1838 w1860 w1939 w2054 w2092 w2105 w2119 w2126 w2142 w2154 w2163 w2180 w2265] -> w1472
      tunnel: [w1477 errorcluster {"status"=FALSE, "code"=0, "source"=""} ("error in (no error)") w1516 w1546 w1566 w1650 w1677 w1708 w1742 w1766 w1806 w1824 w1839 w1854 w1881 w2053 w2093 w2103 w2117 w2129 w2141 w2149 w2160 w2183 w2262] -> w1471
      tunnel: w1470 -> [w1478 _ _ w1558 w1564 w1660 w1665 w1709 w1737 w1787 w1805 w1825 w1842 w1862 w1879 w2053 w2094 w2104 w2116 w2130 w2148 w2150 w2161 w2184 w2266]
      tunnel: w1469 -> [w1480 w1504 w1509 w1543 w1562 w1648 w1672 w1702 w1736 w1782 w1801 w1826 w1834 w1859 w1913 w2049 w2091 w2101 w2115 w2125 w2146 w2153 w2164 w2185 w2264]
      tunnel: [w1480 w1503 w1510 w1543 w1562 w1649 w1673 w1700 w1740 w1788 w1800 w1827 w1834 w1858 w1905 w2055 w2090 w2099 w2115 w2124 w2144 w2151 w2164 w2185 w2264] -> w1468
      tunnel: [_ _ _ _ _ _ _ _ _ _ w1807 _ _ _ w1922 _ _ _ _ _ _ _ _ _ _] -> w1467
      tunnel: w1466 -> [_ _ _ _ _ _ _ _ _ _ w1804 _ _ _ _ _ _ _ _ _ _ _ _ _ _]
      tunnel: [_ _ _ _ _ _ _ _ _ _ _ _ _ _ w1935 _ _ _ _ _ _ _ _ _ _] -> w1465
      tunnel: w1464 -> [_ _ _ _ _ _ _ _ _ _ _ _ _ _ w1931 _ _ _ _ _ _ _ _ _ _]
      tunnel: w1463 -> [_ w1506 _ _ _ _ _ _ _ _ _ _ _ _ _ _ _ _ _ _ _ _ _ _ _]
      tunnel: w1462 -> [_ w1505 _ _ _ _ _ _ _ _ _ _ _ _ _ _ _ _ _ _ _ _ _ _ _]
      tunnel: w1458 -> [_ _ _ _ _ _ _ _ _ _ _ _ _ _ _ _ _ _ _ _ _ _ _ _ _]
      frame "BadReference", Default {
        n667 = xnode "Error Ring"() -> ("error out"=w1476:errorcluster)
        n668 = Merge Errors(w1478, w1476) -> (w1477:errorcluster)
      }
      frame "Idle" {
        n669 = call <extravilib>:"Read.vi"("channel"=w1505) -> ("element"=w1500:T31)  [unwired: 8 in, 2 out]
        n670 = call <extravilib>:"Read.vi"("channel"=w1506) -> ("element"=w1495:T24)  [unwired: 8 in, 2 out]
        n671 = Unbundle By Name(w1500) -> ("SyncStart"=w1488:bool, "ConfirmTDMSOptimizations"=w1496:bool, "ConfirmTDMSDisableBuffer"=w1497:bool, "VideoSave"=w1498:bool, "rendezvous ref"=w1499:T7)
        n672 = Unbundle By Name(w1495) -> ("User Camera Settings"=w1489:T33, "Trigger Settings"=w1490:T30, "Camera Attributes"=w1491:T53, "AcquisitionSettings"=w1492:cluster{"Buffer":i32, "FramesPerFile":i32}, "FileSettings"=w1493:T32, "DisplayEveryNFrames"=w1494:i32)
        n673 = Not(x=w1488) -> (.not. x?=w1487:bool)
        n674 = Bundle By Name(cluster=w1501, "User Camera Settings"=w1489, "Trigger Settings"=w1490, "Camera Attributes"=w1491, "AcquisitionSettings"=w1492, "FileSettings"=w1493, "DisplayEveryNFrames"=w1494) -> (w1502:T21)
        n675 = Bundle By Name(cluster=w1504, "SyncStart"=w1488, "ConfirmTDMSOptimizations"=w1496, "ConfirmTDMSDisableBuffer"=w1497, "VideoSave"=w1498, "rendezvous ref"=w1499, "AcStarted"=w1487) -> (w1503:T17)
      }
      frame "InitializeCameraSettings" {
        w1513 = u32 0 items=["Get Oldest"=0, "Fail"=2, "Get Newest"=3] ("OverwriteMode")
        # "User Settings"
        # "Mandatory Settings"
        n676 = Unbundle By Name(w1512) -> ("User Camera Settings.Session In"=w1511:T2)
        n677 = call <vilib>:"IMAQdx Open Camera.vi"("Session In"=w1511) -> ("error out"=w1536:errorcluster, "Session Out"=w1535:T2)  [unwired: 9 in]
        n678 = property class="IMAQdx"(reference=w1535, error in=w1536, "ActiveAttribute"="CameraAttributes::AcquisitionControl::TriggerMode", "ValueString"="On", "ActiveAttribute"="CameraAttributes::AcquisitionControl::ExposureMode", "ValueString"="Trigger Width", "OverwriteMode"=w1513) -> (reference out=w1530:T2, error out=w1529:errorcluster)
        n679 = Unbundle By Name(w1512) -> ("User Camera Settings"=w1528:T33)
        n680 = Bundle By Name(cluster=w1509, "CameraOpen"=TRUE) -> (w1510:T17)
        n681 = Unbundle By Name(w1528) -> ("Pixel Format"=w1522:string, "Width"=w1521:i64, "Height"=w1520:i64, "Trigger Source"=w1519:string, "Readout Mode"=w1518:string)
        n682 = property class="IMAQdx"(reference=w1530, error in=w1529, "ActiveAttribute"="CameraAttributes::ImageFormatControl::PixelFormat", "ValueString"=w1522, "ActiveAttribute"="CameraAttributes::ImageFormatControl::Width", "ValueU32"=w1521, "ActiveAttribute"="CameraAttributes::ImageFormatControl::Height", "ValueU32"=w1520, "ActiveAttribute"="CameraAttributes::AcquisitionControl::TriggerSource", "ValueString"=w1519, "ActiveAttribute"="CameraAttributes::AcquisitionControl::SensorReadoutMode", "ValueString"=w1518) -> (reference out=w1514:T2, error out=w1516:errorcluster)
        n683 = Bundle By Name(cluster=w1512, "IMAQdx Session"=w1514) -> (w1515:T21)
      }
      frame "ReadCameraAttributes" {
        n684 = Unbundle By Name(w1556) -> ("IMAQdx Session"=w1559:T2)
        n685 = Unbundle By Name(w1556) -> ("Camera Aq Attributes"=w1555:T54, "Camera Attributes"=w1541:T53)
        n686 = property class="IMAQdx"(reference=w1559, error in=w1558, "ActiveAttribute"="CameraAttributes::AcquisitionControl::SensorReadoutTime", "ActiveAttribute"="CameraAttributes::AcquisitionControl::ResultingFrameRate", "ActiveAttribute"="TypeOfImageInUse", "ActiveAttribute"="BitsPerPixelInUse", "ActiveAttribute"="CameraAttributes::DeviceControl::DeviceModelName") -> (reference out=w1544:T2, error out=w1546:errorcluster, "ValueDBL"=w1554:dbl, "ValueDBL"=w1553:dbl, "ValueU32"=w1550:u32, "ValueU32"=w1549:u32, "Width"=w1548:u32, "Height"=w1547:u32, "VendorName"=w1540:string, "ValueString"=w1539:string)
        n687 = Bundle By Name(cluster=w1555, "Readout Time"=w1554, "Resulting FPS"=w1553, "Format"=w1550, "Bit Depth"=w1549, "Width"=w1548, "Height"=w1547) -> (w1545:T54)
        n688 = Bundle By Name(cluster=w1541, "Make"=w1540, "Model"=w1539) -> (w1538:T53)
        n689 = Bundle By Name(cluster=w1556, "IMAQdx Session"=w1544, "Camera Aq Attributes"=w1545, "Camera Attributes"=w1538) -> (w1557:T21)
      }
      frame "ExposureStartDelay" {
        n690 = Unbundle By Name(w1570) -> ("IMAQdx Session"=w1567:T2, "Camera Aq Attributes.Bit Depth"=w1568:u32, "Camera Attributes"=w1573:T53, "Trigger Settings.Exposure Time"=w1563:dbl)
        n691 = Unbundle By Name(w1573) -> ("Make"=w1572:string, "Model"=w1571:string)
        n692 = case shown="\"Basler\"" w1572 {
          tunnel: w1571 -> [_ w1583]
          tunnel: w1570 -> [w1575 w1582]
          tunnel: [w1575 w1581] -> w1569
          tunnel: w1568 -> [_ w1580]
          tunnel: w1567 -> [_ w1579]
          tunnel: [errorcluster {"status"=TRUE, "code"=2458, "source"="This make of camera is not yet supported"} ("error constant") w1578] -> w1565
          tunnel: w1563 -> [_ w1577]
          frame "False", Default {
          }
          frame "Basler" {
            n693 = case shown="\"acA1300-200um\"" w1583 {
              tunnel: w1582 -> [w1591 w1632 w1643]
              tunnel: [w1592 w1632 w1641] -> w1581
              tunnel: w1580 -> [w1590 _ _]
              tunnel: w1579 -> [w1587 _ _]
              tunnel: [w1585 errorcluster {"status"=TRUE, "code"=4557, "source"="Basler Camera Model Not Yet Supported"} ("error constant") w1637] -> w1578
              tunnel: w1577 -> [w1584 _ w1638]
              frame "acA720-520uc" {
                n694 = property class="IMAQdx"(reference=w1587, "ActiveAttribute"="CameraAttributes::AcquisitionControl::ExposureTimeMode") -> ("ValueString"=w1586:string)  [unwired: 1 in, 2 out]
                n695 = case shown="Default" w1586 {
                  tunnel: w1590 -> [w1600 _ w1611]
                  tunnel: [w1601 0.0 w1610] -> w1589
                  tunnel: [w1593 errorcluster {"status"=TRUE, "code"=2134, "source"="Exposure mode not supported"} ("error constant") w1608] -> w1585
                  tunnel: w1584 -> [w1598 _ w1609]
                  frame "Ultra Short" {
                    n696 = case shown="12" w1600 {
                      tunnel: [2.7e-05 3.5e-05] -> w1601
                      frame 8, Default {
                      }
                      frame 12 {
                      }
                    }
                    n697 = Greater?(x=w1598, y=1e-06) -> (0:w1594:bool)
                    n698 = Less?(x=w1598, y=1.3e-05) -> (x < y?=w1595:bool)
                    n699 = Or(x=w1594, y=w1595) -> (x .or. y?=w1596:bool)
                    n700 = case shown="False" w1596 {
                      tunnel: [errorcluster {"status"=TRUE, "code"=47896, "source"="Ultra short exposure requires\ntimes between 13-1 us"} ("error constant") errorcluster {"status"=FALSE, "code"=0, "source"=""} ("error constant")] -> w1593
                      frame False {
                      }
                      frame True {
                      }
                    }
                  }
                  frame Default {
                  }
                  frame "Standard" {
                    n701 = case shown="8, Default" w1611 {
                      tunnel: [1.15e-05 1.8e-05] -> w1610
                      tunnel: w1609 -> [w1612 w1626]
                      tunnel: [w1613 w1622] -> w1608
                      frame 8, Default {
                        n702 = Greater?(x=w1612, y=0.0003) -> (0:w1616:bool)
                        n703 = Less?(x=w1612, y=1.0) -> (x < y?=w1615:bool)
                        n704 = And(x=w1616, y=w1615) -> (x .and. y?=w1614:bool)
                        n705 = case shown="False" w1614 {
                          tunnel: [errorcluster {"status"=TRUE, "code"=0, "source"="12 bit exposure\non this model \nrequires between\n1s-30us exposure"} ("error constant") errorcluster {"status"=FALSE, "code"=0, "source"=""} ("error constant")] -> w1613
                          frame False {
                          }
                          frame True {
                          }
                        }
                      }
                      frame 12 {
                        n706 = Greater?(x=w1626, y=2.4e-05) -> (0:w1625:bool)
                        n707 = Less?(x=w1626, y=1.0) -> (x < y?=w1624:bool)
                        n708 = And(x=w1625, y=w1624) -> (x .and. y?=w1623:bool)
                        n709 = case shown="False" w1623 {
                          tunnel: [errorcluster {"status"=TRUE, "code"=0, "source"="12 bit exposure\non this model \nrequires between\n1s-24us exposure"} ("error constant") errorcluster {"status"=FALSE, "code"=0, "source"=""} ("error constant")] -> w1622
                          frame False {
                          }
                          frame True {
                          }
                        }
                      }
                    }
                  }
                }
                n710 = Bundle By Name(cluster=w1591, "Camera Attributes.Exposure Start Delay"=w1589) -> (w1592:T21)
              }
              frame "NotSupported", Default {
              }
              frame "acA1300-200um" {
                n711 = Greater?(x=w1638, y=5.9e-05 ("x")) -> (0:w1635:bool)
                n712 = Less?(x=w1638, y=1.0) -> (x < y?=w1634:bool)
                n713 = And(x=w1635, y=w1634) -> (x .and. y?=w1636:bool)
                n714 = case shown="True" w1636 {
                  tunnel: [errorcluster {"status"=TRUE, "code"=4879, "source"="Exposure time needs to be\nlarger than 59 us or less than 1s"} ("error constant") errorcluster {"status"=FALSE, "code"=0, "source"=""} ("error constant")] -> w1637
                  frame False {
                  }
                  frame True {
                  }
                }
                n715 = Bundle By Name(cluster=w1643, "Camera Attributes.Exposure Start Delay"=8e-06) -> (w1641:T21)
              }
            }
          }
        }
        n716 = Merge Errors(w1564, w1565) -> (w1566:errorcluster)
      }
      frame "CheckParameterCompatability" {
        n717 = Unbundle By Name(w1647) -> ("Camera Attributes.Exposure Start Delay"=w1659:dbl, "Camera Aq Attributes"=w1656:T54, "Trigger Settings"=w1658:T30)
        n718 = Unbundle By Name(w1658) -> ("FPS"=w1654:i32, "Exposure Time"=w1657:dbl)
        n719 = Unbundle By Name(w1656) -> ("Readout Time"=w1655:dbl, "Resulting FPS"=w1653:dbl, "Width"=w1652:u32)
        n720 = call "CheckExposure.vi"("error constant"=w1660, "Sensor readout time"=w1655, "Frame Rate"=w1654, "Exposure Time"=w1657, "Exposure Start Delay"=w1659) -> ("error out"=w1662:errorcluster)  [unwired: 6 in]
        n721 = call "IsFPSSmaller.vi"("error constant"=w1662, "Frame Rate"=w1654, "Max FrameRate"=w1653) -> ("error out"=w1661:errorcluster)  [unwired: 8 in]
        n722 = call "IsWidthRingCompatible.vi"("error in (no error)"=w1661, "Width"=w1652) -> ("error out"=w1650:errorcluster)  [unwired: 9 in]
        n723 = Bundle By Name(cluster=w1648, "AfterErrorCheck"="ConfigureRingAcquisition") -> (w1649:T17)
      }
      frame "ConfigureRingAcquisition" {
        n724 = Unbundle By Name(w1681) -> ("IMAQdx Session"=w1684:T2, "AcquisitionSettings.Buffer"=w1683:i32, "Image Buffer"=w1666:T18[])
        n725 = for {
          shift-right: [w1687] -> w1664
          shift-left: w1665 -> [w1688]
          tunnel: w1666 -> [w1686] mode=indexing
          n726 = call "IMAQ Dispose"("Image"=w1686, "error in (no error)"=w1688) -> ("error out"=w1687:errorcluster)  [unwired: 4 in]
        }
        n727 = for {
          N: w1683 -> [_]
          tunnel: [w1696] -> w1675 mode=indexing
          shift-right: [w1695] -> w1682
          shift-left: w1664 -> [w1690]
          i -> [w1694]
          n728 = Format Into String(format string="Stream Images %d" ("Image Name"), error in=w1690, w1694) -> (resulting string=w1693:string, error out=w1689:errorcluster)  [unwired: 1 in]
          n729 = call "IMAQ Create"("Border Size"=0, "Image Name"=w1693, "error in (no error)"=w1689) -> ("New Image"=w1696:T18, "error out"=w1695:errorcluster)  [unwired: 1 in, 1 out]
        }
        n730 = call <vilib>:"IMAQdx Configure Ring Acquisition.vi"("Mode"=IMAQdx_Acquisition_Mode."Continuous" ("Continuous?"), "error in"=w1682, "Images"=w1675, "Session In"=w1684) -> ("error out"=w1677:errorcluster, "Images Out"=w1679:T18[], "Session Out"=w1680:T2)  [unwired: 5 in]
        n731 = Index Array(array=w1679) -> (element=w1678:T18)  [unwired: 1 in]
        n732 = Bundle By Name(cluster=w1681, "IMAQdx Session"=w1680, "Example Image"=w1678, "Image Buffer"=w1675) -> (w1676:T21)
        n733 = Unbundle By Name(w1672) -> ("VideoSave"=w1671:bool)
        n734 = Select(t="FileInitialize", s=w1671, f="InitializeIMAQ") -> (s? t:f=w1670:string)
        n735 = Bundle By Name(cluster=w1672, "AfterErrorCheck"=w1670, "Acquisition Configured"=TRUE, "BufferOpen"=TRUE) -> (w1673:T17)
      }
      frame "FileInitialize" {
        n736 = Unbundle By Name(w1704) -> ("FileSettings.Format"=w1697:string)
        n737 = Unbundle By Name(w1704) -> ("FileSettings"=w1707:T32)
        n738 = Unbundle By Name(w1707) -> ("FileSaveLocation"=w1698:path, "FileName"=w1699:string, "VideoSuffix"=w1706:string)
        n739 = Concatenate Strings(w1699, w1706, "_000") -> (w1703:string)
        n740 = case shown="\"TDMS\"" w1697 {
          tunnel: ["ErrorCheck" "InitializeIMAQ" "TDMSInitialize" "AVIInitialize"] -> w1710
          tunnel: w1709 -> [w1713 w1716 w1719 w1726]
          tunnel: [w1712 w1716 w1719 w1726] -> w1708
          tunnel: w1703 -> [_ _ w1724 w1728]
          tunnel: w1698 -> [w1711 w1717 w1722 w1729]
          tunnel: [w1711 w1717 w1720 w1727] -> w1701
          frame "BadOption", Default {
            n741 = Merge Errors(errorcluster {"status"=TRUE, "code"=199, "source"="The file format is not implemented"} ("error constant"), w1713) -> (w1712:errorcluster)
          }
          frame "None" {
          }
          frame "TDMS" {
            n742 = Concatenate Strings(w1724, ".tdms" ("string")) -> (w1721:string)
            n743 = Build Path(base path=w1722, name or relative path=w1721) -> (appended path=w1720:path)
          }
          frame "AVI" {
            n744 = Concatenate Strings(w1728, ".avi" ("string")) -> (w1731:string)
            n745 = Build Path(base path=w1729, name or relative path=w1731) -> (appended path=w1727:path)
          }
        }
        n746 = Bundle By Name(cluster=w1702, "VideoPath"=w1701) -> (w1700:T17)
      }
      frame "AVIInitialize" {
        # "If codec selected doesn't match\nOr if user wants to select at runtime"
        # "Check Available Codecs"
        n747 = Unbundle By Name(w1744) -> ("Camera Aq Attributes"=w1757:T54, "Example Image"=w1752:T18, "FileSettings.Codec"=w1749:string, "Trigger Settings.FPS"=w1733:i32, "FileSettings.Quality"=w1741:i32)
        n748 = Unbundle By Name(w1757) -> ("Width"=w1756:u32, "Height"=w1755:u32, "Format"=w1754:u32, "Bit Depth"=w1753:u32)
        n749 = call "GetAVICodecs.vi"("error in (no error)"=w1737, "Refnum in"=w1752, "Bit Depth"=w1753, "Format"=w1754, "Height"=w1755, "Width"=w1756) -> ("error out"=w1748:errorcluster, "Codec Names"=w1750:string[])  [unwired: 4 in]
        n750 = Search 1D Array(1D array=w1750, element=w1749) -> (index of element=w1751:i32)  [unwired: 1 in]
        n751 = case shown="-1" w1751 {
          tunnel: w1750 -> [_ w1763]
          tunnel: w1749 -> [w1759 _]
          tunnel: [w1759 w1762] -> w1746
          tunnel: w1748 -> [w1758 w1761]
          tunnel: [w1758 w1760] -> w1747
          frame Default {
          }
          frame -1 {
            n752 = call "Codec Selector (SubVi).vi"("error in (no error)"=w1761, "Array"=w1763) -> ("error out"=w1760:errorcluster, "String"=w1762:string)  [unwired: 8 in]
          }
        }
        n753 = Unbundle By Name(w1736) -> ("VideoPath"=w1735:path)
        n754 = call "IMAQ AVI2 Create"("Quality"=w1741, "error in (no error)"=w1747, "Codec"=w1746, "Frames Per Second"=w1733, "AVI Path"=w1735) -> ("error out"=w1742:errorcluster, "AVI Refnum"=w1743:T19)  [unwired: 5 in]
        n755 = Bundle By Name(cluster=w1736, "AfterErrorCheck"="InitializeIMAQ", "FileOpen"=TRUE ("FileCreated")) -> (w1740:T17)
        n756 = Bundle By Name(cluster=w1744, "FileSettings.Codec"=w1746, "AVIRef"=w1743, "FileSettings.AVI FPS"=w1733) -> (w1745:T21)
      }
      frame "TDMSInitialize" {
        n757 = Unbundle By Name(w1782) -> ("VideoPath"=w1785:path)
        n758 = Unbundle By Name(w1770) -> ("Example Image"=w1786:T18, "AcquisitionSettings.FramesPerFile"=w1784:i32)
        n759 = call "InitializeTDMS.vi"("FilePath"=w1785, "error in (no error)"=w1787, "Images per File"=w1784, "Image Ref in"=w1786) -> ("error out"=w1772:errorcluster, "Write Settings Out"=w1768:T55, "Optimizations"=w1783:T56, "Refnum out"=w1769:refnum<k34>)  [unwired: 4 in]
        n760 = Unbundle By Name(w1782) -> ("ConfirmTDMSOptimizations"=w1781:bool, "ConfirmTDMSDisableBuffer"=w1777:bool)
        n761 = Bundle By Name(cluster=w1770, "TDMSRef"=w1769, "TDMSWSet"=w1768) -> (w1767:T21)
        n762 = Unbundle By Name(w1783) -> ("Asynchronous Writes"=w1774:bool, "Reserve Disk Space"=w1773:bool, "Disable Buffering"=w1765:bool)
        n763 = Not(x=w1781) -> (.not. x?=w1779:bool)
        n764 = Not(x=w1777) -> (.not. x?=w1776:bool)
        n765 = And(x=w1774, y=w1773) -> (x .and. y?=w1780:bool)
        n766 = Or(x=w1780, y=w1779) -> (x .or. y?=w1778:bool)
        n767 = Or(x=w1765, y=w1776) -> (x .or. y?=w1775:bool)
        n768 = case shown="False" w1778 {
          tunnel: w1774 -> [w1797 _]
          tunnel: w1773 -> [w1798 _]
          tunnel: w1772 -> [w1796 w1799]
          tunnel: [w1795 w1799] -> w1771
          frame False {
            n769 = call "ShowAsynchAndReserve (SubVI).vi"("error constant 2"=w1796, "Reserve Disk Space in"=w1798, "Asynchronous Writes in"=w1797) -> ("error constant"=w1795:errorcluster)  [unwired: 6 in, 2 out]
          }
          frame True {
          }
        }
        n770 = case shown="True" w1775 {
          tunnel: w1771 -> [w1793 w1794]
          tunnel: [w1791 w1794] -> w1766
          tunnel: w1765 -> [w1792 _]
          frame False {
            n771 = call "Confirm Disable Buffering (SubVI).vi"("error constant 2"=w1793, "Disable Buffering in"=w1792) -> ("error constant"=w1791:errorcluster)  [unwired: 8 in, 1 out]
          }
          frame True {
          }
        }
        n772 = Bundle By Name(cluster=w1782, "AfterErrorCheck"="InitializeIMAQ", "FileOpen"=TRUE ("FileCreated")) -> (w1788:T17)
      }
      frame "ErrorCheck" {
        n773 = call <extravilib>:"Write.vi"("element"=w1805) -> ("channel"=w1807:T46)  [unwired: 8 in, 2 out]
        n774 = call <extravilib>:"Read.vi"("channel"=w1804) -> ("element"=w1803:errorcluster)  [unwired: 1 in, 1 out]
        n775 = Merge Errors(w1803, w1805) -> (w1806:errorcluster)
        n776 = Unbundle By Name(w1801) -> ("AfterErrorCheck"=w1810:string)
        n777 = flat-sequence {
          tunnel: w1810 -> [w1815]
          tunnel: "Shutdown" ("t") -> [w1814]
          tunnel: w1806 -> [w1812]
          tunnel: [w1813] -> w1802
          tunnel: [w1819] -> w1808
          tunnel: w1802 -> [w1819]
          tunnel: w1801 -> [w1818]
          tunnel: [w1816] -> w1800
          frame #0 {
            n778 = Select(t=w1814, s=w1812, f=w1815) -> (s? t:f=w1813:string)
          }
          frame #1 {
            n779 = Bundle By Name(cluster=w1818, "AfterErrorCheck"="Shutdown") -> (w1816:T17)
          }
        }
      }
      frame "InitializeIMAQ" {
        n780 = Unbundle By Name(w1820) -> ("IMAQdx Session"=w1823:T2)
        n781 = call <vilib>:"IMAQdx Start Acquisition.vi"("error in"=w1825, "Session In"=w1823) -> ("error out"=w1824:errorcluster, "Session Out"=w1822:T2)  [unwired: 8 out]
        n782 = Bundle By Name(cluster=w1826, "AfterErrorCheck"="InitializeCameraTrigger", "AcquisitionStarted"=TRUE ("FileCreated")) -> (w1827:T17)
        n783 = Bundle By Name(cluster=w1820, "IMAQdx Session"=w1822) -> (w1821:T21)
      }
      frame "InitializeCameraTrigger" {
        n784 = Unbundle By Name(w1837) -> ("Trigger Settings"=w1847:T30, "Camera Attributes.Exposure Start Delay"=w1843:dbl)
        n785 = Unbundle By Name(w1847) -> ("FPS"=w1846:i32, "Exposure Time"=w1845:dbl, "Start Trigger Source"=w1844:tag, "Camera\nClock\nCounter"=w1841:tag, "PhysicalCameraSignalLine"=w1840:tag, "Sync Type"=w1833:string)
        n786 = Scan From String(input string=w1833, default 1=T25."Exposure Center" ("Sync Type")) -> (output 1=w1831:T25)  [unwired: 3 in, 3 out]
        n787 = call "CameraTriggerSetup.vi"("Camera\nTrigger\nOutput"=w1840, "Frame Rate"=w1846, "Sync Type"=w1831, "Exposure Time"=w1845, "error in"=w1842, "Camera\nClock\nCounter"=w1841, "Start Trigger Source"=w1844, "Exposure Start Delay"=w1843) -> ("error out"=w1839:errorcluster, "CameraSignalDefinition"=w1835:T57, "CameraSignalRefnum"=w1836:refnum<k21>)  [unwired: 1 in]
        n788 = Bundle By Name(cluster=w1837, "CameraSignalRefnum"=w1836, "CameraSignalDefinition"=w1835) -> (w1838:T21)
      }
      frame "WaitForAcStart" {
        # "Counter output can never be the origin of a start trigger,\ninitializing it first always works."
        n789 = Unbundle By Name(w1856) -> ("CameraSignalRefnum"=w1863:refnum<k21>)
        n790 = Unbundle By Name(w1859) -> ("SyncStart"=w1865:bool, "rendezvous ref"=w1851:T7)
        n791 = call <vilib>:"DAQmx Start Task.vi"("task/channels in"=w1863, "error in"=w1862) -> ("task out"=w1861:refnum<k21>, "error out"=w1864:errorcluster)  [unwired: 12 in]
        n792 = case shown="True" w1865 {
          tunnel: w1864 -> [w1867 w1869]
          tunnel: [w1867 w1869] -> w1854
          tunnel: w1851 -> [_ w1870]
          tunnel: [TRUE ("AcStarted") TRUE ("AcStarted")] -> w1849
          frame False {
          }
          frame True {
            n793 = call <vilib>:"Wait at Rendezvous.vi"("rendezvous"=w1870) -> ()  [unwired: 4 in, 3 out]
          }
        }
        n794 = Bundle By Name(cluster=w1856, "CameraSignalRefnum"=w1861) -> (w1860:T21)
        n795 = Bundle By Name(cluster=w1859, "TriggerStarted"=TRUE, "ResetAq?"=TRUE, "AcStarted"=w1849) -> (w1858:T17)
        n796 = Select(t="ErrorCheck", s=w1854, f="Acquire" ("AfterErrorCheck")) -> (s? t:f=w1855:string)
      }
      frame "Acquire" {
        w1894 = u32 1000 ("Minimum Display Update Interval (ms)")
        w1925 = T58 0 items=["no dialog", "OK message", "continue or stop message", "OK message + warnings", "continue/stop + warnings"] ("type of dialog (OK msg:1)")
        w1926 = 1 items=["no exception", "cancel error on match", "set error on match"] ("[exception action] (none:0)")
        w1902 = 0
        w1911 = errorcluster {"status"=FALSE, "code"=0, "source"=""}  # Initial Value
        w1909 = T18 refnum ("Image Out")
        w1916 = u32 0
        w1945 = FALSE  # Release Previous
        # "Only shutdown image acquisition\non timeout or error"
        # "Exclude timout error"
        # "Check if generation error"
        n797 = Unbundle By Name(w1873) -> ("IMAQdx Session"=w1923:T2, "AcquisitionSettings.Buffer"=w1897:i32)
        n798 = Unbundle By Name(w1913) -> ("ResetAq?"=w1893:bool, "Frames"=w1901:i32)
        n799 = feedback #1(w1916) -> (w1915:u32)
        n800 = Select(t=w1916, s=w1893, f=w1915) -> (s? t:f=w1914:u32)
        n801 = call <vilib>:"IMAQdx Extract Image.vi"("Release Previous (true)"=w1945, "Buffer Number Mode (Next)"=IMAQdx_Buffer_Number_Mode."Buffer Number" ("Buffer Number Mode"), "error in"=w1879, "Buffer Number In"=w1914, "Session In"=w1923) -> ("error out"=w1878:errorcluster, "Buffer Number Out"=w1941:u32, "Image Out"=w1942:T18, "Session Out"=w1932:T2)  [unwired: 3 in]
        n802 = call "High Resolution Timer Helper.vi"("error in (no error)"=w1878) -> ("error out"=w1877:errorcluster, "Current Time"=w1876:dbl)  [unwired: 8 in, 1 out]
        n803 = Compound Arithmetic op=ADD(u32 1 ("value"), w1941) -> (w1944:u32)
        n804 = feedback-in #1(w1944) -> ()
        n805 = feedback #2(w1911) -> (w1910:errorcluster)
        n806 = Select(t=w1911, s=w1893, f=w1910) -> (s? t:f=w1889:errorcluster)
        n807 = Unbundle By Name(w1889) -> ("code"=w1887:i32)
        n808 = Equal?(x=-1074360293, y=w1887) -> (x = y?=w1886:bool)
        n809 = feedback-in #2(w1877) -> ()
        n810 = call <vilib>:"IMAQdx Calculate Frames per Second.vi"("Session In"=w1932, "Buffer Number"=w1941, "Minimum Display Update Interval (ms)"=w1894, "Frames per Second Update Interval (ms)"=w1894, "Reset Counters"=w1893) -> ("Images Behind"=w1898:i32, "Images Missed"=w1899:u32)  [unwired: 4 in, 5 out]
        n811 = case shown="False" w1886 {
          tunnel: w1899 -> [w1948 _]
          frame False {
            "Images Missed" <- w1948
          }
          frame True {
          }
        }
        n812 = feedback #3(w1909) -> (w1907:T18)
        n813 = feedback-in #3(w1942) -> ()
        n814 = Divide(x=w1898, y=w1897) -> (x/y=w1896:dbl)
        n815 = Multiply(x=w1896, y=100.0) -> (x*y=w1884:dbl)
        "Video Buffer Fill Percent" <- w1884
        n816 = Select(t=w1909, s=w1893, f=w1907) -> (s? t:f=w1908:T18)
        n817 = Bundle By Name(cluster=cluster{"Image":T18, "Session":T2} {"Image"=refnum, "Session"=""}, "Image"=w1908, "Session"=w1932) -> (w1936:cluster{"Image":T18, "Session":T2})
        n818 = Not Equal?(x=w1908, y=w1909) -> (x != y?=w1924:bool)
        n819 = case shown="True" w1924 {
          tunnel: w1889 -> [w1970 w1990]
          tunnel: [w1970 w1988] -> w1874
          tunnel: w1873 -> [w1969 w1991]
          tunnel: w1936 -> [_ w1983]
          tunnel: [w1969 w1981] -> w1939
          tunnel: w1893 -> [_ w1976]
          tunnel: w1901 -> [w1968 w1974]
          tunnel: [w1968 w1973] -> w1900
          frame False {
          }
          frame True {
            w1971 = 0
            n820 = Unbundle By Name(w1991) -> ("AcquisitionSettings.FramesPerFile"=w1994:i32, "FileSettings.Format"=w1986:string)
            n821 = Increment(x=w1974) -> (x+1=w1973:i32)
            n822 = feedback #4(w1971) -> (w1977:i32)
            n823 = Select(t=w1971, s=w1976, f=w1977) -> (s? t:f=w1975:i32)
            n824 = Equal?(x=w1975, y=w1994) -> (x = y?=w1993:bool)
            n825 = case shown="False" w1993 {
              tunnel: [w2014 1] -> w1992
              tunnel: w1975 -> [w2015 _]
              tunnel: w1986 -> [_ w2020]
              tunnel: w1991 -> [w2013 w2019]
              tunnel: w1990 -> [w2012 w2018]
              tunnel: [w2012 w2017] -> w1987
              tunnel: [w2013 w2016] -> w1982
              frame False {
                n826 = Increment(x=w2015) -> (x+1=w2014:i32)
              }
              frame True {
                n827 = case shown="\"TDMS\", Default" w2020 {
                  tunnel: w2019 -> [w2025 w2029 w2038]
                  tunnel: w2018 -> [w2027 w2028 w2040]
                  tunnel: [w2023 w2028 w2032] -> w2017
                  tunnel: [w2022 w2029 w2042] -> w2016
                  frame "TDMS", Default {
                    n828 = Unbundle By Name(w2025) -> ("TDMSRef"=w2026:refnum<k34>)
                    n829 = call "TDMS Start New File.vi"("error in"=w2027, "Previous TDMS Refnum In"=w2026) -> ("error out"=w2023:errorcluster, "New TDMS Refnum Out"=w2024:refnum<k34>)  [unwired: 8 in]
                    n830 = Bundle By Name(cluster=w2025, "TDMSRef"=w2024) -> (w2022:T21)
                  }
                  frame "None" {
                  }
                  frame "AVI" {
                    n831 = Unbundle By Name(w2038) -> ("AVIRef"=w2041:T19)
                    n832 = Unbundle By Name(w2038) -> ("FileSettings"=w2037:T32)
                    n833 = call "IMAQ AVI2 Close"("error in (no error)"=w2040, "AVI Refnum"=w2041) -> ("error out"=w2039:errorcluster)  [unwired: 9 in]
                    n834 = Unbundle By Name(w2037) -> ("FileSaveLocation"=w2036:path, "AVI FPS"=w2035:i32, "Codec"=w2034:string, "Quality"=w2033:i32)
                    n835 = call "Increment Filename.vi"("Path In"=w2036) -> ("Incremented Path Out"=w2030:path)  [unwired: 10 in]
                    n836 = call "IMAQ AVI2 Create"("Quality"=w2033, "error in (no error)"=w2039, "Codec"=w2034, "Frames Per Second"=w2035, "AVI Path"=w2030) -> ("error out"=w2032:errorcluster, "AVI Refnum"=w2031:T19)  [unwired: 5 in]
                    n837 = Bundle By Name(cluster=w2038, "AVIRef"=w2031, "FileSettings.FileSaveLocation"=w2030) -> (w2042:T21)
                  }
                }
              }
            }
            n838 = feedback-in #4(w1992) -> ()
            n839 = Unbundle By Name(w1983) -> ("Session"=w1979:T2, "Image"=w1978:T18)
            n840 = call "High Resolution Timer Helper.vi"("error in (no error)"=w1987) -> ("error out"=w1985:errorcluster, "Current Time"=w1980:dbl)  [unwired: 8 in, 1 out]
            n841 = case shown="\"AVI\"" w1986 {
              tunnel: w1985 -> [w1996 w2003 w2011]
              tunnel: [w1996 w2002 w2010] -> w1984
              tunnel: w1978 -> [_ w2001 w2009]
              tunnel: w1982 -> [w1995 w1998 w2005]
              tunnel: [w1995 w1997 w2006] -> w1981
              frame "None", Default {
              }
              frame "AVI" {
                n842 = Unbundle By Name(w1998) -> ("AVIRef"=w2000:T19)
                n843 = call "IMAQ AVI2 Write Frame"("error in (no error)"=w2003, "Image"=w2001, "AVI Refnum"=w2000) -> ("error out"=w2002:errorcluster, "AVI Refnum (duplicate)"=w1999:T19)  [unwired: 6 in, 1 out]
                n844 = Bundle By Name(cluster=w1998, "AVIRef"=w1999) -> (w1997:T21)
              }
              frame "TDMS" {
                n845 = Unbundle By Name(w2005) -> ("TDMSRef"=w2008:refnum<k34>, "TDMSWSet"=w2007:T55)
                n846 = call "TDMS Write File.vi"("error in"=w2011, "Write Settings"=w2007, "Image"=w2009, "TDMS Ref In"=w2008) -> ("error out"=w2010:errorcluster, "TDMS Ref Out"=w2004:refnum<k34>)  [unwired: 6 in]
                n847 = Bundle By Name(cluster=w2005, "TDMSRef"=w2004) -> (w2006:T21)
              }
            }
            n848 = call "High Resolution Timer Helper.vi"("error in (no error)"=w1984, "Previous Time"=w1980) -> ("error out"=w1989:errorcluster, "Time Difference (ms)"=→"Write Speed (ms)":dbl)  [unwired: 7 in, 1 out]
            n849 = call <vilib>:"IMAQdx Release Image.vi"("error in"=w1989, "Image"=w1978, "Session In"=w1979) -> ("error out"=w1988:errorcluster)  [unwired: 7 in, 1 out]
          }
        }
        n850 = property on="Stop Acquisition on Full Buffer" class="Bool (strict)"() -> ("Value"=w1883:bool)  [unwired: 2 in, 2 out]
        n851 = Greater Or Equal?(x=w1884, y=95.0) -> (x >= y?=w1891:bool)
        n852 = feedback #5(w1902) -> (w1903:i32)
        n853 = Select(t=w1902, s=w1893, f=w1903) -> (s? t:f=w1912:i32)
        n854 = Equal?(x="Update Viewport Every N Frames", y=w1912) -> (x = y?=w1938:bool)
        n855 = And(x=w1891, y=w1883) -> (x .and. y?=w1871:bool)
        n856 = case shown="True" w1938 {
          tunnel: w1912 -> [w1963 _]
          tunnel: [w1962 1] -> w1937
          tunnel: w1936 -> [_ w1966]
          tunnel: [_ w1964] -> w1935
          frame False {
            n857 = Increment(x=w1963) -> (x+1=w1962:i32)
          }
          frame True {
            n858 = Unbundle By Name(w1966) -> ("Image"=w1965:T18)
            n859 = call <extravilib>:"Write.vi"("element"=w1965) -> ("channel"=w1964:T59)  [unwired: 8 in, 2 out]
          }
        }
        n860 = feedback-in #5(w1937) -> ()
        n861 = Unbundle By Name(w1889) -> ("code"=w1929:i32)
        n862 = Unbundle By Name(w1873) -> ("CameraSignalRefnum"=w1872:refnum<k21>)
        n863 = case shown="True" w1871 {
          frame False {
          }
          frame True {
            "BufferWasFull" <- TRUE ("BufferWasFull")
          }
        }
        n864 = Equal?(x=-1074360293, y=w1929) -> (x = y?=w1928:bool)
        n865 = case shown="False" w1928 {
          tunnel: ["Acquire" ("AfterErrorCheck") "Shutdown"] -> w1930
          frame False {
          }
          frame True {
          }
        }
        n866 = call <extravilib>:"Read.vi"("channel"=w1931) -> ("element"=w1875:bool)  [unwired: 1 in, 1 out]
        n867 = Unbundle By Name(w1913) -> ("TriggerStarted"=w1919:bool)
        n868 = Or(x=w1875, y=w1871) -> (x .or. y?=w1890:bool)
        n869 = And(x=w1919, y=w1890) -> (x .and. y?=w1918:bool)
        n870 = case shown="True" w1918 {
          tunnel: w1913 -> [w1950 w1957]
          tunnel: [w1950 w1955] -> w1906
          tunnel: [w1949 w1954] -> w1920
          tunnel: w1874 -> [w1949 w1952]
          tunnel: w1872 -> [_ w1953]
          frame False {
          }
          frame True {
            # "If stopped or signal error\nNeed to shut down signal\nimmediately to let buffer catch up"
            n871 = call <vilib>:"DAQmx Stop Task.vi"("task/channels in"=w1953, "error in"=w1952) -> ("task out"=w1959:refnum<k21>, "error out"=w1958:errorcluster)  [unwired: 12 in]
            n872 = call <vilib>:"DAQmx Clear Task.vi"("task in"=w1959, "error in"=w1958) -> ("error out"=w1954:errorcluster)  [unwired: 13 in]
            n873 = Bundle By Name(cluster=w1957, "TriggerStarted"=FALSE) -> (w1955:T17)
            n874 = property on="Shutting\nDown" class="Bool (strict)"("Value"=TRUE ("Shutting\nDown")) -> ()  [unwired: 2 in, 2 out]
          }
        }
        n875 = Merge Errors(w1920, w1874) -> (w1921:errorcluster)
        n876 = call <vilib>:"General Error Handler.vi"("type of dialog (OK msg:1)"=w1925, "error in (no error)"=w1921, "[exception action] (none:0)"=w1926, "[exception code]"=-1074360293 ("x")) -> ("error out"=w1882:errorcluster)  [unwired: 7 in, 4 out]
        n877 = Bundle By Name(cluster=w1906, "ResetAq?"=FALSE, "Frames"=w1900) -> (w1905:T17)
        n878 = call <extravilib>:"Write.vi"("element"=w1882) -> ("channel"=w1922:T46)  [unwired: 8 in, 2 out]
        n879 = call "High Resolution Timer Helper.vi"("error in (no error)"=w1882, "Previous Time"=w1876) -> ("error out"=w1881:errorcluster, "Time Difference (ms)"=→"Processing Speed (ms)":dbl)  [unwired: 7 in, 1 out]
        n880 = Select(t="Shutdown", s=w1882, f=w1930) -> (s? t:f=w1933:string)
      }
      frame "Shutdown" {
        n881 = Unbundle By Name(w2049) -> ("ShutdownActions"=w2047:string[])
        n882 = Empty Array?(array=w2047) -> (empty?=w2048:bool)
        n883 = case shown="True" w2048 {
          tunnel: w2049 -> [_ w2071]
          tunnel: [w2056 w2064] -> w2052
          tunnel: w2047 -> [w2056 w2070]
          frame False {
          }
          frame True {
            n884 = Unbundle By Name(w2071) -> ("TriggerStarted"=w2078:bool, "AcquisitionStarted"=w2077:bool, "Acquisition Configured"=w2076:bool, "FileOpen"=w2075:bool, "CameraOpen"=w2074:bool, "BufferOpen"=w2067:bool, "AcStarted"=w2060:bool, "VideoSave"=w2057:bool)
            n885 = Not(x=w2060) -> (.not. x?=w2059:bool)
            n886 = Build Array("ShutdownTrigger", "ShutdownAcquisition", "UnconfigureAcquisition", "CloseFile", "ShutdownCamera", "ReleaseBuffer", "ReleaseRendezvous", "WriteTimingFile" ("element")) -> (w2073:string[])
            n887 = Build Array(w2078, w2077, w2076, w2075, w2074, w2067, w2059, w2057) -> (w2072:bool[])
            n888 = for {
              tunnel: w2073 -> [w2083] mode=indexing
              tunnel: w2072 -> [w2084] mode=indexing
              shift-right: [w2081] -> w2069
              shift-left: w2070 -> [w2082]
              n889 = case shown="True" w2084 {
                tunnel: w2083 -> [_ w2088]
                tunnel: w2082 -> [w2085 w2087]
                tunnel: [w2085 w2086] -> w2081
                frame False {
                }
                frame True {
                  n890 = Insert Into Array(array=w2087, new element=w2088) -> (w2086:string[])  [unwired: 1 in]
                }
              }
            }
            n891 = Insert Into Array(array=w2069, new element="FinalErrorHandler" ("new element/subarray")) -> (w2064:string[])  [unwired: 1 in]
          }
        }
        n892 = property on="Video Buffer Fill Percent" class="Slide (strict)"("Value"=0.0 ("Video Buffer Fill Percent")) -> ()  [unwired: 2 in, 2 out]
        n893 = property on="Shutting\nDown" class="Bool (strict)"("Value"=TRUE ("Shutting\nDown")) -> ()  [unwired: 2 in, 2 out]
        n894 = Delete From Array(array=w2052, index=0) -> (deleted portion=w2051:string, array with subset deleted=w2050:string[])  [unwired: 1 in]
        n895 = Bundle By Name(cluster=w2049, "ShutdownActions"=w2050, "ResetAq?"=TRUE) -> (w2055:T17)
      }
      frame "ShutdownTrigger " {
        n896 = Unbundle By Name(w2092) -> ("CameraSignalRefnum"=w2095:refnum<k21>)
        n897 = call <vilib>:"DAQmx Stop Task.vi"("task/channels in"=w2095, "error in"=w2094) -> ("task out"=w2098:refnum<k21>, "error out"=w2097:errorcluster)  [unwired: 12 in]
        n898 = call <vilib>:"DAQmx Clear Task.vi"("task in"=w2098, "error in"=w2097) -> ("error out"=w2093:errorcluster)  [unwired: 13 in]
        n899 = Bundle By Name(cluster=w2091, "TriggerStarted"=FALSE) -> (w2090:T17)
      }
      frame "ShutdownAcquisition" {
        n900 = Unbundle By Name(w2106) -> ("IMAQdx Session"=w2108:T2)
        n901 = flat-sequence {
          tunnel: w2108 -> [w2113]
          tunnel: [w2112] -> w2107
          tunnel: w2104 -> [w2111]
          tunnel: [w2110] -> w2103
          frame #0 {
            n902 = call <vilib>:"IMAQdx Stop Acquisition.vi"("error in"=w2111, "Session In"=w2113) -> ("error out"=w2110:errorcluster, "Session Out"=w2112:T2)  [unwired: 8 out]
            n903 = Wait (ms)(milliseconds to wait=u32 10) -> ()  [unwired: 1 out]
          }
        }
        n904 = Bundle By Name(cluster=w2106, "IMAQdx Session"=w2107) -> (w2105:T21)
        n905 = Bundle By Name(cluster=w2101, "AcquisitionStarted"=FALSE) -> (w2099:T17)
      }
      frame "UnconfigureAcquisition" {
        n906 = Unbundle By Name(w2120) -> ("IMAQdx Session"=w2122:T2)
        n907 = call <vilib>:"IMAQdx Unconfigure Acquisition.vi"("error in"=w2116, "Session In"=w2122) -> ("error out"=w2117:errorcluster, "Session Out"=w2121:T2)  [unwired: 8 out]
        n908 = Bundle By Name(cluster=w2120, "IMAQdx Session"=w2121) -> (w2119:T21)
        n909 = Bundle By Name(cluster=w2115, "Acquisition Configured"=FALSE) -> ()  [unwired: 1 out]
      }
      frame "CloseFile" {
        n910 = Unbundle By Name(w2126) -> ("FileSettings.Format"=w2128:string)
        n911 = case shown="\"AVI\", Default" w2128 {
          tunnel: w2130 -> [w2134 w2138 w2140]
          tunnel: [w2131 w2137 w2140] -> w2129
          tunnel: w2126 -> [w2133 w2136 _]
          frame "AVI", Default {
            n912 = Unbundle By Name(w2133) -> ("AVIRef"=w2132:T19)
            n913 = call "IMAQ AVI2 Close"("error in (no error)"=w2134, "AVI Refnum"=w2132) -> ("error out"=w2131:errorcluster)  [unwired: 9 in]
          }
          frame "TDMS" {
            n914 = Unbundle By Name(w2136) -> ("TDMSRef"=w2135:refnum<k34>)
            n915 = TDMS Advanced Close(6:10.0 ("timeout (10 s)"), 8:w2138, 11:w2135) -> (0:w2137:errorcluster)  [unwired: 1 in, 1 out]
          }
          frame "None" {
          }
        }
        n916 = Bundle By Name(cluster=w2125, "FileOpen"=FALSE ("FileCreated")) -> (w2124:T17)
      }
      frame "ShutdownCamera" {
        n917 = Unbundle By Name(w2142) -> ("IMAQdx Session"=w2143:T2)
        n918 = call <vilib>:"IMAQdx Close Camera.vi"("error in"=w2148, "Session In"=w2143) -> ("error out"=w2141:errorcluster)  [unwired: 9 out]
        n919 = Bundle By Name(cluster=w2146, "CameraOpen"=FALSE) -> (w2144:T17)
      }
      frame "ReleaseBuffer" {
        n920 = Unbundle By Name(w2154) -> ("Image Buffer"=w2156:T18[])
        n921 = for {
          shift-right: [w2158] -> w2149
          shift-left: w2150 -> [w2159]
          tunnel: w2156 -> [w2157] mode=indexing
          n922 = call "IMAQ Dispose"("Image"=w2157, "error in (no error)"=w2159) -> ("error out"=w2158:errorcluster)  [unwired: 4 in]
        }
        n923 = Bundle By Name(cluster=w2153, "BufferOpen"=FALSE) -> (w2151:T17)
      }
      frame "ReleaseRendezvous" {
        n924 = Unbundle By Name(w2164) -> ("rendezvous ref"=w2165:T7)
        n925 = call <vilib>:"Wait at Rendezvous.vi"("error in (no error)"=w2161, "rendezvous"=w2165) -> ("error out"=w2160:errorcluster)  [unwired: 3 in, 2 out]
      }
      frame "WriteTimingFile" {
        n926 = Unbundle By Name(w2185) -> ("Frames"=w2186:i32)
        n927 = property on="Include Camera Signal Output File" class="Bool (strict)"() -> ("Value"=w2178:bool)  [unwired: 2 in, 2 out]
        n928 = property on="File Time Resolution (s)" class="DigNum (strict)"() -> ("Value"=w2177:dbl)  [unwired: 2 in, 2 out]
        n929 = Unbundle By Name(w2180) -> ("CameraSignalDefinition"=w2187:T57, "Camera Attributes.Exposure Start Delay"=w2200:dbl)
        n930 = Unbundle By Name(w2187) -> ("Delay"=w2198:dbl, "High Time"=w2196:dbl, "Low Time"=w2197:dbl)
        n931 = Add(x=w2196, y=w2197) -> (x+y=w2195:dbl)
        n932 = Subtract(x=w2196, y=w2200) -> (x-y=w2202:dbl)
        n933 = Divide(x=w2202, y=2.0) -> (x/y=w2199:dbl)
        n934 = for {
          N: w2186 -> [_]
          tunnel: w2200 -> [w2260]
          tunnel: w2199 -> [w2261]
          tunnel: w2198 -> [w2258]
          tunnel: w2195 -> [w2256]
          tunnel: [w2251] -> w2194 mode=indexing
          i -> [w2257]
          n935 = Add(x=w2260, y=w2261) -> (x+y=w2259:dbl)
          n936 = Add(x=w2258, y=w2259) -> (x+y=w2255:dbl)
          n937 = Multiply(x=w2256, y=w2257) -> (x*y=w2254:dbl)
          n938 = Add(x=w2254, y=w2255) -> (x+y=w2253:dbl)
          n939 = Format Value(format string="%.9f", value (0)=w2253) -> (output string=w2251:string)  [unwired: 1 in]
        }
        n940 = Unbundle By Name(w2180) -> ("FileSettings.FileSaveLocation"=w2189:path, "FileSettings.TimingSuffix"=w2188:string, "FileSettings.FileName"=w2176:string)
        n941 = case shown="False" w2178 {
          tunnel: w2189 -> [_ w2245]
          tunnel: w2188 -> [_ w2244]
          tunnel: w2187 -> [_ w2233]
          tunnel: w2186 -> [_ w2223]
          tunnel: w2184 -> [w2206 w2219]
          tunnel: [w2206 w2216] -> w2182
          tunnel: w2177 -> [_ w2212]
          tunnel: w2177 -> [_ w2211]
          tunnel: w2176 -> [_ w2210]
          frame False {
          }
          frame True {
            w2225 = cluster{"Sample Rate":dbl, "Samples":dbl} {"Sample Rate"=0.0, "Samples"=0.0}
            w2231 = 2.5 ("offset")
            # "Frequency"
            # "Period"
            # "Camera Amplitude from 0 to 5V"
            # "Signal Delay"
            n942 = Unbundle By Name(w2233) -> ("Delay"=w2235:dbl)
            n943 = Reciprocal(x=w2212) -> (1/x=w2214:dbl)
            n944 = Multiply(x=w2235, y=w2214) -> (x*y=w2236:dbl)
            n945 = Bundle By Name(cluster=w2225, "Sample Rate"=w2214, "Samples"=w2236) -> (w2237:cluster{"Sample Rate":dbl, "Samples":dbl})
            n946 = call <vilib>:"Square Waveform.vi"("sampling info"=w2237, "error in (no error)"=w2219, "amplitude"=0.0, "frequency"=1.0) -> ("error out"=w2218:errorcluster, "signal out"=w2234:waveform(dbl))  [unwired: 6 in]
            n947 = Unbundle By Name(w2233) -> ("High Time"=w2230:dbl, "Low Time"=w2232:dbl)
            n948 = Add(x=w2230, y=w2232) -> (x+y=w2229:dbl)
            n949 = Reciprocal(x=w2211) -> (1/x=w2213:dbl)
            n950 = Divide(x=w2230, y=w2229) -> (x/y=w2228:dbl)
            n951 = Multiply(x=w2228, y=100.0) -> (x*y=w2226:dbl)
            n952 = Reciprocal(x=w2229) -> (1/x=w2220:dbl)
            n953 = Multiply(x=w2220, y=w2213) -> (x*y=w2222:dbl)
            n954 = Multiply(x=w2222, y=w2223) -> (x*y=w2221:dbl)
            n955 = Bundle By Name(cluster=w2225, "Sample Rate"=w2213, "Samples"=w2221) -> (w2224:cluster{"Sample Rate":dbl, "Samples":dbl})
            n956 = call <vilib>:"Square Waveform.vi"("duty cycle (%)"=w2226, "offset"=w2231, "sampling info"=w2224, "error in (no error)"=w2218, "amplitude"=w2231, "frequency"=w2220) -> ("error out"=w2217:errorcluster, "signal out"=w2239:waveform(dbl))  [unwired: 4 in]
            n957 = call-poly <vilib>:"Append Waveforms.vi"("waveform B"=w2239, "waveform A"=w2234) -> ("waveform out"=w2240:waveform(dbl))  [unwired: 8 in, 1 out]
            n958 = Concatenate Strings(w2210, w2244, "_Signal.tdms" ("string")) -> (w2246:string)
            n959 = Build Path(base path=w2245, name or relative path=w2246) -> (appended path=w2243:path)
            n960 = TDMS Open(8:w2217, 10:T48."open or create" ("operation (0:open)"), 11:w2243) -> (0:w2208:errorcluster, 3:w2207:refnum<k34>)  [unwired: 4 in]
            n961 = TDMS Write(0:w2207, 9:w2240, 11:w2208) -> (4:w2241:refnum<k34>, 15:w2242:errorcluster)  [unwired: 3 in, 2 out]
            n962 = TDMS Close(8:w2242, 11:w2241) -> (0:w2216:errorcluster)  [unwired: 1 out]
          }
        }
        n963 = for {
          N: w2186 -> [_]
          tunnel: [w2248] -> w2193 mode=indexing
          i -> [w2250]
          n964 = Format Value(format string="%d", value (0)=w2250) -> (output string=w2248:string)  [unwired: 1 in]
        }
        n965 = Concatenate Strings(w2176, w2188, ".csv" ("string")) -> (w2190:string)
        n966 = Build Array(w2193, w2194) -> (w2192:string[][])
        n967 = Build Path(base path=w2189, name or relative path=w2190) -> (appended path=w2167:path)
        n968 = Open/Create/Replace File(file path (use dialog)=w2167, operation (0:open)=T23."replace or create") -> (refnum out=w2174:refnum<file>, error out=w2173:errorcluster)  [unwired: 4 in, 1 out]
        n969 = Concatenate Strings("FrameNo,Time (s)" ("text"), "\r") -> (w2171:string)
        n970 = Write to Text File(file (use dialog)=w2174, text=w2171, error in=w2173) -> (refnum out=w2168:refnum<file>, error out=w2169:errorcluster)  [unwired: 1 in, 1 out]
        n971 = Close File(refnum=w2168, error in=w2169) -> (path=w2166:path)  [unwired: 1 out]
        n972 = call-poly <vilib>:"Write Delimited Spreadsheet.vi"("file path (dialog if empty)"=w2166, "2D data"=w2192, "append to file? (new file:F)"=FALSE, "transpose? (no:F)"=TRUE, "delimiter (\\t)"="," ("delimiter (\\t)")) -> ("error out"=w2181:errorcluster)  [unwired: 9 in, 1 out]
        n973 = Merge Errors(w2182, w2181) -> (w2183:errorcluster)
      }
      frame "FinalErrorHandler" {
        n974 = call <vilib>:"Simple Error Handler.vi"("error in (no error)"=w2266) -> ("error out"=w2262:errorcluster)  [unwired: 4 in, 4 out]
      }
    }
    n975 = call <extravilib>:"Read.vi"("channel"=w1460) -> ("element"=w1459:bool)  [unwired: 1 in, 1 out]
  }
  n976 = while {
    shift-right: [w2283] -> _
    shift-left: "Idle" ("AfterErrorCheck") -> [w2282]
    shift-right: [w2280] -> _
    shift-left: errorcluster {"status"=FALSE, "code"=0, "source"=""} ("error IO") -> [w2279]
    shift-right: [w2278] -> _
    shift-left: T16 {"Physical Settings"={"physical channels"="Dev1/ao0:2", "source"="OnboardClock", "Start Trigger"="/Dev1/ai/StartTrigger", "StartTriggered"=TRUE}, "OutputTask"="", "GenerationSettings"={"NumberOfSamples"=10000, "Sample Rate"=50000, "SampleBuffer"=100000}, "Channel Names"="", "FileSettings"={"Path"=path "E:/Jacob", "File"="Test3", "FileFormat"=enum."TDMS", "FileSuffix"="_Data_Output", "Multiple Time Columns"=TRUE}} -> [w2281]
    shift-right: [w2276] -> _
    shift-left: w12 -> [w2277]
    tunnel: w13 -> [w2275]
    tunnel: w35 -> [w2274]
    tunnel: w3 -> [w2273]
    tunnel: w24 -> [w2272]
    tunnel: w23 -> [w2271]
    tunnel: [w2270] -> w19
    tunnel: w16 -> [w2268]
    tunnel: w4 -> [w2267]
    stop <- w2269 stop-if-true
    # "Analog Output"
    n977 = call <extravilib>:"Write.vi"("element"=w2282) -> ("channel"=w2270:T49)  [unwired: 1 out]
    n978 = case shown="\"Idle\", Default" w2282 {
      tunnel: ["InitializeFile" w2316 "InitializeSignal" ("AfterErrorCheck") "InitializeSignal" ("AfterErrorCheck") "ErrorCheck" ("AfterErrorCheck") "Generate" ("AfterErrorCheck") w2467 "FinalErrorCheck" "Idle" ("AfterErrorCheck") w2545 "InitializeChannels"] -> w2283
      tunnel: w2281 -> [w2298 w2314 w2325 w2341 w2368 w2403 w2469 w2513 w2541 w2546 w2564]
      tunnel: [w2301 w2313 w2328 w2338 w2354 w2401 w2462 w2515 w2539 w2544 errorcluster {"status"=FALSE, "code"=0, "source"=""} ("error IO")] -> w2280
      tunnel: w2279 -> [w2285 w2313 w2320 w2338 w2373 w2405 w2474 w2517 w2540 w2550 _]
      tunnel: [w2299 w2314 w2325 w2341 w2369 w2402 w2470 w2513 w2541 w2546 w2576] -> w2278
      tunnel: w2277 -> [w2296 w2315 w2331 w2343 w2371 w2398 w2472 w2514 w2542 w2543 w2574]
      tunnel: [w2296 w2315 w2330 w2342 w2366 w2396 w2453 w2507 w2542 w2547 w2572] -> w2276
      tunnel: [_ _ _ _ _ _ w2466 _ _ w2549 _] -> w2275
      tunnel: w2274 -> [_ _ _ _ _ _ w2465 _ _ w2548 _]
      tunnel: w2273 -> [_ _ _ _ _ _ w2461 _ _ _ _]
      tunnel: w2272 -> [_ _ _ _ _ _ _ _ _ _ w2582]
      tunnel: w2271 -> [_ _ _ _ _ _ _ _ _ _ w2581]
      tunnel: [_ _ _ _ _ _ w2449 _ _ _ _] -> w2267
      frame "InitializeChannels" {
        w2292 = 10123 items=["Finite Samples"=10178, "Continuous Samples"=10123, "Hardware Timed Single Point"=12522] ("sample mode")
        n979 = Unbundle By Name(w2298) -> ("Physical Settings"=w2291:T38, "Channel Names"=w2293:string, "GenerationSettings.Sample Rate"=w2295:i32, "GenerationSettings.SampleBuffer"=w2294:i32, "OutputTask"=w2284:refnum<k21>)
        n980 = Unbundle By Name(w2291) -> ("physical channels"=w2290:tag, "source"=w2288:tag, "Start Trigger"=w2287:tag, "StartTriggered"=w2289:bool)
        n981 = call <vilib>:"DAQmx Clear Task.vi"("task in"=w2284, "error in"=w2285) -> ("error out"=w2286:errorcluster)  [unwired: 13 in]
        n982 = call-poly <vilib>:"DAQmx Create Virtual Channel.vi"("task in"=w2284, "physical channels"=w2290, "name to assign"=w2293, "error in"=w2286) -> ("task out"=w2304:refnum<k21>, "error out"=w2305:errorcluster)  [unwired: 10 in]
        n983 = call-poly <vilib>:"DAQmx Timing.vi"("task/channels in"=w2304, "sample mode"=w2292, "samples per channel"=w2294, "rate"=w2295, "source"=w2288, "error in"=w2305) -> ("task out"=w2303:refnum<k21>, "error out"=w2302:errorcluster)  [unwired: 8 in]
        n984 = case shown="True" w2289 {
          tunnel: w2303 -> [w2306 w2312]
          tunnel: w2302 -> [w2307 w2311]
          tunnel: w2287 -> [_ w2310]
          tunnel: [w2307 w2308] -> w2301
          tunnel: [w2306 w2309] -> w2297
          frame False {
          }
          frame True {
            n985 = call-poly <vilib>:"DAQmx Trigger.vi"("task/channels in"=w2312, "source"=w2310, "error in"=w2311) -> ("task out"=w2309:refnum<k21>, "error out"=w2308:errorcluster)  [unwired: 11 in]
          }
        }
        n986 = Bundle By Name(cluster=w2298, "OutputTask"=w2297) -> (w2299:T16)
      }
      frame "InitializeFile" {
        n987 = Unbundle By Name(w2314) -> ("FileSettings.FileFormat"=w2317:enum16{"TDMS", "CSV"})
        n988 = case shown="\"TDMS\", Default" w2317 {
          tunnel: ["InitializeTDMS" ("AfterErrorCheck") "InitializeCSV" ("AfterErrorCheck")] -> w2316
          frame "TDMS", Default {
          }
          frame "CSV" {
          }
        }
      }
      frame "InitializeTDMS" {
        n989 = Unbundle By Name(w2325) -> ("FileSettings.Path"=w2321:path, "FileSettings.File"=w2322:string, "FileSettings.FileSuffix"=w2327:string)
        n990 = Concatenate Strings(w2322, w2327, ".tdms" ("string")) -> (w2326:string)
        n991 = Build Path(base path=w2321, name or relative path=w2326) -> (appended path=w2324:path)
        n992 = TDMS Open(8:w2320, 10:T48."open or create" ("operation (0:open)"), 11:w2324) -> (0:w2335:errorcluster, 3:w2332:refnum<k34>)  [unwired: 4 in]
        n993 = TDMS Set Properties(5:string[] ["Data"] ("property values"), 7:string[] ["Title"] ("property names"), 8:w2335, 11:w2332) -> (0:w2328:errorcluster, 3:w2329:refnum<k34>)  [unwired: 2 in, 2 out]
        n994 = Bundle By Name(cluster=w2331, "TDMSRef"=w2329) -> (w2330:T15)
      }
      frame "InitializeCSV" {
        n995 = Unbundle By Name(w2341) -> ("FileSettings.Path"=w2340:path, "FileSettings.File"=w2347:string, "FileSettings.FileSuffix"=w2346:string)
        n996 = Concatenate Strings(w2347, w2346, ".csv" ("string")) -> (w2345:string)
        n997 = Build Path(base path=w2340, name or relative path=w2345) -> (appended path=w2339:path)
        n998 = Bundle By Name(cluster=w2343, "CSV path"=w2339) -> (w2342:T15)
      }
      frame "InitializeSignal" {
        n999 = Unbundle By Name(w2368) -> ("GenerationSettings.NumberOfSamples"=w2361:i32, "OutputTask"=w2363:refnum<k21>, "Channel Names"=w2358:string, "FileSettings"=w2352:T36)
        n1000 = property class="DAQmx Timing"(reference=w2363, error in=w2373) -> (error out=w2375:errorcluster, "SampClk.Rate"=w2355:dbl)  [unwired: 1 out]
        n1001 = call <vilib>:"Delimited String to 1D String Array.vi"("delimiter"=",", "delimited string"=w2358) -> ("string array"=w2360:string[])  [unwired: 9 in]
        n1002 = Unbundle By Name(w2371) -> ("PreviousInfo"=w2372:T60)
        n1003 = property on="Outputs" class="Clust (strict)"() -> ("Value"=w2362:T61)  [unwired: 2 in, 2 out]
        n1004 = call "GenerateOutputSignal (SubVI).vi"("PreviousInfoIn"=w2372, "Checkbox"=TRUE ("reset signal"), "error constant"=w2375, "#s"=w2361, "Fs"=w2355, "Outputs"=w2362) -> ("error constant 2"=w2374:errorcluster, "PreviousInfoOut"=w2370:T60, "Array 2"=w2357:waveform(dbl)[])  [unwired: 3 in]
        n1005 = for {
          tunnel: w2360 -> [w2392] mode=indexing
          tunnel: w2357 -> [w2391] mode=indexing
          tunnel: [w2390] -> w2351 mode=indexing
          n1006 = Set Waveform Attribute(5:w2392, 6:"NI_ChannelName" ("name"), 7:w2391) -> (3:w2390:waveform(dbl))  [unwired: 1 in, 2 out]
        }
        n1007 = Bundle By Name(cluster=w2371, "PreviousInfo"=w2370) -> (w2350:T15)
        n1008 = call-poly <vilib>:"DAQmx Write.vi"("task/channels in"=w2363, "data"=w2357, "error in"=w2374) -> ("task out"=w2367:refnum<k21>, "error out"=w2354:errorcluster)  [unwired: 10 in, 1 out]
        n1009 = Unbundle By Name(w2352) -> ("FileFormat"=w2353:enum16{"TDMS", "CSV"})
        n1010 = case shown="\"TDMS\", Default" w2353 {
          tunnel: w2350 -> [w2381 w2389]
          tunnel: w2351 -> [w2379 w2387]
          tunnel: w2350 -> [w2378 w2382]
          tunnel: [w2376 w2382] -> w2349
          frame "TDMS", Default {
            n1011 = Unbundle By Name(w2381) -> ("TDMSRef"=w2380:refnum<k34>)
            n1012 = TDMS Write(0:w2380, 9:w2379) -> (4:w2377:refnum<k34>)  [unwired: 4 in, 3 out]
            n1013 = Bundle By Name(cluster=w2378, "TDMSRef"=w2377) -> (w2376:T15)
          }
          frame "CSV" {
            n1014 = Unbundle By Name(w2389) -> ("CSV path"=w2388:path)
            n1015 = call-poly <vilib>:"Export Waveforms to Spreadsheet File.vi"("header? (write header:T)"=TRUE, "delimiter (Tab)"=",", "append to file? (new file:F)"=FALSE, "multiple time columns? (single:F)"=TRUE, "waveforms"=w2387, "file path (dialog if empty)"=w2388) -> ()  [unwired: 4 in, 2 out]
          }
        }
        n1016 = Bundle By Name(cluster=w2368, "OutputTask"=w2367) -> (w2369:T16)
        n1017 = Bundle By Name(cluster=w2349, "AfterErrorCheck"="WaitForAcStart", "PrevousWave"=w2351) -> (w2366:T15)
      }
      frame "WaitForAcStart" {
        n1018 = Unbundle By Name(w2398) -> ("SyncStart"=w2407:bool, "Leader"=w2400:bool, "rendezvous ref"=w2399:T7)
        n1019 = Unbundle By Name(w2403) -> ("OutputTask"=w2406:refnum<k21>)
        n1020 = case shown="True" w2407 {
          tunnel: w2406 -> [w2412 w2417]
          tunnel: w2405 -> [w2411 w2418]
          tunnel: [w2410 w2415] -> w2404
          tunnel: [w2409 w2416] -> w2401
          tunnel: w2400 -> [_ w2419]
          tunnel: w2399 -> [_ w2414]
          tunnel: [TRUE ("AcStarted") w2413] -> w2394
          frame False {
            n1021 = call <vilib>:"DAQmx Start Task.vi"("task/channels in"=w2412, "error in"=w2411) -> ("task out"=w2410:refnum<k21>, "error out"=w2409:errorcluster)  [unwired: 12 in]
          }
          frame True {
            n1022 = case shown="False" w2419 {
              tunnel: w2418 -> [w2425 w2434]
              tunnel: w2417 -> [w2424 w2435]
              tunnel: [w2423 w2432] -> w2416
              tunnel: [w2422 w2433] -> w2415
              tunnel: w2414 -> [w2421 w2436]
              tunnel: [TRUE ("AcStarted") TRUE ("AcStarted")] -> w2413
              frame False {
                n1023 = flat-sequence {
                  tunnel: w2425 -> [w2429]
                  tunnel: w2424 -> [w2428]
                  tunnel: [w2427] -> w2423
                  tunnel: [w2426] -> w2422
                  tunnel: w2421 -> [w2430]
                  frame #0 {
                    n1024 = call <vilib>:"DAQmx Start Task.vi"("task/channels in"=w2428, "error in"=w2429) -> ("task out"=w2426:refnum<k21>, "error out"=w2427:errorcluster)  [unwired: 12 in]
                  }
                  frame #1 {
                    n1025 = call <vilib>:"Wait at Rendezvous.vi"("rendezvous"=w2430) -> ()  [unwired: 4 in, 3 out]
                  }
                  frame #2 {
                  }
                }
              }
              frame True {
                n1026 = flat-sequence {
                  tunnel: w2436 -> [w2437]
                  tunnel: w2435 -> [w2441]
                  tunnel: w2434 -> [w2439]
                  tunnel: [w2440] -> w2433
                  tunnel: [w2438] -> w2432
                  frame #0 {
                    n1027 = call <vilib>:"Wait at Rendezvous.vi"("rendezvous"=w2437) -> ()  [unwired: 4 in, 3 out]
                  }
                  frame #1 {
                    n1028 = call <vilib>:"DAQmx Start Task.vi"("task/channels in"=w2441, "error in"=w2439) -> ("task out"=w2440:refnum<k21>, "error out"=w2438:errorcluster)  [unwired: 12 in]
                  }
                }
              }
            }
          }
        }
        n1029 = Bundle By Name(cluster=w2403, "OutputTask"=w2404) -> (w2402:T16)
        n1030 = Bundle By Name(cluster=w2398, "Started?"=TRUE, "AcStarted"=w2394) -> (w2396:T15)
      }
      frame "Generate" {
        n1031 = Unbundle By Name(w2469) -> ("GenerationSettings.NumberOfSamples"=w2459:i32, "OutputTask"=w2457:refnum<k21>, "Channel Names"=w2456:string, "FileSettings.FileFormat"=w2443:enum16{"TDMS", "CSV"})  [unwired: 1 out]
        n1032 = call <extravilib>:"Write.vi"("element"=w2464) -> ("channel"=w2466:T46)  [unwired: 8 in, 2 out]
        n1033 = property class="DAQmx Timing"(reference=w2457, error in=w2474) -> (reference out=w2475:refnum<k21>, error out=w2477:errorcluster, "SampClk.Rate"=w2447:dbl)
        "Actual Sample Rate" <- w2447
        n1034 = call <vilib>:"Delimited String to 1D String Array.vi"("delimiter"=",", "delimited string"=w2456) -> ("string array"=w2454:string[])  [unwired: 9 in]
        n1035 = Unbundle By Name(w2472) -> ("PreviousInfo"=w2473:T60, "PrevousWave"=w2450:waveform(dbl)[])
        n1036 = property on="Outputs" class="Clust (strict)"() -> ("Value"=w2460:T61)  [unwired: 2 in, 2 out]
        n1037 = call "GenerateOutputSignal (SubVI).vi"("PreviousInfoIn"=w2473, "Checkbox"=FALSE ("reset signal"), "error constant"=w2477, "#s"=w2459, "Fs"=w2447, "Outputs"=w2460) -> ("error constant 2"=w2476:errorcluster, "PreviousInfoOut"=w2471:T60, "Array 2"=w2446:waveform(dbl)[])  [unwired: 3 in]
        n1038 = for {
          tunnel: w2454 -> [w2503] mode=indexing
          tunnel: w2446 -> [w2502] mode=indexing
          tunnel: [w2501] -> w2442 mode=indexing
          n1039 = Set Waveform Attribute(5:w2503, 6:"NI_ChannelName" ("name"), 7:w2502) -> (3:w2501:waveform(dbl))  [unwired: 1 in, 2 out]
        }
        n1040 = Bundle By Name(cluster=w2472, "PreviousInfo"=w2471) -> (w2445:T15)
        n1041 = flat-sequence {
          tunnel: w2476 -> [w2496]
          tunnel: w2475 -> [w2495]
          tunnel: w2446 -> [w2492]
          tunnel: [w2494] -> w2452
          tunnel: [w2493] -> w2451
          tunnel: [w2499] -> w2464
          tunnel: [w2500] -> w2468
          tunnel: w2452 -> [w2500]
          tunnel: w2451 -> [w2499]
          tunnel: w2450 -> [w2498]
          tunnel: [w2497] -> w2449
          frame #0 {
            n1042 = call-poly <vilib>:"DAQmx Write.vi"("task/channels in"=w2495, "data"=w2492, "error in"=w2496) -> ("task out"=w2494:refnum<k21>, "error out"=w2493:errorcluster)  [unwired: 10 in, 1 out]
          }
          frame #1 {
            n1043 = call <extravilib>:"Write.vi"("element"=w2498) -> ("channel"=w2497:T50)  [unwired: 8 in, 2 out]
          }
        }
        n1044 = case shown="\"TDMS\", Default" w2443 {
          tunnel: w2442 -> [w2482 w2490]
          tunnel: w2445 -> [w2481 w2485]
          tunnel: [w2479 w2485] -> w2444
          tunnel: w2445 -> [w2478 w2484]
          frame "TDMS", Default {
            n1045 = Unbundle By Name(w2478) -> ("TDMSRef"=w2483:refnum<k34>)
            n1046 = TDMS Write(0:w2483, 9:w2482) -> (4:w2480:refnum<k34>)  [unwired: 4 in, 3 out]
            n1047 = Bundle By Name(cluster=w2481, "TDMSRef"=w2480) -> (w2479:T15)
          }
          frame "CSV" {
            n1048 = Unbundle By Name(w2484) -> ("CSV path"=w2491:path)
            n1049 = call-poly <vilib>:"Export Waveforms to Spreadsheet File.vi"("header? (write header:T)"=TRUE, "delimiter (Tab)"=",", "append to file? (new file:F)"=TRUE, "multiple time columns? (single:F)"=TRUE, "waveforms"=w2490, "file path (dialog if empty)"=w2491) -> ()  [unwired: 4 in, 2 out]
          }
        }
        n1050 = Bundle By Name(cluster=w2444, "PrevousWave"=w2442) -> (w2453:T15)
        n1051 = Bundle By Name(cluster=w2469, "OutputTask"=w2468) -> (w2470:T16)
        n1052 = call <extravilib>:"Read.vi"("channel"=w2461) -> ("element"=w2458:bool)  [unwired: 1 in, 1 out]
        n1053 = case shown="False" w2458 {
          tunnel: ["Shutdown" "Generate"] -> w2467
          frame True {
          }
          frame False {
          }
        }
        n1054 = call <extravilib>:"Read.vi"("channel"=w2465) -> ("element"=w2463:errorcluster)  [unwired: 1 in, 1 out]
        n1055 = Merge Errors(w2464, w2463) -> (w2462:errorcluster)
      }
      frame "Shutdown" {
        n1056 = Unbundle By Name(w2513) -> ("OutputTask"=w2519:refnum<k21>, "FileSettings.FileFormat"=w2508:enum16{"TDMS", "CSV"})
        n1057 = Unbundle By Name(w2514) -> ("Started?"=w2520:bool, "AcStarted"=w2511:bool, "rendezvous ref"=w2510:T7)
        n1058 = case shown="False" w2520 {
          tunnel: w2519 -> [w2530 w2537]
          tunnel: [w2530 w2536] -> w2518
          tunnel: w2517 -> [w2529 w2535]
          tunnel: [w2529 w2534] -> w2516
          tunnel: w2514 -> [w2528 w2533]
          tunnel: [w2528 w2532] -> w2509
          frame False {
          }
          frame True {
            n1059 = call <vilib>:"DAQmx Stop Task.vi"("task/channels in"=w2537, "error in"=w2535) -> ("task out"=w2536:refnum<k21>, "error out"=w2534:errorcluster)  [unwired: 12 in]
            n1060 = Bundle By Name(cluster=w2533, "Started?"=FALSE) -> (w2532:T15)
          }
        }
        n1061 = call <vilib>:"DAQmx Clear Task.vi"("task in"=w2518, "error in"=w2516) -> ("error out"=w2515:errorcluster)  [unwired: 13 in]
        n1062 = case shown="False" w2511 {
          tunnel: w2510 -> [w2524 _]
          tunnel: w2509 -> [w2523 w2527]
          tunnel: [w2523 w2525] -> w2507
          frame False {
            n1063 = call <vilib>:"Wait at Rendezvous.vi"("rendezvous"=w2524) -> ()  [unwired: 4 in, 3 out]
          }
          frame True {
            n1064 = Bundle By Name(cluster=w2527, "AcStarted"=FALSE) -> (w2525:T15)
          }
        }
        n1065 = case shown="\"TDMS\", Default" w2508 {
          tunnel: w2507 -> [w2522 _]
          frame "TDMS", Default {
            n1066 = Unbundle By Name(w2522) -> ("TDMSRef"=w2521:refnum<k34>)
            n1067 = TDMS Close(11:w2521) -> ()  [unwired: 1 in, 2 out]
          }
          frame "CSV" {
          }
        }
      }
      frame "FinalErrorCheck" {
        n1068 = call <vilib>:"Simple Error Handler.vi"("error in (no error)"=w2540) -> ("error out"=w2539:errorcluster)  [unwired: 4 in, 4 out]
      }
      frame "ErrorCheck" {
        n1069 = call <extravilib>:"Write.vi"("element"=w2550) -> ("channel"=w2549:T46)  [unwired: 8 in, 2 out]
        n1070 = call <extravilib>:"Read.vi"("channel"=w2548) -> ("element"=w2551:errorcluster)  [unwired: 1 in, 1 out]
        n1071 = Merge Errors(w2551, w2550) -> (w2544:errorcluster)
        n1072 = Unbundle By Name(w2543) -> ("AfterErrorCheck"=w2553:string)
        n1073 = flat-sequence {
          tunnel: w2553 -> [w2558]
          tunnel: "Shutdown" ("t") -> [w2557]
          tunnel: w2544 -> [w2555]
          tunnel: [w2556] -> w2554
          tunnel: [w2562] -> w2545
          tunnel: w2554 -> [w2562]
          tunnel: w2543 -> [w2561]
          tunnel: [w2559] -> w2547
          frame #0 {
            n1074 = Select(t=w2557, s=w2555, f=w2558) -> (s? t:f=w2556:string)
          }
          frame #1 {
            n1075 = Bundle By Name(cluster=w2561, "AfterErrorCheck"="Shutdown") -> (w2559:T15)
          }
        }
      }
      frame "Idle", Default {
        n1076 = call <extravilib>:"Read.vi"("channel"=w2582) -> ("element"=w2580:T26)  [unwired: 8 in, 2 out]
        n1077 = Unbundle By Name(w2580) -> ("Physical Settings"=w2579:T38, "GenerationSettings"=w2578:T39, "Channel Names"=w2577:string, "FileSettings"=w2563:T36)
        n1078 = call <extravilib>:"Read.vi"("channel"=w2581) -> ("element"=w2573:T37)  [unwired: 8 in, 2 out]
        n1079 = Unbundle By Name(w2573) -> ("PreviousInfo"=w2565:T60, "SyncStart"=w2566:bool, "Leader"=w2567:bool, "Started?"=w2568:bool, "AfterErrorCheck"=w2569:string, "rendezvous ref"=w2570:T7, "AcStarted"=w2571:bool)
        n1080 = Bundle By Name(cluster=w2564, "Physical Settings"=w2579, "GenerationSettings"=w2578, "Channel Names"=w2577, "FileSettings"=w2563) -> (w2576:T16)
        n1081 = Bundle By Name(cluster=w2574, "PreviousInfo"=w2565, "SyncStart"=w2566, "Leader"=w2567, "Started?"=w2568, "AfterErrorCheck"=w2569, "rendezvous ref"=w2570, "AcStarted"=w2571) -> (w2572:T15)
      }
    }
    n1082 = call <extravilib>:"Read.vi"("channel"=w2268) -> ("element"=w2269:bool)  [unwired: 1 in, 1 out]
  }
  n1083 = while {
    tunnel: w105 -> [w2585]
    tunnel: w16 -> [w2587]
    stop <- w2586 stop-if-true
    n1084 = call <extravilib>:"Read.vi"("channel"=w2585) -> ("element"=w2584:T18)  [unwired: 6 in, 4 out]
    n1085 = call "CameraDisplay.vi"("Image Display 2"=w2584) -> ()  [unwired: 10 in, 1 out]
    n1086 = call <extravilib>:"Read.vi"("channel"=w2587) -> ("element"=w2586:bool)  [unwired: 1 in, 1 out]
  }
  n1087 = while {
    tunnel: w4 -> [w2614]
    tunnel: w16 -> [w2612]
    tunnel: w3 -> [w2609]
    shift-right: [w2588] -> _
    shift-left: FALSE ("DoneReset") -> [w2607]
    stop <- w2613 stop-if-true
    # "Plotting"
    n1088 = call <extravilib>:"Read.vi"("channel"=w2614) -> ("remaining"=→"Plot Overflow":i32, "element"=w2603:waveform(dbl)[])  [unwired: 8 in, 1 out]
    n1089 = call <extravilib>:"Read.vi"("channel"=w2609) -> ("element"=w2608:bool)  [unwired: 1 in, 1 out]
    n1090 = control-ref of="Plot 1 Channels"() -> (w2598:refnum<vi>)
    n1091 = control-ref of="Plot 2 Channels"() -> (w2597:refnum<vi>)
    n1092 = control-ref of="Plot 4 Channels"() -> (w2595:refnum<vi>)
    n1093 = control-ref of="Plot 3 Channels"() -> (w2596:refnum<vi>)
    n1094 = Or(x=w2607, y=w2608) -> (x .or. y?=w2594:bool)
    n1095 = call "FilterWaveformByPlot.vi"("ListBox in"=w2597, "element"=w2603) -> ("error IO"=w2600:errorcluster, "Array"=w2604:waveform(dbl)[])  [unwired: 8 in]
    n1096 = call "FilterWaveformByPlot.vi"("ListBox in"=w2598, "element"=w2603) -> ("error IO"=w2599:errorcluster, "Array"=w2611:waveform(dbl)[])  [unwired: 8 in]
    n1097 = call "FilterWaveformByPlot.vi"("ListBox in"=w2596, "element"=w2603) -> ("error IO"=w2601:errorcluster, "Array"=w2606:waveform(dbl)[])  [unwired: 8 in]
    n1098 = call "FilterWaveformByPlot.vi"("ListBox in"=w2595, "element"=w2603) -> ("error IO"=w2602:errorcluster, "Array"=w2605:waveform(dbl)[])  [unwired: 8 in]
    n1099 = call "Plot2.vi"("error constant"=w2600, "Reset"=w2594, "Array 2"=w2604) -> ("DoneReset"=w2592:bool)  [unwired: 6 in, 2 out]
    n1100 = call "Plot4.vi"("error constant"=w2602, "Reset"=w2594, "Array 2"=w2605) -> ("DoneReset"=w2590:bool)  [unwired: 6 in, 2 out]
    n1101 = call "Plot1.vi"("error constant"=w2599, "Reset"=w2594, "Array 2"=w2611) -> ("DoneReset"=w2593:bool)  [unwired: 6 in, 2 out]
    n1102 = call "Plot3.vi"("error constant"=w2601, "Reset"=w2594, "Array 2"=w2606) -> ("DoneReset"=w2591:bool)  [unwired: 6 in, 2 out]
    n1103 = Build Array(w2593, w2592, w2591, w2590) -> (w2589:bool[])
    n1104 = And Array Elements(Boolean array=w2589) -> (logical AND=w2588:bool)
    n1105 = call <extravilib>:"Read.vi"("channel"=w2612) -> ("element"=w2613:bool)  [unwired: 1 in, 1 out]
  }
  n1106 = while {
    tunnel: w16 -> [w2644]
    stop <- w2645 stop-if-true
    # "File Management"
    n1107 = while {
      tunnel: ["First Video File"] -> w2622
      tunnel: ["Combine Split Videos"] -> w2631
      tunnel: ["Save Path"] -> w2630
      tunnel: ["Save Name"] -> w2617
      tunnel: ["Same as previous"] -> w2629
      tunnel: ["Quality"] -> w2628
      tunnel: ["AVI FPS"] -> w2624
      tunnel: ["Current Image Type"] -> w2627
      tunnel: ["Timing File"] -> w2626
      tunnel: ["Same as acquisition"] -> w2625
      stop <- "Start Button" stop-if-true
      n1108 = Wait (ms)(milliseconds to wait=u32 1000) -> ()  [unwired: 1 out]
    }
    n1109 = Strip Path(path=w2622) -> (name=w2621:string)  [unwired: 1 out]
    n1110 = Concatenate Strings(w2617, "_000" ("string"), ".avi" ("string")) -> (w2616:string)
    n1111 = case shown="False" w2625 {
      tunnel: w2626 -> [_ w2660]
      tunnel: w2624 -> [w2646 _]
      tunnel: [w2646 w2647] -> w2623
      frame False {
      }
      frame True {
        n1112 = call-poly <vilib>:"Read Delimited Spreadsheet.vi"("file path (dialog if empty)"=w2660, "number of rows (all:-1)"=3, "delimiter (\\t)"="," ("delimiter (\\t)")) -> ("all rows"=w2653:dbl[][])  [unwired: 7 in, 5 out]
        n1113 = Index Array(array=w2653, index (row)=1) -> (element=w2655:dbl[])  [unwired: 1 in]
        n1114 = Index Array(array=w2653, index (row)=2) -> (element=w2652:dbl[])  [unwired: 1 in]
        n1115 = Index Array(array=w2652, index=1) -> (element=w2650:dbl)
        n1116 = Index Array(array=w2655, index=1) -> (element=w2649:dbl)
        n1117 = Subtract(x=w2650, y=w2649) -> (x-y=w2648:dbl)
        n1118 = Reciprocal(x=w2648) -> (1/x=w2647:dbl)
      }
    }
    n1119 = Search and Replace String(input string=w2621, search string=".tdms", replace string=".avi" ("replace string (\"\")")) -> (result string=w2618:string)  [unwired: 5 in, 3 out]
    n1120 = Select(t=w2618, s=w2629, f=w2616) -> (s? t:f=w2615:string)
    n1121 = call "IMAQ Create"("Border Size"=0, "Image Name"="TDMS to AVI", "Image Type"=w2627) -> ("New Image"=w2640:T18)  [unwired: 1 in, 2 out]
    n1122 = while {
      tunnel: [w2746] -> w2635
      shift-right: [w2744] -> _
      shift-left: w2622 -> [w2745]
      i -> [w2746]
      stop <- w2748 stop-if-true
      n1123 = Equal To 0?(x=w2746) -> (x = 0?=w2747:bool)
      n1124 = case shown="False" w2747 {
        tunnel: [w2750 w2752] -> w2744
        tunnel: w2745 -> [w2751 w2752]
        frame False {
          n1125 = call "Increment Filename.vi"("Path In"=w2751) -> ("Incremented Path Out"=w2750:path)  [unwired: 10 in]
        }
        frame True {
        }
      }
      n1126 = call <vilib>:"Check if File or Folder Exists.vi"("path"=w2744) -> ("file or folder exists?"=w2749:bool)  [unwired: 8 in, 2 out]
      n1127 = Not(x=w2749) -> (.not. x?=w2748:bool)
    }
    n1128 = Build Path(base path=w2630, name or relative path=w2615) -> (appended path=w2636:path)
    n1129 = for {
      N: w2635 -> [w2683]
      tunnel: w2640 -> [w2706]
      tunnel: w2631 -> [w2687]
      tunnel: w2628 -> [w2702]
      tunnel: w2623 -> [w2701]
      shift-right: [w2691] -> _
      shift-left: _ -> [w2696]
      tunnel: w2640 -> [w2692]
      shift-right: [w2686] -> _
      shift-left: w2622 -> [w2688]
      tunnel: [w2682] -> w2634
      shift-right: [w2681] -> _
      shift-left: w2636 -> [w2690]
      tunnel: [w2677] -> w2632
      i -> [w2682]
      stop <- w2677 stop-if-true
      n1130 = Equal To 0?(x=w2682) -> (x = 0?=w2689:bool)
      n1131 = case shown="False" w2689 {
        tunnel: [w2712 w2713] -> w2686
        tunnel: w2688 -> [w2711 w2713]
        frame False {
          n1132 = call "Increment Filename.vi"("Path In"=w2711) -> ("Incremented Path Out"=w2712:path)  [unwired: 10 in]
        }
        frame True {
        }
      }
      n1133 = Not(x=w2687) -> (.not. x?=w2704:bool)
      n1134 = And(x=w2687, y=w2689) -> (x .and. y?=w2705:bool)
      n1135 = call-poly "TDMS File Initialization (Poly).vi"("Image In"=w2706, "File Path"=w2686) -> ("Number of Images in TDMS File"=w2697:u32, "Read Settings"=w2700:T62, "TDMS Refnum Out"=w2699:refnum<k34>)  [unwired: 6 in, 1 out]
      n1136 = Or(x=w2704, y=w2705) -> (x .or. y?=w2703:bool)
      n1137 = case shown="True" w2703 {
        tunnel: w2687 -> [_ _]
        tunnel: w2702 -> [_ w2735]
        tunnel: w2701 -> [_ w2733]
        tunnel: [w2728 w2732] -> w2698
        tunnel: w2696 -> [w2728 _]
        tunnel: w2689 -> [_ w2731]
        tunnel: w2690 -> [w2727 w2730]
        tunnel: [w2727 w2729] -> w2681
        frame False {
        }
        frame True {
          n1138 = case shown="False" w2731 {
            tunnel: w2730 -> [w2737 w2738]
            tunnel: [w2736 w2738] -> w2729
            frame False {
              n1139 = call "Increment Filename.vi"("Path In"=w2737) -> ("Incremented Path Out"=w2736:path)  [unwired: 10 in]
            }
            frame True {
            }
          }
          n1140 = property on="Codec" class="Ring (strict)"() -> ("RingText.Text"=w2734:string)  [unwired: 2 in, 2 out]
          n1141 = call "IMAQ AVI2 Create"("Quality"=w2735, "Codec"=w2734, "Frames Per Second"=w2733, "AVI Path"=w2729) -> ("AVI Refnum"=w2732:T19)  [unwired: 6 in, 1 out]
        }
      }
      n1142 = for {
        N: w2697 -> [w2721]
        tunnel: w2699 -> [w2726]
        tunnel: w2700 -> [w2725]
        tunnel: w2698 -> [w2724]
        tunnel: [w2716] -> w2694
        tunnel: [w2722] -> w2691
        tunnel: [w2719] -> w2695
        tunnel: [w2714] -> w2677
        i -> [w2717]
        stop <- w2714 stop-if-true
        n1143 = call "TDMS Read File.vi"("Image Index"=w2717, "Read Settings"=w2725, "TDMS Refnum In"=w2726) -> ("error out"=w2723:errorcluster, "Image"=w2718:T18, "TDMS Refnum Out"=w2719:refnum<k34>)  [unwired: 5 in, 1 out]
        n1144 = Divide(x=w2717, y=w2721) -> (x/y=→"File Percent Done":dbl)
        n1145 = call "IMAQ AVI2 Write Frame"("error in (no error)"=w2723, "Image"=w2718, "AVI Refnum"=w2724) -> ("error out"=w2716:errorcluster, "AVI Refnum (duplicate)"=w2722:T19)  [unwired: 6 in, 1 out]
        n1146 = Or(x=w2716, y="Stop Conversion") -> (x .or. y?=w2714:bool)
      }
      n1147 = Equal?(x=w2683, y=w2682) -> (x = y?=w2685:bool)
      n1148 = Not(x=w2685) -> (.not. x?=w2684:bool)
      n1149 = Not(x=w2677) -> (.not. x?=w2678:bool)
      n1150 = TDMS Advanced Close(8:w2694, 11:w2695) -> (0:w2693:errorcluster)  [unwired: 2 in, 1 out]
      n1151 = Or(x=w2684, y=w2687) -> (x .or. y?=w2680:bool)
      n1152 = Or(x=w2678, y=w2680) -> (x .or. y?=w2679:bool)
      n1153 = case shown="False" w2679 {
        tunnel: w2693 -> [w2710 _]
        tunnel: w2692 -> [w2709 _]
        tunnel: w2691 -> [w2708 _]
        frame False {
          n1154 = call "IMAQ Dispose"("Image"=w2709, "error in (no error)"=w2710) -> ("error out"=w2707:errorcluster)  [unwired: 4 in]
          n1155 = call "IMAQ AVI2 Close"("error in (no error)"=w2707, "AVI Refnum"=w2708) -> ()  [unwired: 9 in, 1 out]
        }
        frame True {
        }
      }
      n1156 = property on="Files Complete" class="Slide (strict)"("Value"=w2682) -> ()  [unwired: 2 in, 2 out]
      n1157 = property on="Files Complete" class="Slide (strict)"("Scale.Maximum"=w2683) -> ()  [unwired: 2 in, 2 out]
    }
    n1158 = Less Than 0?(x=w2635) -> (x < 0?=w2643:bool)
    n1159 = case shown="False" w2643 {
      frame False {
      }
      frame True {
        n1160 = xnode "Error Ring"() -> ()  [unwired: 1 out]
      }
    }
    n1161 = call <extravilib>:"Read.vi"("channel"=w2644) -> ("element"=w2645:bool)  [unwired: 1 in, 1 out]
    n1162 = Wait (ms)(milliseconds to wait=u32 10000) -> ()  [unwired: 1 out]
    n1163 = case shown="True" w2632 {
      tunnel: w2634 -> [w2662 _]
      tunnel: [w2661 0] -> w2633
      frame False {
        n1164 = Increment(x=w2662) -> (x+1=w2661:i32)
      }
      frame True {
        n1165 = property on="File Percent Done" class="Slide (strict)"("Value"=0.0 ("File Percent Done")) -> ()  [unwired: 2 in, 2 out]
      }
    }
    n1166 = property on="Files Complete" class="Slide (strict)"("Value"=w2633) -> ()  [unwired: 2 in, 2 out]
  }
